vi "tvac_gui_chamber_workingcopy.vi"() -> ()   [LabVIEW 2017]
uses:
  Zones.ctl
  <vilib>/httpClient/ClientHandle.ctl
  msg7171_linux.llb/send single message.vi
  <vilib>/httpClient/POSTBuffer.vi
  <vilib>/Utility/file.llb/Read Delimited Spreadsheet (string).vi
  <vilib>/httpClient/LabVIEWHTTPClient.lvlib
panel:
  in  "tprofilesheet":string[][](array[string])
  in  "ThermalProfileCluster":T1
  out "body 2":string
  out "body":string
  in  "Custom Graph Selector":i32
  in  "exit":bool
  in  "AlarmColor":u32(colorbox)
  in  "Alarm String":string
  in  "Plot Color":u32(colorbox)=16860
  in  "Temperature":dbl format="%#_13g"
  in  "TC Label":string
  in  "Graph ON/OFF":u32(colorbox)=4250624
  in  "index (col)":i32
  in  "index (row)":i32
  out "working array":bool[](array[boolean])
  in  "Local Debug":bool
  in  "Tab Control":T2(tab)
  in  "Log/Linear Y-Axis":u16(ring) items=["Linear", "Log"]
  in  "Total Time":dbl
  in  "Set Time TC Graph":bool
  in  "Graphing Selection":u16(ring) items=["User Selection", "Graph All Thermocouples", "Clear Graph"]
  in  "Time Scale":u16(ring) items=["Minutes", "Hours", "Seconds"]
  out "Waveform Chart":waveform(dbl)[](graph)
  out "Thermocouples":T3(array[cluster])
  in  "Log/Linear Y-Axis 6":u16(ring) items=["Linear", "Log"]
  in  "Log/Linear Y-Axis 5":u16(ring) items=["Linear", "Log"]
  in  "Log/Linear Y-Axis 3":u16(ring) items=["Linear", "Log"]
  in  "Log/Linear Y-Axis 2":u16(ring) items=["Linear", "Log"]
  in  "Total Time 6":dbl
  in  "Set Time TC Graph 6":bool
  in  "Time Scale 6":u16(ring) items=["Minutes", "Hours", "Seconds"]
  in  "Total Time 5":dbl
  in  "Set Time TC Graph 5":bool
  in  "Time Scale 5":u16(ring) items=["Minutes", "Hours", "Seconds"]
  in  "Total Time 4":dbl
  in  "Set Time TC Graph 4":bool
  in  "Time Scale 4":u16(ring) items=["Minutes", "Hours", "Seconds"]
  in  "Total Time 3":dbl
  in  "Set Time TC Graph 3":bool
  in  "Time Scale 3":u16(ring) items=["Minutes", "Hours", "Seconds"]
  in  "Total Time 2":dbl
  in  "Set Time TC Graph 2":bool
  in  "Time Scale 2":u16(ring) items=["Minutes", "Hours", "Seconds"]
  in  "Log/Linear Y-Axis 1":u16(ring) items=["Linear", "Log"]
  in  "Total Time 1":dbl
  in  "Set Time TC Graph 1":bool
  in  "Time Scale 1":u16(ring) items=["Minutes", "Hours", "Seconds"]
  in  "Custom Chart 2 Selection":i32[](listbox)=[0]
  in  "Custom Chart 1 Selection":i32[](listbox)=[0]
  out "Custom Chart 1":waveform(dbl)[](graph)
  in  "Custom Chart 3 Selection":i32[](listbox)=[0]
  in  "Custom Chart 4 Selection":i32[](listbox)=[0]
  in  "Custom Chart 5 Selection":i32[](listbox)=[0]
  in  "Custom Chart 6 Selection":i32[](listbox)=[0]
  out "Custom Chart 2":waveform(dbl)[](graph)
  out "Custom Chart 3":waveform(dbl)[](graph)
  out "Custom Chart 4":waveform(dbl)[](graph)
  out "Custom Chart 5":waveform(dbl)[](graph)
  out "Custom Chart 6":waveform(dbl)[](graph)
  in  "Log/Linear Y-Axis 4":u16(ring) items=["Linear", "Log"]
  in  "Import Profile":bool
  out "Thermal Profile":dbl[](graph)
  out "Thermal Profile Event Status":string
  in  "CreateTProfile":T4(tab)
  in  "ZoneSetup":T5={"Number of Set points"=0.0, "Zone Selection"=[8], "Initiate Setup"=FALSE, "Thermal Profile Name"=""}
  in  "RampSoakTimes":cluster{"RampSoakTimes":dbl[][]}
  in  "Zone 1":T6={"Zone Thermocouples"=[0], "Temperature Calculation"=0, "Thermocouples Selected"="", "Temperature Goal"=[], "Max Allowable Temp"="", "Min Allowable Temp"=""} {"Temperature Calculation" items=["Average", "Minimum", "Maximum"]}
  in  "Zone 2":T6={"Zone Thermocouples"=[0], "Temperature Calculation"=0, "Thermocouples Selected"="", "Temperature Goal"=[], "Max Allowable Temp"="", "Min Allowable Temp"=""} {"Temperature Calculation" items=["Average", "Minimum", "Maximum"]}
  in  "Zone 3":T6={"Zone Thermocouples"=[0], "Temperature Calculation"=0, "Thermocouples Selected"="", "Temperature Goal"=[], "Max Allowable Temp"="", "Min Allowable Temp"=""} {"Temperature Calculation" items=["Average", "Minimum", "Maximum"]}
  in  "Zone 4":T6={"Zone Thermocouples"=[0], "Temperature Calculation"=0, "Thermocouples Selected"="", "Temperature Goal"=[], "Max Allowable Temp"="", "Min Allowable Temp"=""} {"Temperature Calculation" items=["Average", "Minimum", "Maximum"]}
  in  "Zone 5":T6={"Zone Thermocouples"=[0], "Temperature Calculation"=0, "Thermocouples Selected"="", "Temperature Goal"=[], "Max Allowable Temp"="", "Min Allowable Temp"=""} {"Temperature Calculation" items=["Average", "Minimum", "Maximum"]}
  in  "Zone 6":T6={"Zone Thermocouples"=[0], "Temperature Calculation"=0, "Thermocouples Selected"="", "Temperature Goal"=[], "Max Allowable Temp"="", "Min Allowable Temp"=""} {"Temperature Calculation" items=["Average", "Minimum", "Maximum"]}
  in  "Zone 7":T6={"Zone Thermocouples"=[0], "Temperature Calculation"=0, "Thermocouples Selected"="", "Temperature Goal"=[], "Max Allowable Temp"="", "Min Allowable Temp"=""} {"Temperature Calculation" items=["Average", "Minimum", "Maximum"]}
  in  "Zone 8":T6={"Zone Thermocouples"=[0], "Temperature Calculation"=0, "Thermocouples Selected"="", "Temperature Goal"=[], "Max Allowable Temp"="", "Min Allowable Temp"=""} {"Temperature Calculation" items=["Average", "Minimum", "Maximum"]}
  in  "Zone 9":T6={"Zone Thermocouples"=[0], "Temperature Calculation"=0, "Thermocouples Selected"="", "Temperature Goal"=[], "Max Allowable Temp"="", "Min Allowable Temp"=""} {"Temperature Calculation" items=["Average", "Minimum", "Maximum"]}
  in  "Save as CSV":bool
  in  "Load Into Database":bool
  in  "Compile Profile":bool
  in  "Run Profile":bool
  in  "Resume Profile":bool
  in  "Stop Profile":bool
  in  "Pause Profile":bool
  in  "Hold Profile":bool
  in  "Path":path
  in  "Tab Control 2":enum32{"Current", "History"}(tab)
  in  "Current Errors (click to clear)":i32(listbox)
  in  "Error History":i32(listbox)
  in  "TCs On":bool=TRUE
  in  "Pressure On":bool=TRUE
  in  "MCC On":bool=TRUE
  in  "ZoneTemps On":bool=TRUE
  in  "Compressor On":bool
  in  "Generate Error":bool
  out "errortrue":bool
  # "Set Pt #"
  # "Ramp Time (s)"
  # "Soak Time (s)"
  # "Set Pt #"
  # "Goal Temp (K)"
  # "Set Pt #"
  # "Goal Temp (K)"
  # "Set Pt #"
  # "Goal Temp (K)"
  # "Set Pt #"
  # "Goal Temp (K)"
  # "Set Pt #"
  # "Goal Temp (K)"
  # "Set Pt #"
  # "Goal Temp (K)"
  # "Set Pt #"
  # "Goal Temp (K)"
  # "Set Pt #"
  # "Goal Temp (K)"
  # "Set Pt #"
  # "Goal Temp (K)"
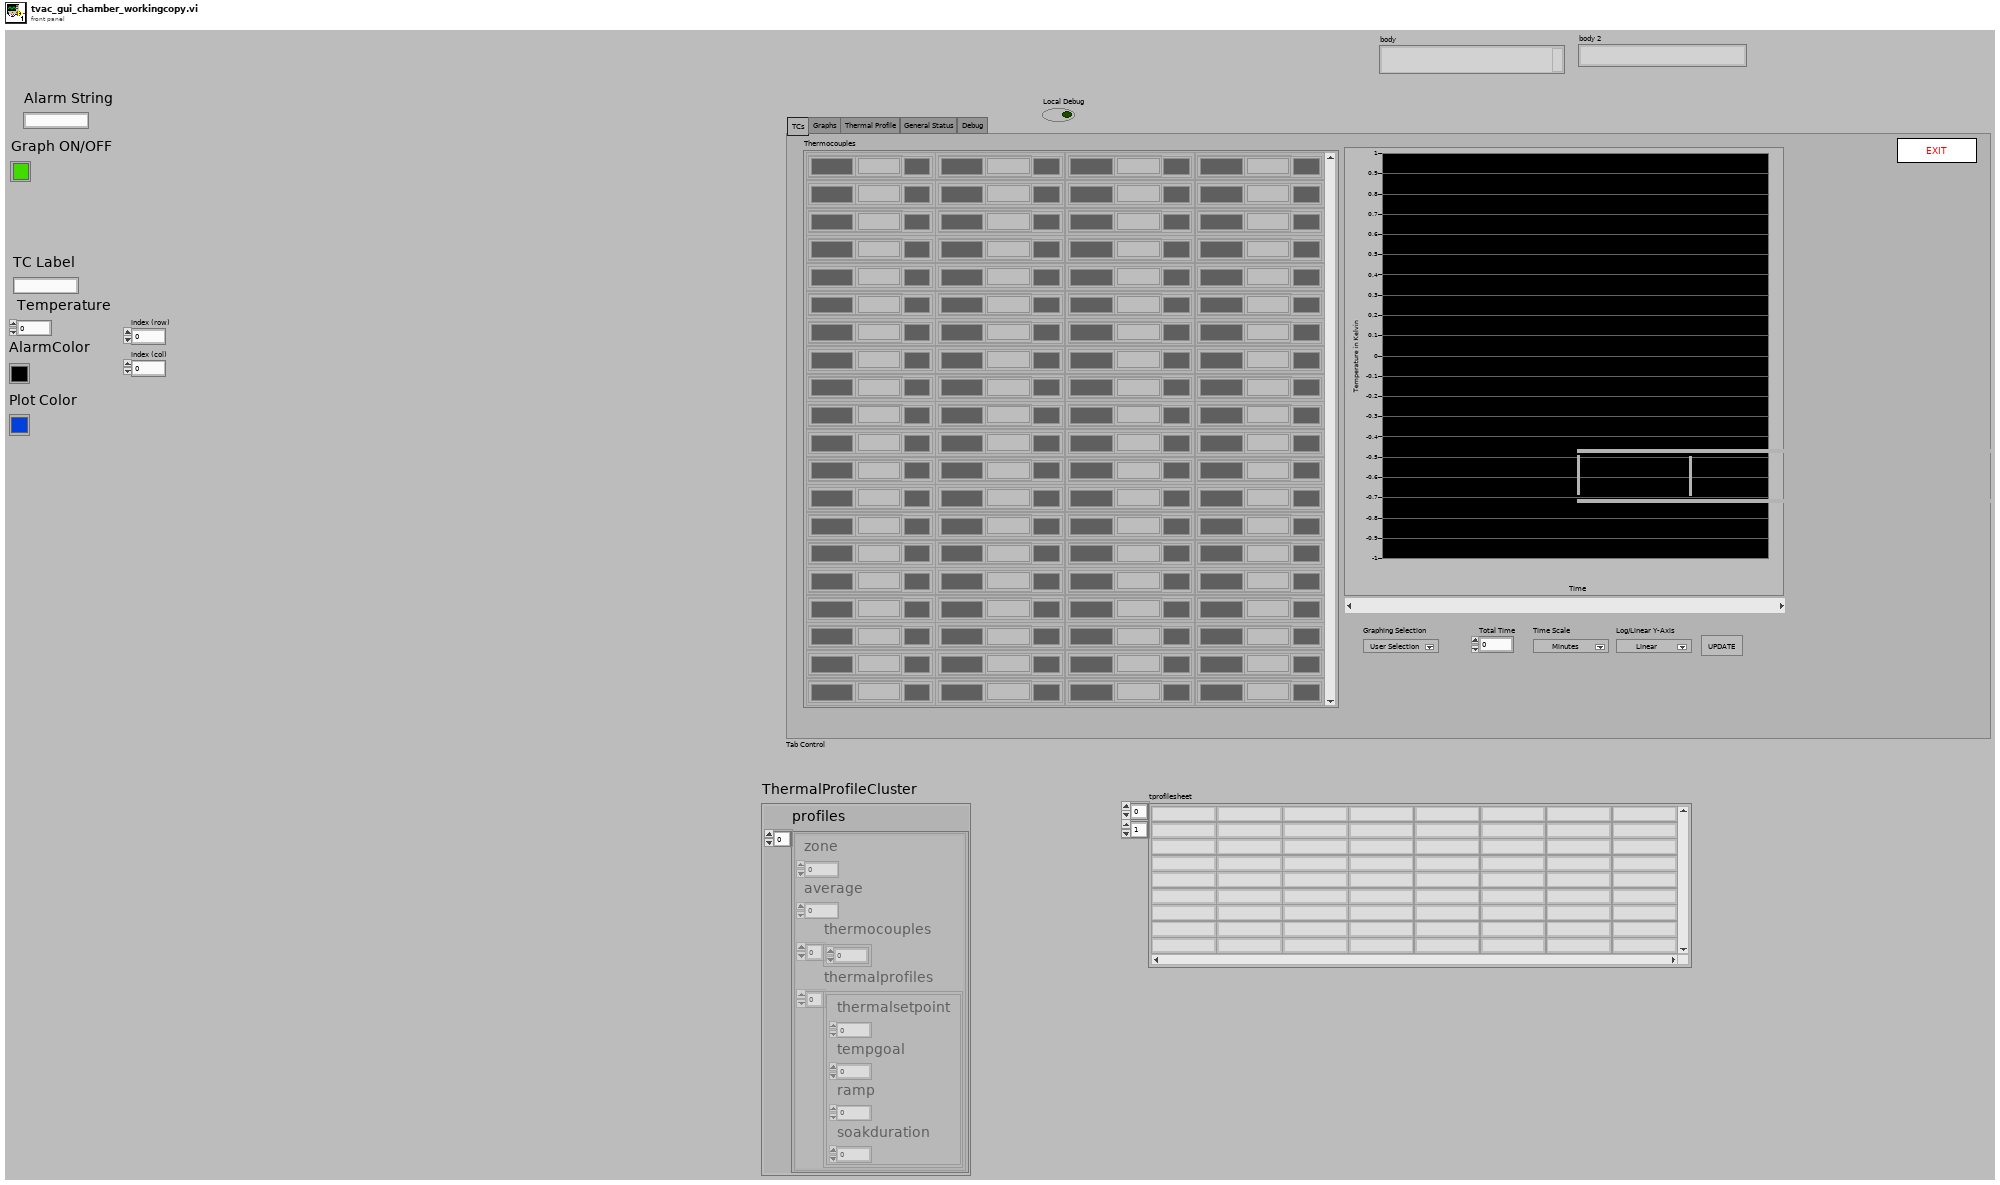
[diagram p1: front panel]
types:
  T1 = cluster{"profiles":cluster{"zone":i32, "average":i32, "thermocouples":i32[], "thermalprofiles":cluster{"thermalsetpoint":i32, "tempgoal":i32, "ramp":i32, "soakduration":i32}[]}[]}
  T2 = enum32{"TCs", "Graphs", "Thermal Profile", "General Status", "Debug"}
  T3 = cluster{"TC Label":string, "Alarm Status":string, "Alarm Color":u32, "Temperature":string, "PlotColor":u32, "Graph On/Off":u32}[][]
  T4 = enum32{"Setup", "Setup 2", "Zone 1", "Zone 2", "Zone 3", "Zone 4", "Zone 5", "Zone 6", "Zone 7", "Zone 8", "Zone 9", "Preview Profile"}
  T5 = cluster{"Number of Set points":dbl, "Zone Selection":i32[], "Initiate Setup":bool, "Thermal Profile Name":string}
  T6 = typedef "Zones.ctl" = cluster{"Zone Thermocouples":i32[], "Temperature Calculation":u16, "Thermocouples Selected":string, "Temperature Goal":dbl[][], "Max Allowable Temp":string, "Min Allowable Temp":string}
  T7 = cluster{"thermocouple":i32, "time":dbl, "temp":dbl, "working":bool, "alarm":i32}[]
  T8 = cluster{"Cp Stage 1 Temp":dbl[], "Cp Stage 2 Temp":dbl[]}
  T9 = typedef "LabVIEWHTTPClient.lvlib/ClientHandle.ctl" = refnum<k1>
  T10 = cluster{"ZoneSetup":cluster{"Number of Set points":dbl, "Zone Selection":i32[], "Initiate Setup":bool, "Thermal Profile Name":string}, "go":bool, "Http session":T9, "URL prefex":string, "index (row)":i32, "index (col)":i32, "Graph ON/OFF":u32, "TC Label":string, "Temperature":dbl, "AlarmColor":u32, "Plot Color":u32, "Alarm String":string, "Thermocouples":cluster{"TC Label":string, "Alarm Status":string, "Alarm Color":u32, "Temperature":string, "PlotColor":u32, "Graph On/Off":u32}[][], "working array":bool[], "i":i32, "NumberTCs":i32, "Waveform Chart":waveform(dbl)[], "Custom Chart 1":waveform(dbl)[], "Pressure":dbl[], "numSensors":i32, "Database":dbl[], "PumpTemps":cluster{"Cp Stage 1 Temp":dbl[], "Cp Stage 2 Temp":dbl[]}, "Zones":dbl[], "Time":i32, "TCs":cluster{"thermocouple":i32, "time":dbl, "temp":dbl, "working":bool, "alarm":i32}[], "ZoneTemps":cluster{"ZoneTemps":dbl[]}, "Compressor":cluster{"CompressorTemp":dbl}, "ErrorArray":string[][], "PrevErrorArray":string[][], "tprofilesheet":string[][], "Zone 1":T6, "ThermalProfileCluster":cluster{"profiles":cluster{"zone":i32, "average":i32, "thermocouples":i32[], "thermalprofiles":cluster{"thermalsetpoint":i32, "tempgoal":i32, "ramp":i32, "soakduration":i32}[]}[]}, "ZonesSelected":bool[], "Zone 2":T6, "Zone 3":T6, "Zone 4":T6, "Zone 5":T6, "Zone 6":T6, "Zone 7":T6, "Zone 8":T6, "Zone 9":T6}
  T11 = cluster{"TC Label":string, "Alarm Status":string, "Alarm Color":u32, "Temperature":string, "PlotColor":u32, "Graph On/Off":u32}
  T12 = enum32{"TCs", "Graphs", "Thermal Profile", "General Status"}
  T13 = cluster{"zone":i32, "average":i32, "thermocouples":i32[], "thermalprofiles":cluster{"thermalsetpoint":i32, "tempgoal":i32, "ramp":i32, "soakduration":i32}[]}
  T14 = cluster{"thermalsetpoint":i32, "tempgoal":i32, "ramp":i32, "soakduration":i32}
  T15 = cluster{"DutyCycle":i32, "Stage1Temp":i32, "CryoPumpReadyState":cluster{"MotorOn":bool, "Ready":bool}, "PurgeValveState":bool, "RegenError":string, "RegenStep":string, "RoughingValveState":bool, "RoughingInterlock":cluster{"RoughingPermission":bool, "RoughingNeeded":bool, "Cryopumprunning":bool}, "Stage2Temp":i32, "Status":cluster{"PumpOn":bool, "RoughOpen":bool, "PurgeOpen":bool, "ThermocoupleGaugeOn":bool, "PowerFailureOccurred":bool}, "TcPressure":i32}
  T16 = cluster{"time":string[], "event":string[], "Thermocouple":i32[], "details":string[], "actions":string[][]}
  T17 = cluster{"CryoPressure":dbl, "ChamberPressure":dbl, "RoughingPressure":dbl}
  T18 = cluster{"time":string, "TCs":cluster{"thermocouple":i32, "time":dbl, "temp":dbl, "working":bool, "alarm":i32}[]}
  T19 = typedef "LVPositionTypeDef.ctl" = cluster{"Left":i32, "Top":i32}
  T20 = typedef "LVPoint32TypeDef.ctl" = cluster{"Horizontal":i32, "Vertical":i32}
  T21 = typedef "LVRangeTypeDef.ctl" = cluster{"Minimum":dbl, "Maximum":dbl, "Increment":dbl, "Minor Increment":dbl, "Start":dbl}
  T22 = typedef "LVRowAndColumnTypeDef.ctl" = cluster{"Row":i32, "Column":i32}
  T23 = cluster{"zone":i32, "average":i32, "thermocouples":i32[], "thermalprofiles":cluster{"thermalsetpoint":i32, "tempgoal":i32, "ramp":i32, "soakduration":i32}[]}[]
  T24 = cluster{"thermalsetpoint":i32, "tempgoal":i32, "ramp":i32, "soakduration":i32}[]
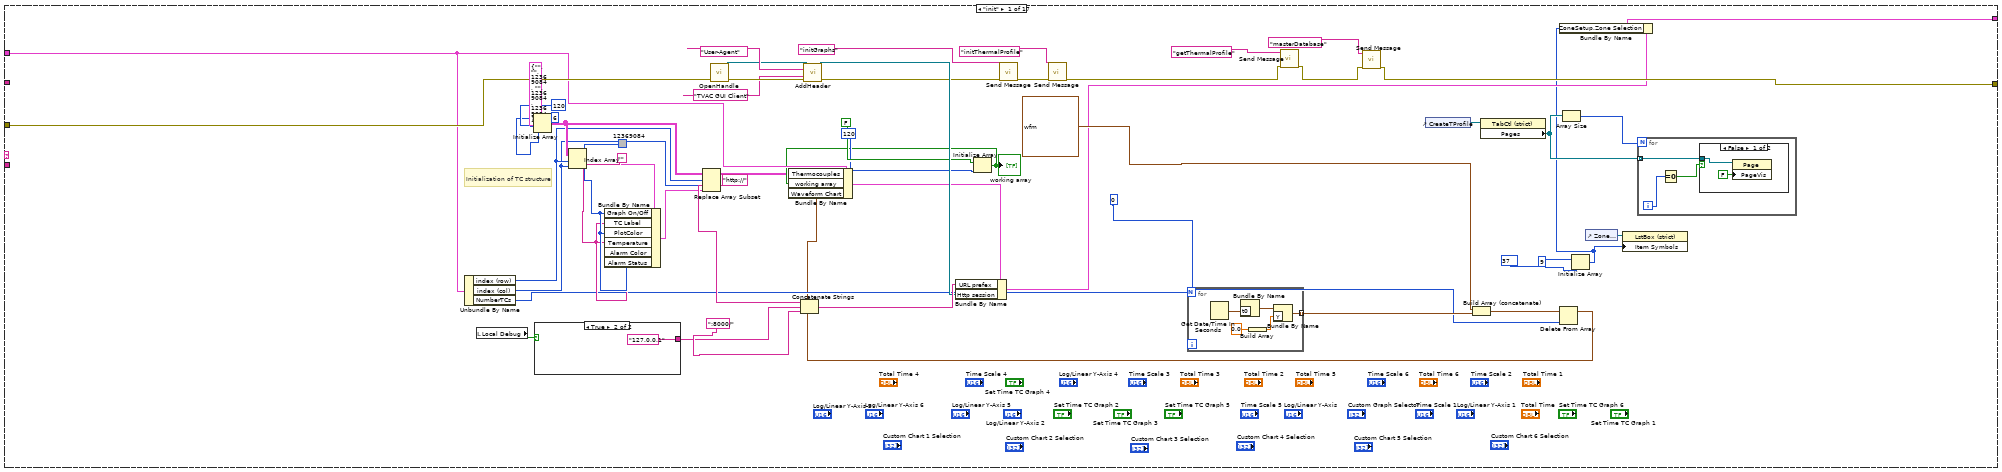
[diagram p2: hidden frame]
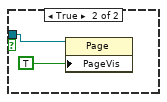
[diagram p3: hidden frame]
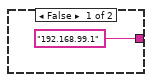
[diagram p4: hidden frame]
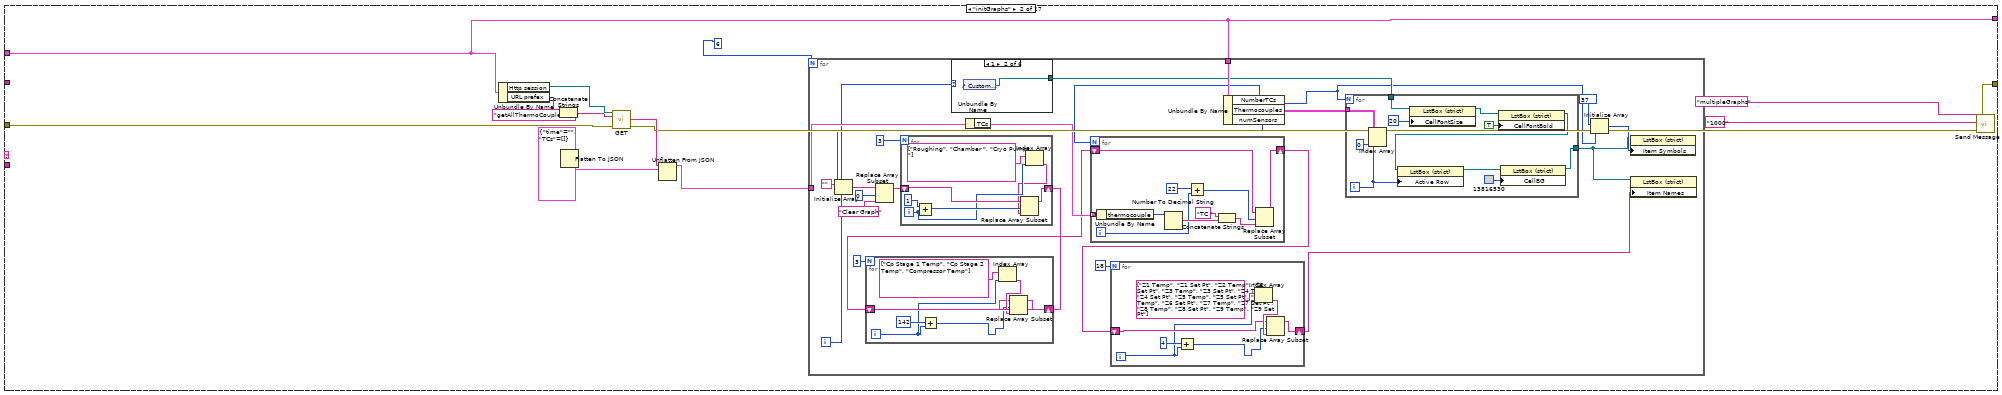
[diagram p5: hidden frame]
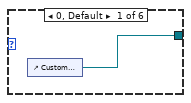
[diagram p6: hidden frame]
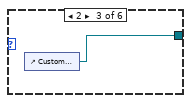
[diagram p7: hidden frame]
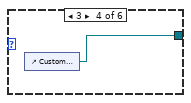
[diagram p8: hidden frame]
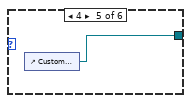
[diagram p9: hidden frame]
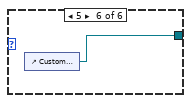
[diagram p10: hidden frame]
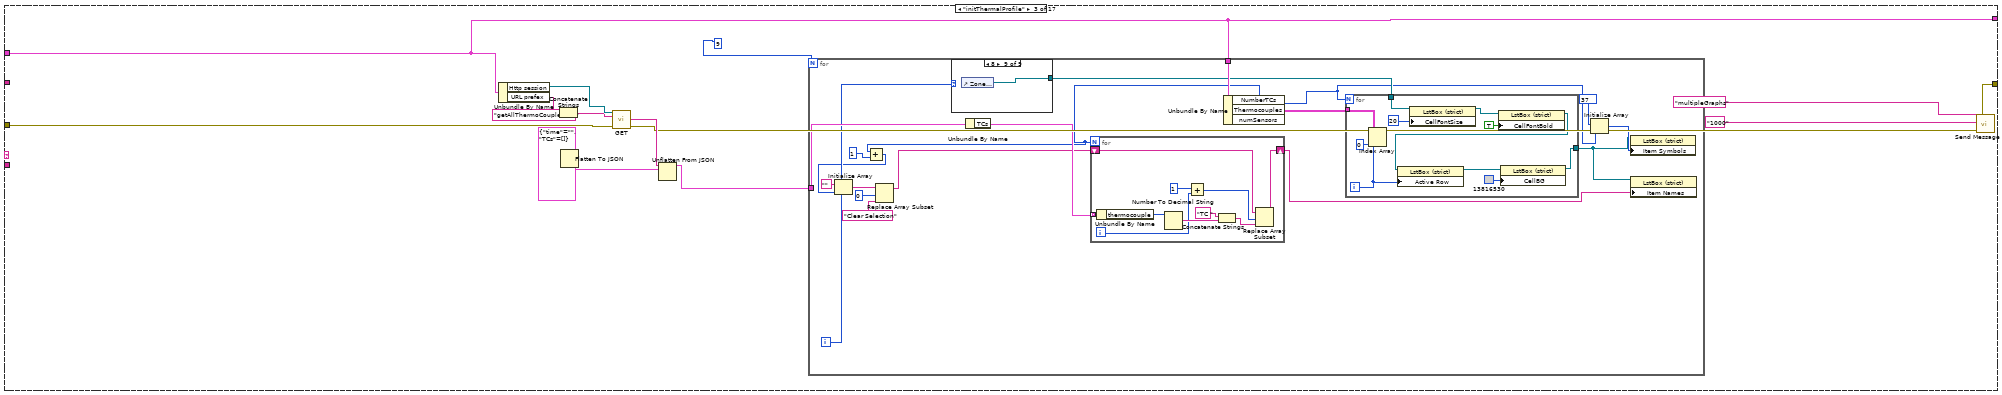
[diagram p11: hidden frame]
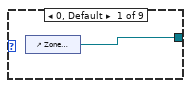
[diagram p12: hidden frame]
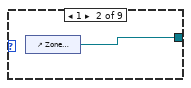
[diagram p13: hidden frame]
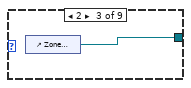
[diagram p14: hidden frame]
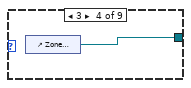
[diagram p15: hidden frame]
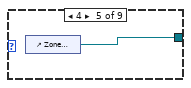
[diagram p16: hidden frame]
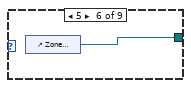
[diagram p17: hidden frame]
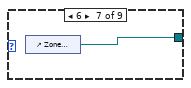
[diagram p18: hidden frame]
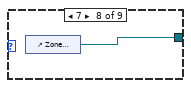
[diagram p19: hidden frame]
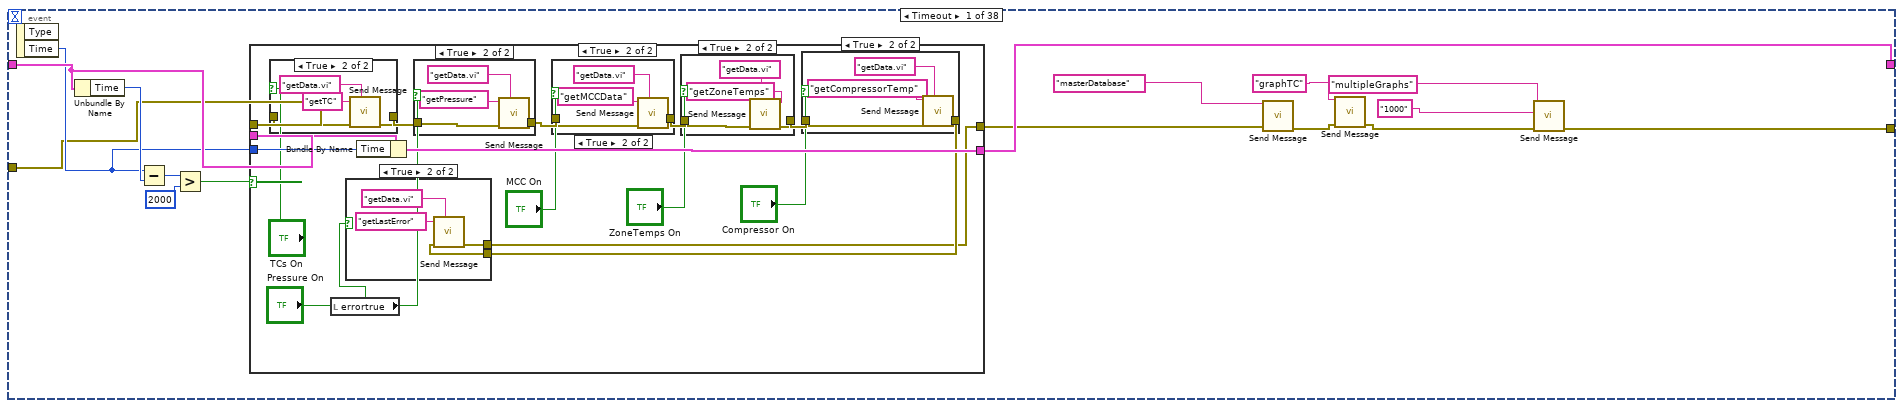
[diagram p20: hidden frame]
diagram:
  w9 = bool[] [FALSE, FALSE, FALSE, FALSE, FALSE, FALSE, FALSE, FALSE, FALSE]  # ZonesSelected
  w14 = string[][] []  # PrevErrorArray
  w15 = string[][] []  # ErrorArray
  w18 = cluster{"ZoneTemps":dbl[]} {"ZoneTemps"=[]}  # ZoneTemps
  w21 = dbl[] [24.54828257301887, 25.0, 20.035959453954195, 26.0, 28.926820041278148, 27.0, 21.321976066931608, 28.0, 29.197600688359813, 29.0, 29.117373424110085, 30.0, 21.092914485312942, 31.0, 27.791581465649088, 32.0, 24.70861457288988, 33.0]  # Zones
  w22 = T8 {"Cp Stage 1 Temp"=[0.0], "Cp Stage 2 Temp"=[0.0]}  # PumpTemps
  w23 = dbl[] [0.0, 1000.5841582194602, 1000.5841582194602, 1000.5841582194602, 0.6389895835935778, 0.7578061575842531, 1.153531014677555, 1.4572061556343079, 1.0192558642672256, 0.9245021790184325, 0.34311035179988925, 1.1970333160202968, 1.066989851322369, 0.5926593131154867, 0.7219240511326698, 1.0529790116491695, 1.4485694746891444, 0.9139060201605569, 0.7997359753068659, 0.6568795179977746, 0.8470104541419833, 1.0272585161866683, 0.6577301535824354, 0.645139941938139, 1.5235316442408067, 0.5128651184775285, 1.6421980587090137, 1.3961508335147417, 1.1242639015795428, 1.5954313466624428, 1.1919135255187876, 1.2615004458206727, 1.1320092264321664, 1.922759836270222, 1.1315561200367314, 1.4924621723754858, 0.6988771274186227, 1.069709701591943, 0.9920698240997152, 0.5395549253287656, 0.42891479657680576, 1.2794224940227927, 0.2687949632437338, 0.16127136772755854, 1.0174597006256374, 1.2079238230365172, 0.9745554383837218, 1.5348516925460962, 0.9488878852839246, 1.6634477658652282, 1.1924291951744272, 1.2231949298067308, 1.2223766746774598, 1.30664154589907, 1.2872878364107239, 0.5274250065177812, 0.7905999067114673, 1.2748974665085449, 1.216972941585413, 0.959115576325391, 0.5743502840762814, 0.8219540421676025, 0.613053899308251, 1.3785560870413707, 1.034117232127813, 1.1237698659753859, 1.4495548642149667, 0.6967905980938514, 0.6224497255665377, 1.6551326273040576, 1.2103048396824558, 0.6078721016951973, 1.3790669246280296, 0.5454332940871525, 1.5318777012492035, 1.2496539590411258, 0.9145395304446965, 1.3855381787793546, 1.0857600342029163, 1.3185833631438346, 0.9769688683142593, 1.026663691242448, 0.6744610422623843, 1.1965175398567691, 0.4847084945450119, 0.6435799980029115, 0.8079659363810663, 0.9130053929540112, 0.5271098423006861, 0.8088111736464799, 1.1455315536576556, 1.139809531926708, 1.5840192673434794, 1.0296748968089129, 1.7370669751200136, 1.3715484550405317, 0.3362063953932494, 1.0385868418202253, 1.4947740276021626, 1.0393600693910505, 0.8870410800672984, 1.2470388696569872, 0.9846724980375481, 0.9952471377109308, 1.0807485178906029, 1.1016630607035562, 1.3301039036808464, 0.8856852816151205, 0.4719509873120426, 0.5191430277856135, 0.12135113366044793, 0.4230478635224125, 1.1140562049976255, 1.5484968368781251, 1.1999891199114734, 1.8721302183420216, 1.071489235222563, 0.6260864330445979, 1.0305668002030492, 1.0223711899566386, 0.7842533472819472, 1.7301290335750898, 1.318694748426881, 0.6978662965493679]  # Database
  w25 = dbl[] [0.0, 0.0, 0.0]  # Pressure
  w45 = ""  # URL prefex
  w46 = T9 refnum  # Http session
  w47 = TRUE  # go
  n1 = call "Register Module.vi"() -> ("error out"=w43:errorcluster)  [unwired: 10 in, 1 out]
  n2 = call-poly "Send Message.vi"("error in (no error)"=w43, "event"="init") -> ("error out"=w42:errorcluster)  [unwired: 9 in]
  n3 = local read "Waveform Chart"() -> (w29:waveform(dbl)[])
  n4 = local read "Thermocouples"() -> (w27:T3)
  n5 = local read "Custom Chart 1"() -> (w26:waveform(dbl)[])
  n6 = Bundle("ZoneSetup"="ZoneSetup", "go"=w47, "Http session"=w46, "URL prefex"=w45, "index (row)"="index (row)", "index (col)"="index (col)", "Graph ON/OFF"="Graph ON/OFF", "TC Label"="TC Label", "Temperature"="Temperature", "AlarmColor"="AlarmColor", "Plot Color"="Plot Color", "Alarm String"="Alarm String", "Thermocouples"=w27, "working array"=bool[] [TRUE, TRUE, TRUE, TRUE, TRUE, TRUE, TRUE, TRUE, TRUE, TRUE, TRUE, TRUE, TRUE, TRUE, TRUE, TRUE, TRUE, TRUE, TRUE, TRUE, TRUE, TRUE, TRUE, TRUE, TRUE, TRUE, TRUE, TRUE, TRUE, TRUE, TRUE, TRUE, TRUE, TRUE, TRUE, TRUE, TRUE, TRUE, TRUE, TRUE, TRUE, TRUE, TRUE, TRUE, TRUE, TRUE, TRUE, TRUE, TRUE, TRUE, TRUE, TRUE, TRUE, TRUE, TRUE, TRUE, TRUE, TRUE, TRUE, TRUE, TRUE, TRUE, TRUE, TRUE, TRUE, TRUE, TRUE, TRUE, TRUE, TRUE, TRUE, TRUE, TRUE, TRUE, TRUE, TRUE, TRUE, TRUE, TRUE, TRUE, TRUE, TRUE, TRUE, TRUE, TRUE, TRUE, TRUE, TRUE, TRUE, TRUE, TRUE, TRUE, TRUE, TRUE, TRUE, TRUE, TRUE, TRUE, TRUE, TRUE, TRUE, TRUE, TRUE, TRUE, TRUE, TRUE, TRUE, TRUE, TRUE, TRUE, TRUE, TRUE, TRUE, TRUE, TRUE, TRUE, TRUE, TRUE, TRUE, TRUE], "i"=0, "NumberTCs"=120, "Waveform Chart"=w29, "Custom Chart 1"=w26, "Pressure"=w25, "numSensors"=145, "Database"=w23, "PumpTemps"=w22, "Zones"=w21, "Time"=0, "TCs"=T7 [], "ZoneTemps"=w18, "Compressor"=cluster{"CompressorTemp":dbl} {"CompressorTemp"=0.0}, "ErrorArray"=w15, "PrevErrorArray"=w14, "tprofilesheet"="tprofilesheet", "Zone 1"="Zone 1", "ThermalProfileCluster"="ThermalProfileCluster", "ZonesSelected"=w9, "Zone 2"="Zone 2", "Zone 3"="Zone 3", "Zone 4"="Zone 4", "Zone 5"="Zone 5", "Zone 6"="Zone 6", "Zone 7"="Zone 7", "Zone 8"="Zone 8", "Zone 9"="Zone 9") -> (w33:T10)  [unwired: 1 in]
  n7 = while {
    shift-left: w33 -> [w52]
    shift-right: [w49] -> _
    shift-right: [w50] -> w28
    shift-left: w42 -> [w57]
    stop <- w48 continue-if-true
    n8 = call "Get Message.vi"("error in (no error)"=w57) -> ("error out"=w55:errorcluster, "event buffer"=w56:string, "event"=w54:string, "source"=w53:string)  [unwired: 7 in]
    n9 = case shown="\"\", \"Idle\"" w54 {
      selector: w54 -> [_ _ _ _ _ _ _ _ _ _ _ _ _ _ _ _ w2622]
      tunnel: [w60 w129 w214 w282 w1761 w1860 w2299 w2381 w2394 w2403 w2437 w2439 w2451 w2464 w2484 w2620 w2624] -> w49
      tunnel: w52 -> [w83 w129 w214 w283 w1763 w1863 w2304 w2380 w2393 w2398 w2438 w2443 w2450 w2465 w2484 w2616 w2624]
      tunnel: w56 -> [_ _ _ _ _ _ _ w2378 w2383 w2414 w2429 w2442 w2448 _ w2485 _ _]
      tunnel: w55 -> [w104 w128 w213 w272 w1766 w1896 w2294 w2379 w2384 w2400 w2430 w2440 w2449 w2470 _ w2619 w2623]
      tunnel: [w68 w124 w209 w271 w1766 w1896 w2294 w2379 w2384 w2400 w2430 w2440 w2449 w2470 _ w2618 w2621] -> w51
      tunnel: w53 -> [_ _ _ _ _ _ _ _ _ _ _ _ _ _ _ _ _]
      frame "init" {
        w88 = ""
        w89 = u32 12369084 ("PlotColor")
        # "Initialization of TC structure"
        n10 = Unbundle By Name(w83) -> ("index (row)"=w91:i32, "index (col)"=w90:i32, "NumberTCs"=w80:i32)
        n11 = local read "Local Debug"() -> (w96:bool)
        n12 = Initialize Array(T11 {"TC Label"="", "Alarm Status"="", "Alarm Color"=12369084, "Temperature"="", "PlotColor"=12369084, "Graph On/Off"=12369084}, 120 ("dimension size"), 6 ("dimension size")) -> (w92:T3)
        n13 = case shown="True" w96 {
          tunnel: ["192.168.99.1" ("Address") "127.0.0.1" ("Address")] -> w97
          frame False {
          }
          frame True {
          }
        }
        n14 = Index Array(array=w92, index (row)=w91, index (col)=w90) -> (element=w87:T11)
        n15 = Bundle By Name(cluster=w87, "Graph On/Off"=w89, "TC Label"=w88, "PlotColor"=w89, "Temperature"=w88, "Alarm Color"=w89, "Alarm Status"=w88) -> (w86:T11)
        n16 = Replace Array Subset(array=w92, new element=w86, index (row)=w91, index (col)=w90) -> (w74:T3)
        n17 = call <vilib>:"OpenHandle.vi"("error in (no error)"=w104) -> ("client handle out"=w105:T9, "error out"=w108:errorcluster)  [unwired: 13 in]
        n18 = Concatenate Strings("http://" ("url"), w97, ":8000/" ("url")) -> (w101:string)
        n19 = call <vilib>:"AddHeader.vi"("client handle"=w105, "header"="User-Agent", "value"="TVAC GUI Client", "error in (no error)"=w108) -> ("client handle out"=w100:T9, "error out"=w99:errorcluster)  [unwired: 10 in]
        n20 = Initialize Array(FALSE ("Boolean"), 120 ("dimension size")) -> (w81:bool[])
        "working array" <- w81
        n21 = call-poly "Send Message.vi"("error in (no error)"=w99, "event"="initGraphs") -> ("error out"=w73:errorcluster)  [unwired: 9 in]
        n22 = call-poly "Send Message.vi"("error in (no error)"=w73, "event"="initThermalProfile") -> ("error out"=w71:errorcluster)  [unwired: 9 in]
        n23 = for {
          N: w80 -> [_]
          tunnel: [w116] -> w78 mode=indexing
          n24 = Get Date/Time In Seconds() -> (seconds since 1Jan1904=w120:timestamp)
          n25 = Bundle By Name("t0"=w120) -> (w117:waveform(dbl))  [unwired: 1 in]
          n26 = Build Array(0.0) -> (w119:dbl[])
          n27 = Bundle By Name(cluster=w117, "Y"=w119) -> (w116:waveform(dbl))
        }
        n28 = call-poly "Send Message.vi"("error in (no error)"=w71, "event"="getThermalProfile") -> ("error out"=w69:errorcluster)  [unwired: 9 in]
        n29 = call-poly "Send Message.vi"("error in (no error)"=w69, "event"="masterDatabase") -> ("error out"=w68:errorcluster)  [unwired: 9 in]
        n30 = control-ref of="CreateTProfile"() -> (w66:refnum<vi>)
        n31 = Build Array (concatenate)(waveform(dbl) {"t0"=timestamp(0 s since 1904-01-01), "dt"=1.0, "Y"=[0.0]} ("element"), w78) -> (w79:waveform(dbl)[])
        n32 = property on="Property Node" class="TabCtl (strict)"(reference=w66) -> ("Pages"=w64:refnum<vi>[])  [unwired: 1 in, 2 out]
        n33 = Delete From Array(array=w79, index=0) -> (array with subset deleted=w77:waveform(dbl)[])  [unwired: 1 in, 1 out]
        n34 = Bundle By Name(cluster=w83, "Thermocouples"=w74, "working array"=w81, "Waveform Chart"=w77) -> (w82:T10)
        n35 = Bundle By Name(cluster=w82, "URL prefex"=w101, "Http session"=w100) -> (w61:T10)
        n36 = Array Size(array=w64) -> (size(s)=w65:i32)
        n37 = Initialize Array(37, 9 ("dimension size")) -> (w58:i32[])
        n38 = Bundle By Name(cluster=w61, "ZoneSetup.Zone Selection"=w58) -> (w60:T10)
        n39 = control-ref of="Zone Selection"() -> (w59:refnum<vi>)
        n40 = property class="LstBox (strict)"(reference=w59, "Item Symbols"=w58) -> ()  [unwired: 1 in, 2 out]
        n41 = for {
          N: w65 -> [_]
          tunnel: w64 -> [w109] mode=indexing
          i -> [w111]
          n42 = Equal To 0?(x=w111) -> (x = 0?=w110:bool)
          n43 = case shown="False" w110 {
            tunnel: w109 -> [w112 w114]
            frame False {
              n44 = property on="Property Node" class="Page"(reference=w112, "PageVis"=FALSE ("Page Visible")) -> ()  [unwired: 1 in, 2 out]
            }
            frame True {
              n45 = property on="Property Node" class="Page"(reference=w114, "PageVis"=TRUE ("Page Selector Visible")) -> ()  [unwired: 1 in, 2 out]
            }
          }
        }
      }
      frame "initGraphs" {
        w130 = T18 {"time"="", "TCs"=[]} ("Cluster")
        n46 = Unbundle By Name(w129) -> ("Http session"=w136:T9, "URL prefex"=w134:string)
        n47 = Concatenate Strings(w134, "getAllThermoCoupleData" ("url")) -> (w135:string)
        n48 = Flatten To JSON(anything=w130) -> ()  [unwired: 2 in, 2 out]
        n49 = call <vilib>:"GET.vi"("client handle"=w136, "url"=w135, "error in (no error)"=w128) -> ("body"=w132:string, "error out"=w125:errorcluster)  [unwired: 9 in, 2 out]
        n50 = Unflatten From JSON(JSON string=w132, type and defaults=w130) -> (value=w131:T18)  [unwired: 5 in, 1 out]
        n51 = for {
          N: 6 ("Numeric") -> [_]
          tunnel: w131 -> [w158]
          tunnel: w129 -> [w157]
          i -> [w140]
          n52 = case shown="1" w140 {
            tunnel: [w160 w161 w162 w163 w164 w165] -> w141
            frame 0, Default {
              n53 = control-ref of="Custom Chart 1 Selection"() -> (w160:refnum<vi>)
            }
            frame 1 {
              n54 = control-ref of="Custom Chart 2 Selection"() -> (w161:refnum<vi>)
            }
            frame 2 {
              n55 = control-ref of="Custom Chart 3 Selection"() -> (w162:refnum<vi>)
            }
            frame 3 {
              n56 = control-ref of="Custom Chart 4 Selection"() -> (w163:refnum<vi>)
            }
            frame 4 {
              n57 = control-ref of="Custom Chart 5 Selection"() -> (w164:refnum<vi>)
            }
            frame 5 {
              n58 = control-ref of="Custom Chart 6 Selection"() -> (w165:refnum<vi>)
            }
          }
          n59 = Unbundle By Name(w158) -> ("TCs"=w154:T7)
          n60 = Unbundle By Name(w157) -> ("NumberTCs"=w152:i32, "Thermocouples"=w159:T3, "numSensors"=w138:i32)
          n61 = Initialize Array("", w138) -> (w150:string[])
          n62 = Replace Array Subset(array=w150, new element="Clear Graph" ("new element/subarray"), index=0) -> (w147:string[])
          n63 = for {
            N: 3 -> [_]
            shift-right: [w185] -> w145
            shift-left: w147 -> [w186]
            i -> [w181]
            n64 = Add(x=1 ("index"), y=w181) -> (x+y=w183:i32)
            n65 = Index Array(array=string[] ["Roughing", "Chamber ", "Cryo Pump "], index=w181) -> (element=w180:string)
            n66 = Replace Array Subset(array=w186, new element=w180, index=w183) -> (w185:string[])
          }
          n67 = for {
            N: 3 -> [_]
            shift-right: [w176] -> w144
            shift-left: w145 -> [w177]
            i -> [w173]
            n68 = Add(x=142 ("index"), y=w173) -> (x+y=w174:i32)
            n69 = Index Array(array=string[] ["Cp Stage 1 Temp", "Cp Stage 2 Temp", "Compressor Temp"], index=w173) -> (element=w178:string)
            n70 = Replace Array Subset(array=w177, new element=w178, index=w174) -> (w176:string[])
          }
          n71 = for {
            N: w152 -> [_]
            tunnel: w154 -> [w193] mode=indexing
            shift-right: [w187] -> w137
            shift-left: w144 -> [w189]
            i -> [w191]
            n72 = Unbundle By Name(w193) -> ("thermocouple"=w194:i32)
            n73 = Number To Decimal String(number=w194) -> (decimal integer string=w196:string)  [unwired: 1 in]
            n74 = Add(x=22 ("index"), y=w191) -> (x+y=w190:i32)
            n75 = Concatenate Strings("TC " ("string"), w196) -> (w188:string)
            n76 = Replace Array Subset(array=w189, new element=w188, index=w190) -> (w187:string[])
          }
          n77 = for {
            N: 18 -> [_]
            shift-right: [w166] -> w143
            shift-left: w137 -> [w168]
            i -> [w167]
            n78 = Add(x=4 ("index"), y=w167) -> (x+y=w169:i32)
            n79 = Index Array(array=string[] ["Z1 Temp", "Z1 Set Pt", "Z2 Temp", "Z2 Set Pt", "Z3 Temp", "Z3 Set Pt", "Z4 Temp", "Z4 Set Pt", "Z5 Temp", "Z5 Set Pt", "Z6 Temp", "Z6 Set Pt", "Z7 Temp", "Z7 Set Pt", "Z8 Temp", "Z8 Set Pt", "Z9 Temp", "Z9 Set Pt"], index=w167) -> (element=w171:string)
            n80 = Replace Array Subset(array=w168, new element=w171, index=w169) -> (w166:string[])
          }
          n81 = for {
            N: w138 -> [_]
            tunnel: w159 -> [w207]
            tunnel: w141 -> [w201]
            tunnel: [w197] -> w139
            i -> [w204]
            n82 = Index Array(array=w207, index (row)=w204, index (col)=0 ("disabled index (col)")) -> ()  [unwired: 1 out]
            n83 = property on="Property Node" class="LstBox (strict)"(reference=w201, "CellFontSize"=u32 20 ("Active Row:Cell Font:Size")) -> (reference out=w200:refnum<vi>)  [unwired: 1 in, 1 out]
            n84 = property on="Property Node" class="LstBox (strict)"(reference=w200, "CellFontBold"=TRUE ("Active Row:Cell Font:Bold")) -> (reference out=w199:refnum<vi>)  [unwired: 1 in, 1 out]
            n85 = property on="Property Node" class="LstBox (strict)"(reference=w199, "Active Row"=w204) -> (reference out=w198:refnum<vi>)  [unwired: 1 in, 1 out]
            n86 = property on="Property Node" class="LstBox (strict)"(reference=w198, "CellBG"=u32 13816530 ("Active Row:Cell Background Color")) -> (reference out=w197:refnum<vi>)  [unwired: 1 in, 1 out]
          }
          n87 = Initialize Array(37, w138) -> (w155:i32[])
          n88 = property on="Property Node" class="LstBox (strict)"(reference=w139, "Item Symbols"=w155) -> ()  [unwired: 1 in, 2 out]
          n89 = property on="Property Node" class="LstBox (strict)"(reference=w139, "Item Names"=w143) -> ()  [unwired: 1 in, 2 out]
        }
        n90 = call-poly "Send Message.vi"("error in (no error)"=w125, "event buffer"="1000", "event"="multipleGraphs") -> ("error out"=w124:errorcluster)  [unwired: 8 in]
      }
      frame "initThermalProfile" {
        w215 = T18 {"time"="", "TCs"=[]} ("Cluster")
        n91 = Unbundle By Name(w214) -> ("Http session"=w221:T9, "URL prefex"=w219:string)
        n92 = Concatenate Strings(w219, "getAllThermoCoupleData" ("url")) -> (w220:string)
        n93 = Flatten To JSON(anything=w215) -> ()  [unwired: 2 in, 2 out]
        n94 = call <vilib>:"GET.vi"("client handle"=w221, "url"=w220, "error in (no error)"=w213) -> ("body"=w217:string, "error out"=w210:errorcluster)  [unwired: 9 in, 2 out]
        n95 = Unflatten From JSON(JSON string=w217, type and defaults=w215) -> (value=w216:T18)  [unwired: 5 in, 1 out]
        n96 = for {
          N: 9 ("Numeric") -> [_]
          tunnel: w216 -> [w239]
          tunnel: w214 -> [w238]
          i -> [w229]
          n97 = case shown="8" w229 {
            tunnel: [w241 w242 w243 w244 w245 w246 w247 w248 w249] -> w230
            frame 0, Default {
              n98 = control-ref of="Zone Thermocouples"() -> (w241:refnum<vi>)
            }
            frame 1 {
              n99 = control-ref of="Zone Thermocouples"() -> (w242:refnum<vi>)
            }
            frame 2 {
              n100 = control-ref of="Zone Thermocouples"() -> (w243:refnum<vi>)
            }
            frame 3 {
              n101 = control-ref of="Zone Thermocouples"() -> (w244:refnum<vi>)
            }
            frame 4 {
              n102 = control-ref of="Zone Thermocouples"() -> (w245:refnum<vi>)
            }
            frame 5 {
              n103 = control-ref of="Zone Thermocouples"() -> (w246:refnum<vi>)
            }
            frame 6 {
              n104 = control-ref of="Zone Thermocouples"() -> (w247:refnum<vi>)
            }
            frame 7 {
              n105 = control-ref of="Zone Thermocouples"() -> (w248:refnum<vi>)
            }
            frame 8 {
              n106 = control-ref of="Zone Thermocouples"() -> (w249:refnum<vi>)
            }
          }
          n107 = Unbundle By Name(w239) -> ("TCs"=w235:T7)
          n108 = Unbundle By Name(w238) -> ("NumberTCs"=w224:i32, "Thermocouples"=w240:T3, "numSensors"=w227:i32)
          n109 = Add(x=w224, y=1 ("index")) -> (x+y=w222:i32)
          n110 = Initialize Array("", w222) -> (w233:string[])
          n111 = Replace Array Subset(array=w233, new element="Clear Selection" ("new element/subarray"), index=0) -> (w226:string[])
          n112 = for {
            N: w224 -> [_]
            tunnel: w235 -> [w256] mode=indexing
            shift-right: [w250] -> w225
            shift-left: w226 -> [w252]
            i -> [w254]
            n113 = Unbundle By Name(w256) -> ("thermocouple"=w257:i32)
            n114 = Number To Decimal String(number=w257) -> (decimal integer string=w259:string)  [unwired: 1 in]
            n115 = Add(x=1 ("index"), y=w254) -> (x+y=w253:i32)
            n116 = Concatenate Strings("TC " ("string"), w259) -> (w251:string)
            n117 = Replace Array Subset(array=w252, new element=w251, index=w253) -> (w250:string[])
          }
          n118 = for {
            N: w227 -> [_]
            tunnel: w240 -> [w270]
            tunnel: w230 -> [w264]
            tunnel: [w260] -> w228
            i -> [w267]
            n119 = Index Array(array=w270, index (row)=w267, index (col)=0 ("disabled index (col)")) -> ()  [unwired: 1 out]
            n120 = property on="Property Node" class="LstBox (strict)"(reference=w264, "CellFontSize"=u32 20 ("Active Row:Cell Font:Size")) -> (reference out=w263:refnum<vi>)  [unwired: 1 in, 1 out]
            n121 = property on="Property Node" class="LstBox (strict)"(reference=w263, "CellFontBold"=TRUE ("Active Row:Cell Font:Bold")) -> (reference out=w262:refnum<vi>)  [unwired: 1 in, 1 out]
            n122 = property on="Property Node" class="LstBox (strict)"(reference=w262, "Active Row"=w267) -> (reference out=w261:refnum<vi>)  [unwired: 1 in, 1 out]
            n123 = property on="Property Node" class="LstBox (strict)"(reference=w261, "CellBG"=u32 13816530 ("Active Row:Cell Background Color")) -> (reference out=w260:refnum<vi>)  [unwired: 1 in, 1 out]
          }
          n124 = Initialize Array(37, w227) -> (w236:i32[])
          n125 = property on="Property Node" class="LstBox (strict)"(reference=w228, "Item Symbols"=w236) -> ()  [unwired: 1 in, 2 out]
          n126 = property on="Property Node" class="LstBox (strict)"(reference=w228, "Item Names"=w225) -> ()  [unwired: 1 in, 2 out]
        }
        n127 = call-poly "Send Message.vi"("error in (no error)"=w210, "event buffer"="1000", "event"="multipleGraphs") -> ("error out"=w209:errorcluster)  [unwired: 8 in]
      }
      frame "", "Idle" {
        n128 = control-ref of="Thermocouples"() -> (w281:refnum<vi>)
        n129 = property on="Property Node" class="Arr (strict)"(reference=w281) -> ("Position"=w280:T19)  [unwired: 1 in, 2 out]
        n130 = Unbundle By Name(w280) -> ("Left"=w279:i32, "Top"=w277:i32)
        n131 = Add(x=4, y=w279) -> (x+y=w275:i32)
        n132 = Add(x=w277, y=23 ("x")) -> (x+y=w274:i32)
        n133 = event shown="[26] \"Import Profile\": Value Change" {
          selector: _ -> [_ _ _ _ _ _ _ _ _ _ _ _ _ _ _ _ _ _ _ _ _ _ _ _ _ _ _ _ _ _ _ _ _ _ _ _ _ _]
          dyn-events: _ -> [_ _ _ _ _ _ _ _ _ _ _ _ _ _ _ _ _ _ _ _ _ _ _ _ _ _ _ _ _ _ _ _ _ _ _ _ _ _]
          timeout: 200 ("milliseconds to wait") -> [_ _ _ _ _ _ _ _ _ _ _ _ _ _ _ _ _ _ _ _ _ _ _ _ _ _ _ _ _ _ _ _ _ _ _ _ _ _]
          tunnel: [w299 w354 w363 w372 w381 w390 w399 w402 w418 w511 w575 w636 w697 w758 w819 w880 w941 w1010 w1011 w1017 w1023 w1029 w1039 w1046 w1069 w1096 w1180 w1264 w1270 w1324 w1378 w1432 w1486 w1540 w1594 w1648 w1702 w1752] -> w271
          tunnel: [w292 w356 w365 w374 w383 w392 w401 w407 w419 w505 w576 w637 w698 w759 w820 w881 w942 w1009 w1016 w1022 w1028 w1034 w1038 w1042 w1064 w1099 w1175 w1260 w1269 w1323 w1377 w1431 w1485 w1539 w1593 w1647 w1701 w1755] -> w282
          tunnel: w283 -> [w293 w356 w365 w374 w383 w392 w401 w407 w420 w507 w576 w637 w698 w759 w820 w881 w942 w1009 w1016 w1022 w1028 w1034 w1038 w1043 w1065 w1099 w1176 w1261 w1269 w1323 w1377 w1431 w1485 w1539 w1593 w1647 w1701 w1755]
          tunnel: w275 -> [_ _ _ _ _ _ _ _ w417 _ _ _ _ _ _ _ _ _ _ _ _ _ _ _ _ _ _ _ _ _ _ _ _ _ _ _ _ _]
          tunnel: w274 -> [_ _ _ _ _ _ _ _ w414 _ _ _ _ _ _ _ _ _ _ _ _ _ _ _ _ _ _ _ _ _ _ _ _ _ _ _ _ _]
          tunnel: w272 -> [w288 w355 w364 w373 w382 w391 w400 w403 w418 w511 w575 w636 w697 w758 w819 w880 w941 w1010 w1012 w1018 w1024 w1030 w1039 w1046 w1069 w1096 w1181 w1265 w1270 w1324 w1378 w1432 w1486 w1540 w1594 w1648 w1702 w1754]
          event Timeout {
            n134 = event-data() -> ("Time"=w291:u32)  [unwired: 1 in, 1 out]
            n135 = Unbundle By Name(w293) -> ("Time"=w296:i32)
            n136 = Subtract(x=w291, y=w296) -> (x-y=w295:u32)
            n137 = Greater?(x=w295, y=u32 2000 ("millisecond multiple")) -> (0:w284:bool)
            n138 = case shown="True" w284 {
              tunnel: w293 -> [w301 w317]
              tunnel: [w301 w316] -> w292
              tunnel: w291 -> [_ w315]
              tunnel: [w300 w308] -> w290
              tunnel: w288 -> [w300 w314]
              frame False {
              }
              frame True {
                n139 = case shown="True" "TCs On" {
                  tunnel: w314 -> [w318 w322]
                  tunnel: [w318 w320] -> w313
                  frame False {
                  }
                  frame True {
                    n140 = call-poly "Send Message.vi"("Destination Module"="getData.vi", "error in (no error)"=w322, "event"="getTC") -> ("error out"=w320:errorcluster)  [unwired: 8 in]
                  }
                }
                n141 = local read "errortrue"() -> (w307:bool)
                n142 = Bundle By Name(cluster=w317, "Time"=w315) -> (w316:T10)
                n143 = case shown="True" "Pressure On" {
                  tunnel: w313 -> [w338 w341]
                  tunnel: [w338 w339] -> w312
                  frame False {
                  }
                  frame True {
                    n144 = call-poly "Send Message.vi"("Destination Module"="getData.vi", "error in (no error)"=w341, "event"="getPressure") -> ("error out"=w339:errorcluster)  [unwired: 8 in]
                  }
                }
                n145 = case shown="True" "MCC On" {
                  tunnel: w312 -> [w333 w335]
                  tunnel: [w333 w334] -> w311
                  frame False {
                  }
                  frame True {
                    n146 = call-poly "Send Message.vi"("Destination Module"="getData.vi", "error in (no error)"=w335, "event"="getMCCData") -> ("error out"=w334:errorcluster)  [unwired: 8 in]
                  }
                }
                n147 = case shown="True" "ZoneTemps On" {
                  tunnel: w311 -> [w328 w332]
                  tunnel: [w328 w329] -> w310
                  frame False {
                  }
                  frame True {
                    n148 = call-poly "Send Message.vi"("Destination Module"="getData.vi", "error in (no error)"=w332, "event"="getZoneTemps") -> ("error out"=w329:errorcluster)  [unwired: 8 in]
                  }
                }
                n149 = case shown="True" "Compressor On" {
                  tunnel: w310 -> [w323 w325]
                  tunnel: [w323 w324] -> w309
                  frame False {
                  }
                  frame True {
                    n150 = call-poly "Send Message.vi"("Destination Module"="getData.vi", "error in (no error)"=w325, "event"="getCompressorTemp") -> ("error out"=w324:errorcluster)  [unwired: 8 in]
                  }
                }
                n151 = case shown="True" w307 {
                  tunnel: w309 -> [w343 w345]
                  tunnel: [w343 w344] -> w308
                  frame False {
                  }
                  frame True {
                    n152 = call-poly "Send Message.vi"("Destination Module"="getData.vi", "error in (no error)"=w345, "event"="getLastError") -> ("error out"=w344:errorcluster)  [unwired: 8 in]
                  }
                }
              }
            }
            n153 = call-poly "Send Message.vi"("error in (no error)"=w290, "event"="masterDatabase") -> ("error out"=w287:errorcluster)  [unwired: 9 in]
            n154 = call-poly "Send Message.vi"("error in (no error)"=w287, "event"="graphTC") -> ("error out"=w286:errorcluster)  [unwired: 9 in]
            n155 = call-poly "Send Message.vi"("error in (no error)"=w286, "event buffer"="1000", "event"="multipleGraphs") -> ("error out"=w299:errorcluster)  [unwired: 8 in]
          }
          event "Custom Chart 1 Selection": Mouse Down {
            n156 = event-data() -> ("CtlRef"=w350:refnum<vi>, "Coords"=w349:T20)  [unwired: 1 in, 6 out]
            n157 = invoke on="Invoke Node" class="LstBox (strict)" method="Point To Row"(reference=w350, "Point"=w349) -> ("Row"=w348:i32)  [unwired: 5 in, 6 out]
            n158 = local write "Custom Graph Selector"(0) -> ()
            n159 = Number To Decimal String(number=w348) -> (decimal integer string=w352:string)  [unwired: 1 in]
            n160 = call-poly "Send Message.vi"("error in (no error)"=w355, "event buffer"=w352, "event"="multipleGraphs") -> ("error out"=w354:errorcluster)  [unwired: 8 in]
          }
          event "Custom Chart 2 Selection": Mouse Down {
            n161 = event-data() -> ("CtlRef"=w359:refnum<vi>, "Coords"=w358:T20)  [unwired: 1 in, 6 out]
            n162 = invoke on="Invoke Node" class="LstBox (strict)" method="Point To Row"(reference=w359, "Point"=w358) -> ("Row"=w357:i32)  [unwired: 5 in, 6 out]
            n163 = local write "Custom Graph Selector"(1) -> ()
            n164 = Number To Decimal String(number=w357) -> (decimal integer string=w361:string)  [unwired: 1 in]
            n165 = call-poly "Send Message.vi"("error in (no error)"=w364, "event buffer"=w361, "event"="multipleGraphs") -> ("error out"=w363:errorcluster)  [unwired: 8 in]
          }
          event "Custom Chart 3 Selection": Mouse Down {
            n166 = event-data() -> ("CtlRef"=w368:refnum<vi>, "Coords"=w367:T20)  [unwired: 1 in, 6 out]
            n167 = invoke on="Invoke Node" class="LstBox (strict)" method="Point To Row"(reference=w368, "Point"=w367) -> ("Row"=w366:i32)  [unwired: 5 in, 6 out]
            n168 = local write "Custom Graph Selector"(2) -> ()
            n169 = Number To Decimal String(number=w366) -> (decimal integer string=w370:string)  [unwired: 1 in]
            n170 = call-poly "Send Message.vi"("error in (no error)"=w373, "event buffer"=w370, "event"="multipleGraphs") -> ("error out"=w372:errorcluster)  [unwired: 8 in]
          }
          event "Custom Chart 4 Selection": Mouse Down {
            n171 = event-data() -> ("CtlRef"=w377:refnum<vi>, "Coords"=w376:T20)  [unwired: 1 in, 6 out]
            n172 = invoke on="Invoke Node" class="LstBox (strict)" method="Point To Row"(reference=w377, "Point"=w376) -> ("Row"=w375:i32)  [unwired: 5 in, 6 out]
            n173 = local write "Custom Graph Selector"(3) -> ()
            n174 = Number To Decimal String(number=w375) -> (decimal integer string=w379:string)  [unwired: 1 in]
            n175 = call-poly "Send Message.vi"("error in (no error)"=w382, "event buffer"=w379, "event"="multipleGraphs") -> ("error out"=w381:errorcluster)  [unwired: 8 in]
          }
          event "Custom Chart 5 Selection": Mouse Down {
            n176 = event-data() -> ("CtlRef"=w386:refnum<vi>, "Coords"=w385:T20)  [unwired: 1 in, 6 out]
            n177 = invoke on="Invoke Node" class="LstBox (strict)" method="Point To Row"(reference=w386, "Point"=w385) -> ("Row"=w384:i32)  [unwired: 5 in, 6 out]
            n178 = local write "Custom Graph Selector"(4) -> ()
            n179 = Number To Decimal String(number=w384) -> (decimal integer string=w388:string)  [unwired: 1 in]
            n180 = call-poly "Send Message.vi"("error in (no error)"=w391, "event buffer"=w388, "event"="multipleGraphs") -> ("error out"=w390:errorcluster)  [unwired: 8 in]
          }
          event "Custom Chart 6 Selection": Mouse Down {
            n181 = event-data() -> ("CtlRef"=w395:refnum<vi>, "Coords"=w394:T20)  [unwired: 1 in, 6 out]
            n182 = invoke on="Invoke Node" class="LstBox (strict)" method="Point To Row"(reference=w395, "Point"=w394) -> ("Row"=w393:i32)  [unwired: 5 in, 6 out]
            n183 = local write "Custom Graph Selector"(5) -> ()
            n184 = Number To Decimal String(number=w393) -> (decimal integer string=w397:string)  [unwired: 1 in]
            n185 = call-poly "Send Message.vi"("error in (no error)"=w400, "event buffer"=w397, "event"="multipleGraphs") -> ("error out"=w399:errorcluster)  [unwired: 8 in]
          }
          event "Tab Control": Value Change {
            n186 = event-data() -> ("NewVal"=w406:T2)  [unwired: 1 in, 5 out]
            n187 = Equal?(x=w406, y=enum16{"Graphs"}."Graphs") -> (x = y?=w404:bool)
            n188 = case shown="True" w404 {
              tunnel: w403 -> [w408 w410]
              tunnel: [w408 w409] -> w402
              frame False {
              }
              frame True {
                n189 = call-poly "Send Message.vi"("error in (no error)"=w410, "event"="getGraphs") -> ("error out"=w409:errorcluster)  [unwired: 9 in]
              }
            }
          }
          event "Thermocouples": Mouse Down {
            n190 = event-data() -> ("CtlRef"=w422:refnum<vi>, "Coords"=w427:T20)  [unwired: 1 in, 3 out]
            n191 = Unbundle By Name(w427) -> ("Horizontal"=w425:i32, "Vertical"=w424:i32)
            n192 = Add(x=783 ("y"), y=w417) -> (x+y=w412:i32)
            n193 = Less?(x=w425, y=w412) -> (x < y?=w426:bool)
            n194 = Add(x=w414, y=854) -> (x+y=w413:i32)
            n195 = Less?(x=w424, y=w413) -> (x < y?=w423:bool)
            n196 = And(x=w426, y=w423) -> (x .and. y?=w421:bool)
            n197 = case shown="True" w421 {
              tunnel: w422 -> [_ w469]
              tunnel: w420 -> [_ w441]
              tunnel: w420 -> [w428 w439]
              tunnel: [w428 w431] -> w419
              tunnel: w417 -> [_ w430]
              tunnel: w414 -> [_ w429]
              frame False {
              }
              frame True {
                w463 = u16 0 items=["User Selection", "Graph All Thermocouples", "Clear Graph"] ("Graphing Selection")
                n198 = property class="Arr (strict)"(reference=w469) -> ("Array Element.Position"=w461:T19)  [unwired: 1 in, 2 out]
                n199 = local write "Graphing Selection"(w463) -> ()
                n200 = Unbundle By Name(w461) -> ("Left"=w459:i32, "Top"=w462:i32)
                n201 = property on="Thermocouples" class="Arr (strict)"() -> ("Index Values"=w453:u32[])  [unwired: 2 in, 2 out]
                n202 = Subtract(x=w430, y=w459) -> (x-y=w458:i32)
                n203 = Subtract(x=w429, y=w462) -> (x-y=w450:i32)
                n204 = Absolute Value(x=w450) -> (abs(x)=w460:i32)
                n205 = Index Array(array=w453, index=0) -> (element=w449:u32)
                n206 = To Byte Integer(number=w449) -> (8bit integer=w448:i8)
                n207 = Absolute Value(x=w458) -> (abs(x)=w457:i32)
                n208 = local read "Thermocouples"() -> (w432:T3)
                n209 = Quotient & Remainder(x=w460, y=42) -> (floor(x/y)=w447:i32)  [unwired: 1 out]
                n210 = Add(x=w448, y=w447) -> (x+y=w434:i32)
                n211 = Quotient & Remainder(x=w457, y=197 ("Numeric 2")) -> (floor(x/y)=w433:i32)  [unwired: 1 out]
                n212 = Index Array(array=w432, index (row)=w434, index (col)=w433) -> (element=w435:T11)
                n213 = Multiply(x=4, y=w434) -> (x*y=w454:i32)
                n214 = Unbundle By Name(w441) -> ("working array"=w440:bool[])  [unwired: 1 out]
                n215 = Unbundle By Name(w435) -> ("Alarm Color"=w467:u32, "Graph On/Off"=w466:u32, "TC Label"=w465:string, "PlotColor"=w446:u32, "Alarm Status"=w464:string, "Temperature"=w437:string)
                n216 = Add(x=w454, y=w433) -> (x+y=w443:i32)
                n217 = control-ref of="Waveform Chart"() -> (w468:refnum<vi>)
                n218 = Index Array(array=w440, index=w443) -> (element=w442:bool)
                n219 = Decimal String To Number(string=w437) -> ()  [unwired: 2 in, 2 out]
                n220 = Equal?(x=w466, y=u32 12369084) -> (x = y?=w444:bool)
                n221 = case shown="True" w442 {
                  selector: w442 -> [_ w475]
                  tunnel: w468 -> [_ w481]
                  tunnel: w467 -> [_ w480]
                  tunnel: w465 -> [_ w479]
                  tunnel: w464 -> [_ w478]
                  tunnel: w443 -> [_ w471]
                  tunnel: w446 -> [_ w477]
                  tunnel: w444 -> [_ w476]
                  tunnel: w437 -> [_ w474]
                  tunnel: [w470 w473] -> w436
                  tunnel: w435 -> [w470 w472]
                  frame False {
                  }
                  frame True {
                    n222 = case shown="True" w476 {
                      tunnel: w481 -> [w491 w502]
                      tunnel: w480 -> [w485 w497]
                      tunnel: w479 -> [w486 w496]
                      tunnel: w478 -> [w487 w498]
                      tunnel: w477 -> [_ w500]
                      tunnel: w475 -> [_ _]
                      tunnel: w474 -> [w488 w499]
                      tunnel: [w483 w495] -> w473
                      tunnel: w472 -> [w484 w494]
                      tunnel: w471 -> [w482 w493]
                      frame False {
                        w489 = u32 12369084
                        n223 = property on="Property Node" class="WFChart (strict)"(reference=w491, "Active Plot"=w482) -> (reference out=w492:refnum<vi>)  [unwired: 1 in, 1 out]
                        n224 = Bundle By Name(cluster=w484, "Graph On/Off"=w489, "TC Label"=w486, "PlotColor"=w489, "Temperature"=w488, "Alarm Color"=w485, "Alarm Status"=w487) -> (w483:T11)
                        n225 = property class="WFChart (strict)"(reference=w492, "Plot.Visible?"=FALSE ("Plot.Visible")) -> ()  [unwired: 1 in, 2 out]
                      }
                      frame True {
                        n226 = property class="WFChart (strict)"(reference=w502, "Active Plot"=w493) -> (reference out=w503:refnum<vi>)  [unwired: 1 in, 1 out]
                        n227 = Bundle By Name(cluster=w494, "Graph On/Off"=u32 6618880, "TC Label"=w496, "PlotColor"=w500, "Temperature"=w499, "Alarm Color"=w497, "Alarm Status"=w498) -> (w495:T11)
                        n228 = property class="WFChart (strict)"(reference=w503, "Plot.Visible?"=TRUE ("Plot.Visible")) -> ()  [unwired: 1 in, 2 out]
                      }
                    }
                  }
                }
                n229 = Replace Array Subset(array=w432, new element=w436, index (row)=w434, index (col)=w433) -> (w438:T3)
                n230 = Bundle By Name(cluster=w439, "Thermocouples"=w438) -> (w431:T10)
              }
            }
          }
          event "Graphing Selection": Value Change {
            n231 = event-data() -> ("NewVal"=w512:u16)  [unwired: 1 in, 5 out]
            n232 = Unbundle By Name(w507) -> ("Thermocouples"=w506:T3, "working array"=w509:bool[])
            n233 = control-ref of="Waveform Chart"() -> (w513:refnum<vi>)
            n234 = case shown="1" w512 {
              tunnel: w506 -> [w514 w519 w550]
              tunnel: w513 -> [_ w518 w549]
              tunnel: 120 ("disabled index (col)") -> [_ w517 w548]
              tunnel: w507 -> [_ _ _]
              tunnel: w509 -> [_ w516 _]
              tunnel: [w514 w515 w547] -> w508
              frame 0, Default {
              }
              frame 1 {
                n235 = for {
                  N: w517 -> [_]
                  tunnel: w518 -> [w525]
                  shift-right: [w520] -> w515
                  shift-left: w519 -> [w524]
                  tunnel: w516 -> [w521]
                  i -> [w523]
                  n236 = Index Array(array=w521, index=w523) -> (element=w522:bool)
                  n237 = case shown="True" w522 {
                    tunnel: w525 -> [_ w546]
                    tunnel: w524 -> [w526 w527]
                    tunnel: [w526 w528] -> w520
                    tunnel: w523 -> [_ w545]
                    frame False {
                    }
                    frame True {
                      n238 = Quotient & Remainder(x=w545, y=4) -> (x-y*floor(x/y)=w531:i32, floor(x/y)=w530:i32)
                      n239 = Multiply(x=4, y=w530) -> (x*y=w541:i32)
                      n240 = Add(x=w541, y=w531) -> (x+y=w540:i32)
                      n241 = property class="WFChart (strict)"(reference=w546, "Active Plot"=w540) -> (reference out=w543:refnum<vi>)  [unwired: 1 in, 1 out]
                      n242 = Index Array(array=w527, index (row)=w530, index (col)=w531) -> (element=w529:T11)
                      n243 = Unbundle By Name(w529) -> ("TC Label"=w532:string, "Alarm Status"=w538:string, "Temperature"=w537:string, "PlotColor"=w534:u32, "Alarm Color"=w533:u32)
                      n244 = property class="WFChart (strict)"(reference=w543, "Plot.Visible?"=TRUE ("Plot.Visible")) -> ()  [unwired: 1 in, 2 out]
                      n245 = Bundle By Name(cluster=w529, "TC Label"=w532, "Alarm Status"=w538, "Alarm Color"=w533, "Temperature"=w537, "PlotColor"=w534, "Graph On/Off"=u32 6618880) -> (w536:T11)
                      n246 = Replace Array Subset(array=w527, new element=w536, index (row)=w530, index (col)=w531) -> (w528:T3)
                    }
                  }
                }
              }
              frame 2 {
                n247 = for {
                  N: w548 -> [_]
                  tunnel: w549 -> [w568]
                  shift-right: [w551] -> w547
                  shift-left: w550 -> [w555]
                  i -> [w569]
                  w561 = u32 12369084
                  n248 = local read "working array"() -> (w570:bool[])
                  n249 = Quotient & Remainder(x=w569, y=4 ("Numeric")) -> (x-y*floor(x/y)=w553:i32, floor(x/y)=w552:i32)
                  n250 = Index Array(array=w555, index (row)=w552, index (col)=w553) -> (element=w560:T11)
                  n251 = Multiply(x=4, y=w552) -> (x*y=w564:i32)
                  n252 = Add(x=w564, y=w553) -> (x+y=w563:i32)
                  n253 = Index Array(array=w570, index=w569) -> ()  [unwired: 1 out]
                  n254 = property class="WFChart (strict)"(reference=w568, "Active Plot"=w563) -> (reference out=w566:refnum<vi>)  [unwired: 1 in, 1 out]
                  n255 = Unbundle By Name(w560) -> ("TC Label"=w559:string, "Alarm Status"=w558:string, "Temperature"=w557:string, "PlotColor"=w556:u32)
                  n256 = property class="WFChart (strict)"(reference=w566, "Plot.Visible?"=FALSE ("Plot.Visible")) -> ()  [unwired: 1 in, 2 out]
                  n257 = Bundle By Name(cluster=w560, "TC Label"=w559, "Alarm Status"=w558, "Alarm Color"=w561, "Temperature"=w557, "PlotColor"=w556, "Graph On/Off"=w561) -> (w554:T11)
                  n258 = Replace Array Subset(array=w555, new element=w554, index (row)=w552, index (col)=w553) -> (w551:T3)
                }
              }
            }
            n259 = Bundle By Name(cluster=w507, "Thermocouples"=w508) -> (w505:T10)
          }
          event "Set Time TC Graph": Mouse Down {
            n260 = event-data() -> ()  [unwired: 1 in, 8 out]
            n261 = local read "Log/Linear Y-Axis"() -> (w572:u16)
            n262 = control-ref of="Waveform Chart"() -> (w571:refnum<vi>)
            n263 = property on="Property Node" class="WFChart (strict)"(reference=w571, "YScale.Mapping Mode"=w572) -> ()  [unwired: 1 in, 2 out]
            n264 = local read "Total Time"() -> (w573:dbl)
            n265 = local read "Time Scale"() -> (w574:u16)
            n266 = case shown="2" w574 {
              tunnel: w571 -> [w579 w598 w617]
              tunnel: w573 -> [w577 w596 w615]
              frame 0, Default {
                n267 = Not Equal To 0?(x=w577) -> (x != 0?=w578:bool)
                n268 = case shown="True" w578 {
                  tunnel: w579 -> [w581 w593]
                  tunnel: w577 -> [_ w587]
                  frame False {
                    n269 = property on="Property Node" class="WFChart (strict)"(reference=w581) -> (reference out=w580:refnum<vi>, "XScale.Range"=w586:T21)  [unwired: 1 in, 1 out]
                    n270 = Bundle By Name(cluster=w586, "Minimum"=0.0, "Maximum"=3600.0, "Increment"=60.0) -> (w585:T21)
                    n271 = property on="Property Node" class="WFChart (strict)"(reference=w580, "XScale.Range"=w585) -> ()  [unwired: 1 in, 2 out]
                  }
                  frame True {
                    n272 = property on="Property Node" class="WFChart (strict)"(reference=w593) -> (reference out=w590:refnum<vi>, "XScale.Range"=w595:T21)  [unwired: 1 in, 1 out]
                    n273 = Multiply(x=w587, y=60.0) -> (x*y=w589:dbl)
                    n274 = Bundle By Name(cluster=w595, "Minimum"=0.0, "Maximum"=w589, "Increment"=1.0) -> (w594:T21)
                    n275 = property on="Property Node" class="WFChart (strict)"(reference=w590, "XScale.Range"=w594) -> ()  [unwired: 1 in, 2 out]
                  }
                }
              }
              frame 1 {
                n276 = Not Equal To 0?(x=w596) -> (x != 0?=w597:bool)
                n277 = case shown="True" w597 {
                  tunnel: w598 -> [w600 w610]
                  tunnel: w596 -> [_ w607]
                  frame False {
                    n278 = property on="Property Node" class="WFChart (strict)"(reference=w600) -> (reference out=w599:refnum<vi>, "XScale.Range"=w605:T21)  [unwired: 1 in, 1 out]
                    n279 = Bundle By Name(cluster=w605, "Minimum"=0.0, "Maximum"=43200.0, "Increment"=3600.0) -> (w601:T21)
                    n280 = property on="Property Node" class="WFChart (strict)"(reference=w599, "XScale.Range"=w601) -> ()  [unwired: 1 in, 2 out]
                  }
                  frame True {
                    n281 = Multiply(x=w607, y=3600.0) -> (x*y=w606:dbl)
                    n282 = property on="Property Node" class="WFChart (strict)"(reference=w610) -> (reference out=w609:refnum<vi>, "XScale.Range"=w614:T21)  [unwired: 1 in, 1 out]
                    n283 = Bundle By Name(cluster=w614, "Minimum"=0.0, "Maximum"=w606, "Increment"=3600.0) -> (w611:T21)
                    n284 = property on="Property Node" class="WFChart (strict)"(reference=w609, "XScale.Range"=w611) -> ()  [unwired: 1 in, 2 out]
                  }
                }
              }
              frame 2 {
                n285 = Not Equal To 0?(x=w615) -> (x != 0?=w616:bool)
                n286 = case shown="True" w616 {
                  tunnel: w617 -> [w619 w627]
                  tunnel: w615 -> [_ w625]
                  frame False {
                    n287 = property on="Property Node" class="WFChart (strict)"(reference=w619) -> (reference out=w618:refnum<vi>, "XScale.Range"=w624:T21)  [unwired: 1 in, 1 out]
                    n288 = Bundle By Name(cluster=w624, "Minimum"=0.0, "Maximum"=60.0, "Increment"=1.0) -> (w620:T21)
                    n289 = property on="Property Node" class="WFChart (strict)"(reference=w618, "XScale.Range"=w620) -> ()  [unwired: 1 in, 2 out]
                  }
                  frame True {
                    n290 = property on="Property Node" class="WFChart (strict)"(reference=w627) -> (reference out=w626:refnum<vi>, "XScale.Range"=w631:T21)  [unwired: 1 in, 1 out]
                    n291 = Bundle By Name(cluster=w631, "Minimum"=0.0, "Maximum"=w625, "Increment"=1.0) -> (w628:T21)
                    n292 = property on="Property Node" class="WFChart (strict)"(reference=w626, "XScale.Range"=w628) -> ()  [unwired: 1 in, 2 out]
                  }
                }
              }
            }
          }
          event "Set Time TC Graph 1": Mouse Down {
            n293 = event-data() -> ()  [unwired: 1 in, 8 out]
            n294 = local read "Log/Linear Y-Axis 1"() -> (w633:u16)
            n295 = control-ref of="Custom Chart 1"() -> (w632:refnum<vi>)
            n296 = property on="Property Node" class="WFChart (strict)"(reference=w632, "YScale.Mapping Mode"=w633) -> ()  [unwired: 1 in, 2 out]
            n297 = local read "Total Time 1"() -> (w634:dbl)
            n298 = local read "Time Scale 1"() -> (w635:u16)
            n299 = case shown="2" w635 {
              tunnel: w632 -> [w640 w659 w678]
              tunnel: w634 -> [w638 w657 w676]
              frame 0, Default {
                n300 = Not Equal To 0?(x=w638) -> (x != 0?=w639:bool)
                n301 = case shown="True" w639 {
                  tunnel: w640 -> [w642 w654]
                  tunnel: w638 -> [_ w648]
                  frame False {
                    n302 = property on="Property Node" class="WFChart (strict)"(reference=w642) -> (reference out=w641:refnum<vi>, "XScale.Range"=w647:T21)  [unwired: 1 in, 1 out]
                    n303 = Bundle By Name(cluster=w647, "Minimum"=0.0, "Maximum"=3600.0, "Increment"=60.0) -> (w646:T21)
                    n304 = property on="Property Node" class="WFChart (strict)"(reference=w641, "XScale.Range"=w646) -> ()  [unwired: 1 in, 2 out]
                  }
                  frame True {
                    n305 = property on="Property Node" class="WFChart (strict)"(reference=w654) -> (reference out=w651:refnum<vi>, "XScale.Range"=w656:T21)  [unwired: 1 in, 1 out]
                    n306 = Multiply(x=w648, y=60.0) -> (x*y=w650:dbl)
                    n307 = Bundle By Name(cluster=w656, "Minimum"=0.0, "Maximum"=w650, "Increment"=1.0) -> (w655:T21)
                    n308 = property on="Property Node" class="WFChart (strict)"(reference=w651, "XScale.Range"=w655) -> ()  [unwired: 1 in, 2 out]
                  }
                }
              }
              frame 1 {
                n309 = Not Equal To 0?(x=w657) -> (x != 0?=w658:bool)
                n310 = case shown="True" w658 {
                  tunnel: w659 -> [w661 w671]
                  tunnel: w657 -> [_ w668]
                  frame False {
                    n311 = property on="Property Node" class="WFChart (strict)"(reference=w661) -> (reference out=w660:refnum<vi>, "XScale.Range"=w666:T21)  [unwired: 1 in, 1 out]
                    n312 = Bundle By Name(cluster=w666, "Minimum"=0.0, "Maximum"=43200.0, "Increment"=3600.0) -> (w662:T21)
                    n313 = property on="Property Node" class="WFChart (strict)"(reference=w660, "XScale.Range"=w662) -> ()  [unwired: 1 in, 2 out]
                  }
                  frame True {
                    n314 = Multiply(x=w668, y=3600.0) -> (x*y=w667:dbl)
                    n315 = property on="Property Node" class="WFChart (strict)"(reference=w671) -> (reference out=w670:refnum<vi>, "XScale.Range"=w675:T21)  [unwired: 1 in, 1 out]
                    n316 = Bundle By Name(cluster=w675, "Minimum"=0.0, "Maximum"=w667, "Increment"=3600.0) -> (w672:T21)
                    n317 = property on="Property Node" class="WFChart (strict)"(reference=w670, "XScale.Range"=w672) -> ()  [unwired: 1 in, 2 out]
                  }
                }
              }
              frame 2 {
                n318 = Not Equal To 0?(x=w676) -> (x != 0?=w677:bool)
                n319 = case shown="True" w677 {
                  tunnel: w678 -> [w680 w688]
                  tunnel: w676 -> [_ w686]
                  frame False {
                    n320 = property on="Property Node" class="WFChart (strict)"(reference=w680) -> (reference out=w679:refnum<vi>, "XScale.Range"=w685:T21)  [unwired: 1 in, 1 out]
                    n321 = Bundle By Name(cluster=w685, "Minimum"=0.0, "Maximum"=60.0, "Increment"=1.0) -> (w681:T21)
                    n322 = property on="Property Node" class="WFChart (strict)"(reference=w679, "XScale.Range"=w681) -> ()  [unwired: 1 in, 2 out]
                  }
                  frame True {
                    n323 = property on="Property Node" class="WFChart (strict)"(reference=w688) -> (reference out=w687:refnum<vi>, "XScale.Range"=w692:T21)  [unwired: 1 in, 1 out]
                    n324 = Bundle By Name(cluster=w692, "Minimum"=0.0, "Maximum"=w686, "Increment"=1.0) -> (w689:T21)
                    n325 = property on="Property Node" class="WFChart (strict)"(reference=w687, "XScale.Range"=w689) -> ()  [unwired: 1 in, 2 out]
                  }
                }
              }
            }
          }
          event "Set Time TC Graph 2": Mouse Down {
            n326 = event-data() -> ()  [unwired: 1 in, 8 out]
            n327 = local read "Log/Linear Y-Axis 2"() -> (w694:u16)
            n328 = control-ref of="Custom Chart 2"() -> (w693:refnum<vi>)
            n329 = property on="Property Node" class="WFChart (strict)"(reference=w693, "YScale.Mapping Mode"=w694) -> ()  [unwired: 1 in, 2 out]
            n330 = local read "Total Time 2"() -> (w695:dbl)
            n331 = local read "Time Scale 2"() -> (w696:u16)
            n332 = case shown="2" w696 {
              tunnel: w693 -> [w701 w720 w739]
              tunnel: w695 -> [w699 w718 w737]
              frame 0, Default {
                n333 = Not Equal To 0?(x=w699) -> (x != 0?=w700:bool)
                n334 = case shown="True" w700 {
                  tunnel: w701 -> [w703 w715]
                  tunnel: w699 -> [_ w709]
                  frame False {
                    n335 = property on="Property Node" class="WFChart (strict)"(reference=w703) -> (reference out=w702:refnum<vi>, "XScale.Range"=w708:T21)  [unwired: 1 in, 1 out]
                    n336 = Bundle By Name(cluster=w708, "Minimum"=0.0, "Maximum"=3600.0, "Increment"=60.0) -> (w707:T21)
                    n337 = property on="Property Node" class="WFChart (strict)"(reference=w702, "XScale.Range"=w707) -> ()  [unwired: 1 in, 2 out]
                  }
                  frame True {
                    n338 = property on="Property Node" class="WFChart (strict)"(reference=w715) -> (reference out=w712:refnum<vi>, "XScale.Range"=w717:T21)  [unwired: 1 in, 1 out]
                    n339 = Multiply(x=w709, y=60.0) -> (x*y=w711:dbl)
                    n340 = Bundle By Name(cluster=w717, "Minimum"=0.0, "Maximum"=w711, "Increment"=1.0) -> (w716:T21)
                    n341 = property on="Property Node" class="WFChart (strict)"(reference=w712, "XScale.Range"=w716) -> ()  [unwired: 1 in, 2 out]
                  }
                }
              }
              frame 1 {
                n342 = Not Equal To 0?(x=w718) -> (x != 0?=w719:bool)
                n343 = case shown="True" w719 {
                  tunnel: w720 -> [w722 w732]
                  tunnel: w718 -> [_ w729]
                  frame False {
                    n344 = property on="Property Node" class="WFChart (strict)"(reference=w722) -> (reference out=w721:refnum<vi>, "XScale.Range"=w727:T21)  [unwired: 1 in, 1 out]
                    n345 = Bundle By Name(cluster=w727, "Minimum"=0.0, "Maximum"=43200.0, "Increment"=3600.0) -> (w723:T21)
                    n346 = property on="Property Node" class="WFChart (strict)"(reference=w721, "XScale.Range"=w723) -> ()  [unwired: 1 in, 2 out]
                  }
                  frame True {
                    n347 = Multiply(x=w729, y=3600.0) -> (x*y=w728:dbl)
                    n348 = property on="Property Node" class="WFChart (strict)"(reference=w732) -> (reference out=w731:refnum<vi>, "XScale.Range"=w736:T21)  [unwired: 1 in, 1 out]
                    n349 = Bundle By Name(cluster=w736, "Minimum"=0.0, "Maximum"=w728, "Increment"=3600.0) -> (w733:T21)
                    n350 = property on="Property Node" class="WFChart (strict)"(reference=w731, "XScale.Range"=w733) -> ()  [unwired: 1 in, 2 out]
                  }
                }
              }
              frame 2 {
                n351 = Not Equal To 0?(x=w737) -> (x != 0?=w738:bool)
                n352 = case shown="True" w738 {
                  tunnel: w739 -> [w741 w749]
                  tunnel: w737 -> [_ w747]
                  frame False {
                    n353 = property on="Property Node" class="WFChart (strict)"(reference=w741) -> (reference out=w740:refnum<vi>, "XScale.Range"=w746:T21)  [unwired: 1 in, 1 out]
                    n354 = Bundle By Name(cluster=w746, "Minimum"=0.0, "Maximum"=60.0, "Increment"=1.0) -> (w742:T21)
                    n355 = property on="Property Node" class="WFChart (strict)"(reference=w740, "XScale.Range"=w742) -> ()  [unwired: 1 in, 2 out]
                  }
                  frame True {
                    n356 = property on="Property Node" class="WFChart (strict)"(reference=w749) -> (reference out=w748:refnum<vi>, "XScale.Range"=w753:T21)  [unwired: 1 in, 1 out]
                    n357 = Bundle By Name(cluster=w753, "Minimum"=0.0, "Maximum"=w747, "Increment"=1.0) -> (w750:T21)
                    n358 = property on="Property Node" class="WFChart (strict)"(reference=w748, "XScale.Range"=w750) -> ()  [unwired: 1 in, 2 out]
                  }
                }
              }
            }
          }
          event "Set Time TC Graph 3": Mouse Down {
            n359 = event-data() -> ()  [unwired: 1 in, 8 out]
            n360 = local read "Log/Linear Y-Axis 3"() -> (w755:u16)
            n361 = control-ref of="Custom Chart 3"() -> (w754:refnum<vi>)
            n362 = property on="Property Node" class="WFChart (strict)"(reference=w754, "YScale.Mapping Mode"=w755) -> ()  [unwired: 1 in, 2 out]
            n363 = local read "Total Time 3"() -> (w756:dbl)
            n364 = local read "Time Scale 3"() -> (w757:u16)
            n365 = case shown="2" w757 {
              tunnel: w754 -> [w762 w781 w800]
              tunnel: w756 -> [w760 w779 w798]
              frame 0, Default {
                n366 = Not Equal To 0?(x=w760) -> (x != 0?=w761:bool)
                n367 = case shown="True" w761 {
                  tunnel: w762 -> [w764 w776]
                  tunnel: w760 -> [_ w770]
                  frame False {
                    n368 = property on="Property Node" class="WFChart (strict)"(reference=w764) -> (reference out=w763:refnum<vi>, "XScale.Range"=w769:T21)  [unwired: 1 in, 1 out]
                    n369 = Bundle By Name(cluster=w769, "Minimum"=0.0, "Maximum"=3600.0, "Increment"=60.0) -> (w768:T21)
                    n370 = property on="Property Node" class="WFChart (strict)"(reference=w763, "XScale.Range"=w768) -> ()  [unwired: 1 in, 2 out]
                  }
                  frame True {
                    n371 = property on="Property Node" class="WFChart (strict)"(reference=w776) -> (reference out=w773:refnum<vi>, "XScale.Range"=w778:T21)  [unwired: 1 in, 1 out]
                    n372 = Multiply(x=w770, y=60.0) -> (x*y=w772:dbl)
                    n373 = Bundle By Name(cluster=w778, "Minimum"=0.0, "Maximum"=w772, "Increment"=1.0) -> (w777:T21)
                    n374 = property on="Property Node" class="WFChart (strict)"(reference=w773, "XScale.Range"=w777) -> ()  [unwired: 1 in, 2 out]
                  }
                }
              }
              frame 1 {
                n375 = Not Equal To 0?(x=w779) -> (x != 0?=w780:bool)
                n376 = case shown="True" w780 {
                  tunnel: w781 -> [w783 w793]
                  tunnel: w779 -> [_ w790]
                  frame False {
                    n377 = property on="Property Node" class="WFChart (strict)"(reference=w783) -> (reference out=w782:refnum<vi>, "XScale.Range"=w788:T21)  [unwired: 1 in, 1 out]
                    n378 = Bundle By Name(cluster=w788, "Minimum"=0.0, "Maximum"=43200.0, "Increment"=3600.0) -> (w784:T21)
                    n379 = property on="Property Node" class="WFChart (strict)"(reference=w782, "XScale.Range"=w784) -> ()  [unwired: 1 in, 2 out]
                  }
                  frame True {
                    n380 = Multiply(x=w790, y=3600.0) -> (x*y=w789:dbl)
                    n381 = property on="Property Node" class="WFChart (strict)"(reference=w793) -> (reference out=w792:refnum<vi>, "XScale.Range"=w797:T21)  [unwired: 1 in, 1 out]
                    n382 = Bundle By Name(cluster=w797, "Minimum"=0.0, "Maximum"=w789, "Increment"=3600.0) -> (w794:T21)
                    n383 = property on="Property Node" class="WFChart (strict)"(reference=w792, "XScale.Range"=w794) -> ()  [unwired: 1 in, 2 out]
                  }
                }
              }
              frame 2 {
                n384 = Not Equal To 0?(x=w798) -> (x != 0?=w799:bool)
                n385 = case shown="True" w799 {
                  tunnel: w800 -> [w802 w810]
                  tunnel: w798 -> [_ w808]
                  frame False {
                    n386 = property on="Property Node" class="WFChart (strict)"(reference=w802) -> (reference out=w801:refnum<vi>, "XScale.Range"=w807:T21)  [unwired: 1 in, 1 out]
                    n387 = Bundle By Name(cluster=w807, "Minimum"=0.0, "Maximum"=60.0, "Increment"=1.0) -> (w803:T21)
                    n388 = property on="Property Node" class="WFChart (strict)"(reference=w801, "XScale.Range"=w803) -> ()  [unwired: 1 in, 2 out]
                  }
                  frame True {
                    n389 = property on="Property Node" class="WFChart (strict)"(reference=w810) -> (reference out=w809:refnum<vi>, "XScale.Range"=w814:T21)  [unwired: 1 in, 1 out]
                    n390 = Bundle By Name(cluster=w814, "Minimum"=0.0, "Maximum"=w808, "Increment"=1.0) -> (w811:T21)
                    n391 = property on="Property Node" class="WFChart (strict)"(reference=w809, "XScale.Range"=w811) -> ()  [unwired: 1 in, 2 out]
                  }
                }
              }
            }
          }
          event "Set Time TC Graph 4": Mouse Down {
            n392 = event-data() -> ()  [unwired: 1 in, 8 out]
            n393 = local read "Log/Linear Y-Axis 4"() -> (w816:u16)
            n394 = control-ref of="Custom Chart 4"() -> (w815:refnum<vi>)
            n395 = property on="Property Node" class="WFChart (strict)"(reference=w815, "YScale.Mapping Mode"=w816) -> ()  [unwired: 1 in, 2 out]
            n396 = local read "Total Time 4"() -> (w817:dbl)
            n397 = local read "Time Scale 4"() -> (w818:u16)
            n398 = case shown="2" w818 {
              tunnel: w815 -> [w823 w842 w861]
              tunnel: w817 -> [w821 w840 w859]
              frame 0, Default {
                n399 = Not Equal To 0?(x=w821) -> (x != 0?=w822:bool)
                n400 = case shown="True" w822 {
                  tunnel: w823 -> [w825 w837]
                  tunnel: w821 -> [_ w831]
                  frame False {
                    n401 = property on="Property Node" class="WFChart (strict)"(reference=w825) -> (reference out=w824:refnum<vi>, "XScale.Range"=w830:T21)  [unwired: 1 in, 1 out]
                    n402 = Bundle By Name(cluster=w830, "Minimum"=0.0, "Maximum"=3600.0, "Increment"=60.0) -> (w829:T21)
                    n403 = property on="Property Node" class="WFChart (strict)"(reference=w824, "XScale.Range"=w829) -> ()  [unwired: 1 in, 2 out]
                  }
                  frame True {
                    n404 = property on="Property Node" class="WFChart (strict)"(reference=w837) -> (reference out=w834:refnum<vi>, "XScale.Range"=w839:T21)  [unwired: 1 in, 1 out]
                    n405 = Multiply(x=w831, y=60.0) -> (x*y=w833:dbl)
                    n406 = Bundle By Name(cluster=w839, "Minimum"=0.0, "Maximum"=w833, "Increment"=1.0) -> (w838:T21)
                    n407 = property on="Property Node" class="WFChart (strict)"(reference=w834, "XScale.Range"=w838) -> ()  [unwired: 1 in, 2 out]
                  }
                }
              }
              frame 1 {
                n408 = Not Equal To 0?(x=w840) -> (x != 0?=w841:bool)
                n409 = case shown="True" w841 {
                  tunnel: w842 -> [w844 w854]
                  tunnel: w840 -> [_ w851]
                  frame False {
                    n410 = property on="Property Node" class="WFChart (strict)"(reference=w844) -> (reference out=w843:refnum<vi>, "XScale.Range"=w849:T21)  [unwired: 1 in, 1 out]
                    n411 = Bundle By Name(cluster=w849, "Minimum"=0.0, "Maximum"=43200.0, "Increment"=3600.0) -> (w845:T21)
                    n412 = property on="Property Node" class="WFChart (strict)"(reference=w843, "XScale.Range"=w845) -> ()  [unwired: 1 in, 2 out]
                  }
                  frame True {
                    n413 = Multiply(x=w851, y=3600.0) -> (x*y=w850:dbl)
                    n414 = property on="Property Node" class="WFChart (strict)"(reference=w854) -> (reference out=w853:refnum<vi>, "XScale.Range"=w858:T21)  [unwired: 1 in, 1 out]
                    n415 = Bundle By Name(cluster=w858, "Minimum"=0.0, "Maximum"=w850, "Increment"=3600.0) -> (w855:T21)
                    n416 = property on="Property Node" class="WFChart (strict)"(reference=w853, "XScale.Range"=w855) -> ()  [unwired: 1 in, 2 out]
                  }
                }
              }
              frame 2 {
                n417 = Not Equal To 0?(x=w859) -> (x != 0?=w860:bool)
                n418 = case shown="True" w860 {
                  tunnel: w861 -> [w863 w871]
                  tunnel: w859 -> [_ w869]
                  frame False {
                    n419 = property on="Property Node" class="WFChart (strict)"(reference=w863) -> (reference out=w862:refnum<vi>, "XScale.Range"=w868:T21)  [unwired: 1 in, 1 out]
                    n420 = Bundle By Name(cluster=w868, "Minimum"=0.0, "Maximum"=60.0, "Increment"=1.0) -> (w864:T21)
                    n421 = property on="Property Node" class="WFChart (strict)"(reference=w862, "XScale.Range"=w864) -> ()  [unwired: 1 in, 2 out]
                  }
                  frame True {
                    n422 = property on="Property Node" class="WFChart (strict)"(reference=w871) -> (reference out=w870:refnum<vi>, "XScale.Range"=w875:T21)  [unwired: 1 in, 1 out]
                    n423 = Bundle By Name(cluster=w875, "Minimum"=0.0, "Maximum"=w869, "Increment"=1.0) -> (w872:T21)
                    n424 = property on="Property Node" class="WFChart (strict)"(reference=w870, "XScale.Range"=w872) -> ()  [unwired: 1 in, 2 out]
                  }
                }
              }
            }
          }
          event "Set Time TC Graph 5": Mouse Down {
            n425 = event-data() -> ()  [unwired: 1 in, 8 out]
            n426 = local read "Log/Linear Y-Axis 5"() -> (w877:u16)
            n427 = control-ref of="Custom Chart 5"() -> (w876:refnum<vi>)
            n428 = property on="Property Node" class="WFChart (strict)"(reference=w876, "YScale.Mapping Mode"=w877) -> ()  [unwired: 1 in, 2 out]
            n429 = local read "Total Time 5"() -> (w878:dbl)
            n430 = local read "Time Scale 5"() -> (w879:u16)
            n431 = case shown="2" w879 {
              tunnel: w876 -> [w884 w903 w922]
              tunnel: w878 -> [w882 w901 w920]
              frame 0, Default {
                n432 = Not Equal To 0?(x=w882) -> (x != 0?=w883:bool)
                n433 = case shown="True" w883 {
                  tunnel: w884 -> [w886 w898]
                  tunnel: w882 -> [_ w892]
                  frame False {
                    n434 = property on="Property Node" class="WFChart (strict)"(reference=w886) -> (reference out=w885:refnum<vi>, "XScale.Range"=w891:T21)  [unwired: 1 in, 1 out]
                    n435 = Bundle By Name(cluster=w891, "Minimum"=0.0, "Maximum"=3600.0, "Increment"=60.0) -> (w890:T21)
                    n436 = property on="Property Node" class="WFChart (strict)"(reference=w885, "XScale.Range"=w890) -> ()  [unwired: 1 in, 2 out]
                  }
                  frame True {
                    n437 = property on="Property Node" class="WFChart (strict)"(reference=w898) -> (reference out=w895:refnum<vi>, "XScale.Range"=w900:T21)  [unwired: 1 in, 1 out]
                    n438 = Multiply(x=w892, y=60.0) -> (x*y=w894:dbl)
                    n439 = Bundle By Name(cluster=w900, "Minimum"=0.0, "Maximum"=w894, "Increment"=1.0) -> (w899:T21)
                    n440 = property on="Property Node" class="WFChart (strict)"(reference=w895, "XScale.Range"=w899) -> ()  [unwired: 1 in, 2 out]
                  }
                }
              }
              frame 1 {
                n441 = Not Equal To 0?(x=w901) -> (x != 0?=w902:bool)
                n442 = case shown="True" w902 {
                  tunnel: w903 -> [w905 w915]
                  tunnel: w901 -> [_ w912]
                  frame False {
                    n443 = property on="Property Node" class="WFChart (strict)"(reference=w905) -> (reference out=w904:refnum<vi>, "XScale.Range"=w910:T21)  [unwired: 1 in, 1 out]
                    n444 = Bundle By Name(cluster=w910, "Minimum"=0.0, "Maximum"=43200.0, "Increment"=3600.0) -> (w906:T21)
                    n445 = property on="Property Node" class="WFChart (strict)"(reference=w904, "XScale.Range"=w906) -> ()  [unwired: 1 in, 2 out]
                  }
                  frame True {
                    n446 = Multiply(x=w912, y=3600.0) -> (x*y=w911:dbl)
                    n447 = property on="Property Node" class="WFChart (strict)"(reference=w915) -> (reference out=w914:refnum<vi>, "XScale.Range"=w919:T21)  [unwired: 1 in, 1 out]
                    n448 = Bundle By Name(cluster=w919, "Minimum"=0.0, "Maximum"=w911, "Increment"=3600.0) -> (w916:T21)
                    n449 = property on="Property Node" class="WFChart (strict)"(reference=w914, "XScale.Range"=w916) -> ()  [unwired: 1 in, 2 out]
                  }
                }
              }
              frame 2 {
                n450 = Not Equal To 0?(x=w920) -> (x != 0?=w921:bool)
                n451 = case shown="True" w921 {
                  tunnel: w922 -> [w924 w932]
                  tunnel: w920 -> [_ w930]
                  frame False {
                    n452 = property on="Property Node" class="WFChart (strict)"(reference=w924) -> (reference out=w923:refnum<vi>, "XScale.Range"=w929:T21)  [unwired: 1 in, 1 out]
                    n453 = Bundle By Name(cluster=w929, "Minimum"=0.0, "Maximum"=60.0, "Increment"=1.0) -> (w925:T21)
                    n454 = property on="Property Node" class="WFChart (strict)"(reference=w923, "XScale.Range"=w925) -> ()  [unwired: 1 in, 2 out]
                  }
                  frame True {
                    n455 = property on="Property Node" class="WFChart (strict)"(reference=w932) -> (reference out=w931:refnum<vi>, "XScale.Range"=w936:T21)  [unwired: 1 in, 1 out]
                    n456 = Bundle By Name(cluster=w936, "Minimum"=0.0, "Maximum"=w930, "Increment"=1.0) -> (w933:T21)
                    n457 = property on="Property Node" class="WFChart (strict)"(reference=w931, "XScale.Range"=w933) -> ()  [unwired: 1 in, 2 out]
                  }
                }
              }
            }
          }
          event "Set Time TC Graph 6": Mouse Down {
            n458 = event-data() -> ()  [unwired: 1 in, 8 out]
            n459 = local read "Log/Linear Y-Axis 6"() -> (w938:u16)
            n460 = control-ref of="Custom Chart 6"() -> (w937:refnum<vi>)
            n461 = property on="Property Node" class="WFChart (strict)"(reference=w937, "YScale.Mapping Mode"=w938) -> ()  [unwired: 1 in, 2 out]
            n462 = local read "Total Time 6"() -> (w939:dbl)
            n463 = local read "Time Scale 6"() -> (w940:u16)
            n464 = case shown="2" w940 {
              tunnel: w937 -> [w945 w964 w983]
              tunnel: w939 -> [w943 w962 w981]
              frame 0, Default {
                n465 = Not Equal To 0?(x=w943) -> (x != 0?=w944:bool)
                n466 = case shown="True" w944 {
                  tunnel: w945 -> [w947 w959]
                  tunnel: w943 -> [_ w953]
                  frame False {
                    n467 = property on="Property Node" class="WFChart (strict)"(reference=w947) -> (reference out=w946:refnum<vi>, "XScale.Range"=w952:T21)  [unwired: 1 in, 1 out]
                    n468 = Bundle By Name(cluster=w952, "Minimum"=0.0, "Maximum"=3600.0, "Increment"=60.0) -> (w951:T21)
                    n469 = property on="Property Node" class="WFChart (strict)"(reference=w946, "XScale.Range"=w951) -> ()  [unwired: 1 in, 2 out]
                  }
                  frame True {
                    n470 = property on="Property Node" class="WFChart (strict)"(reference=w959) -> (reference out=w956:refnum<vi>, "XScale.Range"=w961:T21)  [unwired: 1 in, 1 out]
                    n471 = Multiply(x=w953, y=60.0) -> (x*y=w955:dbl)
                    n472 = Bundle By Name(cluster=w961, "Minimum"=0.0, "Maximum"=w955, "Increment"=1.0) -> (w960:T21)
                    n473 = property on="Property Node" class="WFChart (strict)"(reference=w956, "XScale.Range"=w960) -> ()  [unwired: 1 in, 2 out]
                  }
                }
              }
              frame 1 {
                n474 = Not Equal To 0?(x=w962) -> (x != 0?=w963:bool)
                n475 = case shown="True" w963 {
                  tunnel: w964 -> [w966 w976]
                  tunnel: w962 -> [_ w973]
                  frame False {
                    n476 = property on="Property Node" class="WFChart (strict)"(reference=w966) -> (reference out=w965:refnum<vi>, "XScale.Range"=w971:T21)  [unwired: 1 in, 1 out]
                    n477 = Bundle By Name(cluster=w971, "Minimum"=0.0, "Maximum"=43200.0, "Increment"=3600.0) -> (w967:T21)
                    n478 = property on="Property Node" class="WFChart (strict)"(reference=w965, "XScale.Range"=w967) -> ()  [unwired: 1 in, 2 out]
                  }
                  frame True {
                    n479 = Multiply(x=w973, y=3600.0) -> (x*y=w972:dbl)
                    n480 = property on="Property Node" class="WFChart (strict)"(reference=w976) -> (reference out=w975:refnum<vi>, "XScale.Range"=w980:T21)  [unwired: 1 in, 1 out]
                    n481 = Bundle By Name(cluster=w980, "Minimum"=0.0, "Maximum"=w972, "Increment"=3600.0) -> (w977:T21)
                    n482 = property on="Property Node" class="WFChart (strict)"(reference=w975, "XScale.Range"=w977) -> ()  [unwired: 1 in, 2 out]
                  }
                }
              }
              frame 2 {
                n483 = Not Equal To 0?(x=w981) -> (x != 0?=w982:bool)
                n484 = case shown="True" w982 {
                  tunnel: w983 -> [w985 w993]
                  tunnel: w981 -> [_ w991]
                  frame False {
                    n485 = property on="Property Node" class="WFChart (strict)"(reference=w985) -> (reference out=w984:refnum<vi>, "XScale.Range"=w990:T21)  [unwired: 1 in, 1 out]
                    n486 = Bundle By Name(cluster=w990, "Minimum"=0.0, "Maximum"=60.0, "Increment"=1.0) -> (w986:T21)
                    n487 = property on="Property Node" class="WFChart (strict)"(reference=w984, "XScale.Range"=w986) -> ()  [unwired: 1 in, 2 out]
                  }
                  frame True {
                    n488 = property on="Property Node" class="WFChart (strict)"(reference=w993) -> (reference out=w992:refnum<vi>, "XScale.Range"=w997:T21)  [unwired: 1 in, 1 out]
                    n489 = Bundle By Name(cluster=w997, "Minimum"=0.0, "Maximum"=w991, "Increment"=1.0) -> (w994:T21)
                    n490 = property on="Property Node" class="WFChart (strict)"(reference=w992, "XScale.Range"=w994) -> ()  [unwired: 1 in, 2 out]
                  }
                }
              }
            }
          }
          event "Run Profile": Mouse Down {
            n491 = event-data() -> ()  [unwired: 1 in, 1 out]
            n492 = Unbundle By Name(w1009) -> ("Http session"=w1008:T9, "URL prefex"=w1000:string)
            n493 = Flatten To JSON(anything=cluster{"profile_name":string} {"profile_name"="testSoak"}) -> (JSON string=w1004:string)  [unwired: 2 in, 1 out]
            n494 = Concatenate Strings(w1000, "loadProfile" ("url")) -> (w1006:string)
            n495 = call-poly <vilib>:"POST.vi"("client handle"=w1008, "url"=w1006, "buffer"=w1004) -> ("client handle out"=w1002:T9, "body"=→"body":string)  [unwired: 9 in, 2 out]
            n496 = Concatenate Strings(w1000, "runProfile" ("url")) -> (w999:string)
            n497 = call <vilib>:"GET.vi"("client handle"=w1002, "url"=w999) -> ("body"=→"body 2":string)  [unwired: 10 in, 3 out]
          }
          event "Hold Profile": Mouse Down {
            n498 = event-data() -> ()  [unwired: 1 in, 1 out]
            n499 = Unbundle By Name(w1016) -> ("URL prefex"=w1014:string)  [unwired: 1 out]
            n500 = Concatenate Strings(w1014, "hold" ("url")) -> (w1013:string)
            n501 = call <vilib>:"GET.vi"("url"=w1013, "error in (no error)"=w1012) -> ("error out"=w1011:errorcluster)  [unwired: 10 in, 3 out]
          }
          event "Pause Profile": Mouse Down {
            n502 = event-data() -> ()  [unwired: 1 in, 1 out]
            n503 = Unbundle By Name(w1022) -> ("URL prefex"=w1020:string)  [unwired: 1 out]
            n504 = Concatenate Strings(w1020, "pause" ("url")) -> (w1019:string)
            n505 = call <vilib>:"GET.vi"("url"=w1019, "error in (no error)"=w1018) -> ("error out"=w1017:errorcluster)  [unwired: 10 in, 3 out]
          }
          event "Resume Profile": Mouse Down {
            n506 = event-data() -> ()  [unwired: 1 in, 1 out]
            n507 = Unbundle By Name(w1028) -> ("URL prefex"=w1026:string)  [unwired: 1 out]
            n508 = Concatenate Strings(w1026, "resume" ("url")) -> (w1025:string)
            n509 = call <vilib>:"GET.vi"("url"=w1025, "error in (no error)"=w1024) -> ("error out"=w1023:errorcluster)  [unwired: 10 in, 3 out]
          }
          event "Stop Profile": Mouse Down {
            n510 = event-data() -> ()  [unwired: 1 in, 1 out]
            n511 = Unbundle By Name(w1034) -> ("URL prefex"=w1032:string)  [unwired: 1 out]
            n512 = Concatenate Strings(w1032, "hardStop" ("url")) -> (w1031:string)
            n513 = call <vilib>:"GET.vi"("url"=w1031, "error in (no error)"=w1030) -> ("error out"=w1029:errorcluster)  [unwired: 10 in, 3 out]
          }
          event "Generate Error": Mouse Down {
            n514 = event-data() -> ()  [unwired: 1 in, 1 out]
            n515 = One Button Dialog(message="There has been an error", button name ("OK")="Proceed to Error Log") -> (true=w1035:bool)
            "errortrue" <- w1035
            n516 = case shown="True" w1035 {
              frame False {
              }
              frame True {
                n517 = local write "Tab Control"(T12."General Status" ("Tab Control")) -> ()
              }
            }
          }
          event "Current Errors (click to clear)": Mouse Down {
            n518 = event-data() -> ("CtlRef"=w1048:refnum<vi>, "Coords"=w1047:T20)  [unwired: 1 in]
            n519 = invoke on="Invoke Node" class="MCListbox (strict)" method="Point To Row Column"(reference=w1048, "Point"=w1047) -> (reference out=w1044:refnum<vi>, "InBounds"=w1041:bool, "CellPosition"=w1045:T22)  [unwired: 5 in, 4 out]
            n520 = case shown="True" w1041 {
              tunnel: w1045 -> [_ w1061]
              tunnel: w1044 -> [_ w1060]
              tunnel: w1043 -> [w1049 w1057]
              tunnel: [w1049 w1056] -> w1042
              frame False {
              }
              frame True {
                n521 = Unbundle By Name(w1061) -> ("Row"=w1058:i32)
                n522 = property on="Property Node" class="MCListbox (strict)"(reference=w1060, "ActiveCell"=w1061) -> (reference out=w1053:refnum<vi>)  [unwired: 1 in, 1 out]
                n523 = Unbundle By Name(w1057) -> ("ErrorArray"=w1059:string[][], "PrevErrorArray"=w1055:string[][])
                n524 = control-ref of="Error History"() -> (w1051:refnum<vi>)
                n525 = Delete From Array(array=w1059, index (row)=w1058) -> (deleted portion=w1054:string[], array with subset deleted=w1052:string[][])  [unwired: 2 in]
                n526 = Build Array (concatenate)(w1054, w1055) -> (w1050:string[][])
                n527 = property on="Property Node" class="MCListbox (strict)"(reference=w1053, "ItemNames"=w1052) -> ()  [unwired: 1 in, 2 out]
                n528 = property on="Property Node" class="MCListbox (strict)"(reference=w1051, "ItemNames"=w1050) -> ()  [unwired: 1 in, 2 out]
                n529 = Bundle By Name(cluster=w1057, "ErrorArray"=w1052, "PrevErrorArray"=w1050) -> (w1056:T10)
              }
            }
          }
          event "ZoneSetup.Zone Selection": Mouse Down {
            n530 = event-data() -> ("CtlRef"=w1068:refnum<vi>, "Coords"=w1074:T20)  [unwired: 1 in]
            n531 = Unbundle By Name(w1065) -> ("ZonesSelected"=w1066:bool[])
            n532 = invoke on="Invoke Node" class="LstBox (strict)" method="Point To Row"(reference=w1068, "Point"=w1074) -> ("Row"=w1067:i32)  [unwired: 5 in, 6 out]
            n533 = property on="Property Node" class="LstBox (strict)"(reference=w1068) -> ("Item Symbols"=w1070:i32[])  [unwired: 1 in, 2 out]
            n534 = Index Array(array=w1070, index=w1067) -> (element=w1072:i32)
            n535 = Equal?(x=w1072, y=37) -> (x = y?=w1073:bool)
            n536 = case shown="True" w1073 {
              tunnel: w1070 -> [w1080 w1088]
              tunnel: w1067 -> [w1076 w1085]
              tunnel: [w1079 w1086] -> w1062
              tunnel: w1066 -> [w1078 w1083]
              tunnel: [w1075 w1082] -> w1063
              frame False {
                n537 = Replace Array Subset(array=w1078, new element=FALSE ("Boolean"), index=w1076) -> (w1075:bool[])
                n538 = Replace Array Subset(array=w1080, new element=37, index=w1076) -> (w1079:i32[])
              }
              frame True {
                n539 = Replace Array Subset(array=w1083, new element=TRUE ("Boolean"), index=w1085) -> (w1082:bool[])
                n540 = Replace Array Subset(array=w1088, new element=38, index=w1085) -> (w1086:i32[])
              }
            }
            n541 = Bundle By Name(cluster=w1065, "ZonesSelected"=w1063, "ZoneSetup.Zone Selection"=w1062) -> (w1064:T10)
            n542 = property on="Property Node" class="LstBox (strict)"(reference=w1068, "Item Symbols"=w1062) -> ()  [unwired: 1 in, 2 out]
          }
          event "ZoneSetup.Initiate Setup": Value Change {
            w1092 = TRUE ("Page Visible")
            n543 = event-data() -> ("CtlRef"=w1091:refnum<vi>, "OldVal"=w1090:bool)  [unwired: 1 in, 4 out]
            n544 = control-ref of="CreateTProfile"() -> (w1105:refnum<vi>)
            n545 = property class="Bool (strict)"(reference=w1091, "Value"=w1090) -> ()  [unwired: 1 in, 2 out]
            n546 = control-ref of="Zone Selection"() -> (w1104:refnum<vi>)
            n547 = property on="Property Node" class="TabCtl (strict)"(reference=w1105) -> ("Pages"=w1095:refnum<vi>[])  [unwired: 1 in, 2 out]
            n548 = property on="Property Node" class="LstBox (strict)"(reference=w1104) -> ("Item Symbols"=w1103:i32[])  [unwired: 1 in, 2 out]
            n549 = for {
              N: 13 -> [_]
              tunnel: w1103 -> [w1159]
              tunnel: w1095 -> [w1160] mode=indexing
              i -> [w1154]
              n550 = Greater?(x=w1154, y=1) -> (0:w1156:bool)
              n551 = Less?(x=w1154, y=11 ("x")) -> (x < y?=w1157:bool)
              n552 = And(x=w1157, y=w1156) -> (x .and. y?=w1155:bool)
              n553 = case shown="True" w1155 {
                tunnel: w1160 -> [_ w1168]
                tunnel: w1159 -> [_ w1165]
                tunnel: w1154 -> [_ w1164]
                frame False {
                }
                frame True {
                  n554 = Subtract(x=w1164, y=2) -> (x-y=w1162:i32)
                  n555 = Index Array(array=w1165, index=w1162) -> (element=w1161:i32)
                  n556 = Equal?(x=38, y=w1161) -> (x = y?=w1166:bool)
                  n557 = case shown="True" w1166 {
                    tunnel: w1168 -> [w1169 w1171]
                    frame False {
                      n558 = property class="Page"(reference=w1169, "Page Visible"=FALSE) -> ()  [unwired: 1 in, 2 out]
                    }
                    frame True {
                      n559 = property class="Page"(reference=w1171, "Page Visible"=TRUE) -> ()  [unwired: 1 in, 2 out]
                    }
                  }
                }
              }
            }
            n560 = Index Array(array=w1095, index #1=11 ("index"), index #2=1 ("index")) -> (element #1=w1100:refnum<vi>, element #2=w1093:refnum<vi>)
            n561 = property on="Number of Set points" class="DigNum (strict)"() -> ("NumText.Text"=w1097:string)  [unwired: 2 in, 2 out]
            n562 = property class="Page"(reference=w1100, "Page Visible"=w1092) -> ()  [unwired: 1 in, 2 out]
            n563 = property class="Page"(reference=w1093, "Page Visible"=w1092) -> ()  [unwired: 1 in, 2 out]
            n564 = Decimal String To Number(string=w1097) -> (number=w1089:i32)  [unwired: 2 in, 1 out]
            n565 = for {
              N: 9 -> [_]
              tunnel: w1089 -> [w1112]
              i -> [w1110]
              n566 = Initialize Array(0, w1112, 2 ("dimension size")) -> (w1111:i32[][])
              n567 = Initialize Array(0, w1112, 3 ("dimension size")) -> (w1117:i32[][])
              n568 = for {
                N: w1112 -> [_]
                shift-right: [w1151] -> w1108
                shift-left: w1117 -> [w1152]
                shift-right: [w1142] -> w1107
                shift-left: w1111 -> [w1143]
                i -> [w1140]
                w1144 = 0 ("disabled index (col)")
                w1146 = 0 ("disabled index (col)")
                n569 = Increment(x=w1140) -> (x+1=w1145:i32)
                n570 = Increment(x=w1140) -> (x+1=w1147:i32)
                n571 = Replace Array Subset(array=i32[][] [[0, 0]], new element=w1145, index (row)=w1144, index (col)=w1144) -> (w1138:i32[][])
                n572 = Replace Array Subset(array=i32[][] [[0, 0, 0]], new element=w1147, index (row)=w1146, index (col)=w1146) -> (w1150:i32[][])
                n573 = Index Array(array=w1138, index (row)=w1144) -> (element=w1141:i32[])  [unwired: 1 in]
                n574 = Index Array(array=w1150, index (row)=w1146) -> (element=w1149:i32[])  [unwired: 1 in]
                n575 = Replace Array Subset(array=w1143, new element=w1141, index (row)=w1140) -> (w1142:i32[][])  [unwired: 1 in]
                n576 = Replace Array Subset(array=w1152, new element=w1149, index (row)=w1140) -> (w1151:i32[][])  [unwired: 1 in]
              }
              n577 = To Double Precision Float(number=w1107) -> (double precision float=w1106:dbl[][])
              n578 = To Double Precision Float(number=w1108) -> (double precision float=w1109:dbl[][])
              n579 = case shown="0, Default" w1110 {
                tunnel: w1109 -> [w1119 _ _ _ _ _ _ _ _]
                tunnel: w1106 -> [w1118 w1122 w1124 w1126 w1128 w1130 w1132 w1134 w1136]
                frame 0, Default {
                  n580 = control-ref of="Temperature Goal"() -> (w1121:refnum<vi>)
                  n581 = control-ref of="RampSoakTimes"() -> (w1120:refnum<vi>)
                  n582 = property class="Arr (strict)"(reference=w1121, "Value"=w1118) -> ()  [unwired: 1 in, 2 out]
                  n583 = property class="Arr (strict)"(reference=w1120, "Value"=w1119) -> ()  [unwired: 1 in, 2 out]
                }
                frame 1 {
                  n584 = control-ref of="Temperature Goal"() -> (w1123:refnum<vi>)
                  n585 = property class="Arr (strict)"(reference=w1123, "Value"=w1122) -> ()  [unwired: 1 in, 2 out]
                }
                frame 2 {
                  n586 = control-ref of="Temperature Goal"() -> (w1125:refnum<vi>)
                  n587 = property class="Arr (strict)"(reference=w1125, "Value"=w1124) -> ()  [unwired: 1 in, 2 out]
                }
                frame 3 {
                  n588 = control-ref of="Temperature Goal"() -> (w1127:refnum<vi>)
                  n589 = property class="Arr (strict)"(reference=w1127, "Value"=w1126) -> ()  [unwired: 1 in, 2 out]
                }
                frame 4 {
                  n590 = control-ref of="Temperature Goal"() -> (w1129:refnum<vi>)
                  n591 = property class="Arr (strict)"(reference=w1129, "Value"=w1128) -> ()  [unwired: 1 in, 2 out]
                }
                frame 5 {
                  n592 = control-ref of="Temperature Goal"() -> (w1131:refnum<vi>)
                  n593 = property class="Arr (strict)"(reference=w1131, "Value"=w1130) -> ()  [unwired: 1 in, 2 out]
                }
                frame 6 {
                  n594 = control-ref of="Temperature Goal"() -> (w1133:refnum<vi>)
                  n595 = property class="Arr (strict)"(reference=w1133, "Value"=w1132) -> ()  [unwired: 1 in, 2 out]
                }
                frame 7 {
                  n596 = control-ref of="Temperature Goal"() -> (w1135:refnum<vi>)
                  n597 = property class="Arr (strict)"(reference=w1135, "Value"=w1134) -> ()  [unwired: 1 in, 2 out]
                }
                frame 8 {
                  n598 = control-ref of="Temperature Goal"() -> (w1137:refnum<vi>)
                  n599 = property class="Arr (strict)"(reference=w1137, "Value"=w1136) -> ()  [unwired: 1 in, 2 out]
                }
              }
            }
          }
          event "Import Profile": Value Change {
            w1191 = TRUE ("Page Visible")
            n600 = event-data() -> ("CtlRef"=w1177:refnum<vi>, "OldVal"=w1178:bool)  [unwired: 1 in, 4 out]
            n601 = local read "Path"() -> (w1183:path)
            n602 = control-ref of="CreateTProfile"() -> (w1201:refnum<vi>)
            n603 = control-ref of="Zone Selection"() -> (w1200:refnum<vi>)
            n604 = property on="Property Node" class="TabCtl (strict)"(reference=w1201) -> ("Pages"=w1194:refnum<vi>[])  [unwired: 1 in, 2 out]
            n605 = property class="Bool (strict)"(reference=w1177, "Value"=w1178) -> ()  [unwired: 1 in, 2 out]
            n606 = property on="Property Node" class="LstBox (strict)"(reference=w1200) -> ("Item Symbols"=w1199:i32[])  [unwired: 1 in, 2 out]
            n607 = call-poly <vilib>:"Read Delimited Spreadsheet.vi"("file path (dialog if empty)"=w1183, "delimiter (\\t)"="," ("delimiter (\\t)")) -> ("all rows"=w1184:string[][])  [unwired: 8 in, 5 out]
            n608 = Array Size(array=w1184) -> (size(s)=w1189:i32[])
            n609 = Index Array(array=w1189, index=0) -> (element=w1187:i32)
            n610 = Subtract(x=w1187, y=7) -> (x-y=w1185:i32)
            n611 = To Double Precision Float(number=w1185) -> (double precision float=w1182:dbl)
            n612 = Unbundle By Name(w1176) -> ("ZonesSelected"=w1173:bool[])
            n613 = for {
              N: 13 -> [_]
              tunnel: w1199 -> [w1236]
              tunnel: w1194 -> [w1237] mode=indexing
              shift-right: [w1229] -> w1174
              shift-left: w1173 -> [w1228]
              i -> [w1231]
              n614 = Greater?(x=w1231, y=1) -> (0:w1233:bool)
              n615 = Less?(x=w1231, y=11 ("x")) -> (x < y?=w1234:bool)
              n616 = And(x=w1234, y=w1233) -> (x .and. y?=w1232:bool)
              n617 = case shown="True" w1232 {
                tunnel: w1237 -> [_ w1248]
                tunnel: w1236 -> [_ w1245]
                tunnel: w1231 -> [_ w1244]
                tunnel: w1228 -> [w1238 w1241]
                tunnel: [w1238 w1239] -> w1229
                frame False {
                }
                frame True {
                  n618 = Subtract(x=w1244, y=2) -> (x-y=w1240:i32)
                  n619 = Index Array(array=w1245, index=w1240) -> (element=w1242:i32)
                  n620 = Equal?(x=38, y=w1242) -> (x = y?=w1246:bool)
                  n621 = case shown="False" w1246 {
                    tunnel: w1248 -> [w1253 w1258]
                    tunnel: w1241 -> [w1252 w1257]
                    tunnel: w1240 -> [w1250 w1256]
                    tunnel: [w1251 w1254] -> w1239
                    frame False {
                      w1249 = FALSE ("Page Visible")
                      n622 = property class="Page"(reference=w1253, "Page Visible"=w1249) -> ()  [unwired: 1 in, 2 out]
                      n623 = Replace Array Subset(array=w1252, new element=w1249, index=w1250) -> (w1251:bool[])
                    }
                    frame True {
                      w1255 = TRUE ("Page Visible")
                      n624 = property class="Page"(reference=w1258, "Page Visible"=w1255) -> ()  [unwired: 1 in, 2 out]
                      n625 = Replace Array Subset(array=w1257, new element=w1255, index=w1256) -> (w1254:bool[])
                    }
                  }
                }
              }
            }
            n626 = Bundle By Name(cluster=w1176, "ZonesSelected"=w1174) -> (w1175:T10)
            n627 = Index Array(array=w1194, index #1=11 ("index"), index #2=1 ("index")) -> (element #1=w1196:refnum<vi>, element #2=w1192:refnum<vi>)
            n628 = property class="Page"(reference=w1196, "Page Visible"=w1191) -> ()  [unwired: 1 in, 2 out]
            n629 = property class="Page"(reference=w1192, "Page Visible"=w1191) -> ()  [unwired: 1 in, 2 out]
            n630 = for {
              N: 9 -> [_]
              tunnel: w1182 -> [w1207]
              n631 = Initialize Array(0, w1207, 2 ("dimension size")) -> (w1206:i32[][])
              n632 = Initialize Array(0, w1207, 3 ("dimension size")) -> (w1212:i32[][])
              n633 = for {
                N: w1207 -> [_]
                shift-right: [w1226] -> w1203
                shift-left: w1212 -> [w1227]
                shift-right: [w1217] -> w1205
                shift-left: w1206 -> [w1218]
                i -> [w1215]
                w1219 = 0 ("disabled index (col)")
                w1221 = 0 ("disabled index (col)")
                n634 = Increment(x=w1215) -> (x+1=w1220:i32)
                n635 = Increment(x=w1215) -> (x+1=w1222:i32)
                n636 = Replace Array Subset(array=i32[][] [[0]], new element=w1220, index (row)=w1219, index (col)=w1219) -> (w1213:i32[][])
                n637 = Replace Array Subset(array=i32[][] [[0, 0, 0]], new element=w1222, index (row)=w1221, index (col)=w1221) -> (w1225:i32[][])
                n638 = Index Array(array=w1213, index (row)=w1219) -> (element=w1216:i32[])  [unwired: 1 in]
                n639 = Index Array(array=w1225, index (row)=w1221) -> (element=w1224:i32[])  [unwired: 1 in]
                n640 = Replace Array Subset(array=w1218, new element=w1216, index (row)=w1215) -> (w1217:i32[][])  [unwired: 1 in]
                n641 = Replace Array Subset(array=w1227, new element=w1224, index (row)=w1215) -> (w1226:i32[][])  [unwired: 1 in]
              }
              n642 = Number To Decimal String(number=w1205) -> ()  [unwired: 1 in, 1 out]
              n643 = To Double Precision Float(number=w1203) -> (double precision float=w1202:dbl[][])
              n644 = control-ref of="RampSoakTimes"() -> (w1204:refnum<vi>)
              n645 = property class="Arr (strict)"(reference=w1204, "Value"=w1202) -> ()  [unwired: 1 in, 2 out]
            }
            n646 = call-poly "Send Message.vi"("error in (no error)"=w1181, "event"="importProfile") -> ("error out"=w1180:errorcluster)  [unwired: 9 in]
          }
          event "Compile Profile": Mouse Down {
            n647 = event-data() -> ()  [unwired: 1 in, 1 out]
            n648 = control-ref of="Number of Set points"() -> (w1262:refnum<vi>)
            n649 = property class="DigNum (strict)"(reference=w1262) -> ("Value"=w1259:dbl)  [unwired: 1 in, 2 out]
            n650 = Bundle By Name(cluster=w1261, "ZoneSetup.Number of Set points"=w1259) -> (w1260:T10)
            n651 = call-poly "Send Message.vi"("error in (no error)"=w1265, "event"="compileProfile") -> ("error out"=w1264:errorcluster)  [unwired: 9 in]
          }
          event Mouse Down {
            n652 = event-data() -> ("CtlRef"=w1266:refnum<vi>, "Coords"=w1272:T20)  [unwired: 1 in, 6 out]
            n653 = invoke on="Invoke Node" class="LstBox (strict)" method="Point To Row"(reference=w1266, "Point"=w1272) -> ("InBounds"=w1267:bool, "Row"=w1268:i32)  [unwired: 5 in, 5 out]
            n654 = property on="Property Node" class="LstBox (strict)"(reference=w1266) -> ("Item Symbols"=w1271:i32[])  [unwired: 1 in, 2 out]
            n655 = case shown="True" w1267 {
              tunnel: w1266 -> [_ w1274]
              tunnel: w1271 -> [_ w1282]
              tunnel: w1268 -> [_ w1281]
              frame False {
              }
              frame True {
                n656 = Index Array(array=w1282, index=w1281) -> (element=w1284:i32)
                n657 = control-ref of="Thermocouples Selected"() -> (w1273:refnum<vi>)
                n658 = Equal?(x=w1284, y=37) -> (x = y?=w1279:bool)
                n659 = case shown="True" w1279 {
                  tunnel: w1282 -> [w1297 w1311]
                  tunnel: w1281 -> [w1294 w1307]
                  tunnel: [w1296 w1309] -> w1276
                  tunnel: w1273 -> [w1295 w1308]
                  frame False {
                    n660 = Not Equal To 0?(x=w1294) -> (x != 0?=w1293:bool)
                    n661 = case shown="True" w1293 {
                      tunnel: w1294 -> [_ w1305]
                      tunnel: w1295 -> [_ w1304]
                      frame False {
                      }
                      frame True {
                        n662 = property class="Str"(reference=w1304) -> (reference out=w1303:refnum<vi>, "Text.Text"=w1300:string)  [unwired: 1 in, 1 out]
                        n663 = Number To Decimal String(number=w1305) -> (decimal integer string=w1302:string)  [unwired: 1 in]
                        n664 = call <vilib>:"Space Constant.vi"() -> ("String"=w1301:string)
                        n665 = Search and Replace String(input string=w1300, search string=w1302, replace string=w1301) -> (result string=w1299:string)  [unwired: 5 in, 3 out]
                        n666 = property class="Str"(reference=w1303, "Text.Text"=w1299) -> ()  [unwired: 1 in, 2 out]
                      }
                    }
                    n667 = Replace Array Subset(array=w1297, new element=37, index=w1294) -> (w1296:i32[])
                  }
                  frame True {
                    n668 = Not Equal To 0?(x=w1307) -> (x != 0?=w1306:bool)
                    n669 = case shown="False" w1306 {
                      tunnel: w1308 -> [w1312 w1319]
                      tunnel: w1307 -> [_ w1318]
                      frame False {
                        n670 = property class="Str"(reference=w1312, "Text.Text"="") -> ()  [unwired: 1 in, 2 out]
                      }
                      frame True {
                        n671 = property class="Str"(reference=w1319) -> ("Text.Text"=w1317:string)  [unwired: 1 in, 2 out]
                        n672 = Number To Decimal String(number=w1318) -> (decimal integer string=w1314:string)  [unwired: 1 in]
                        n673 = call <vilib>:"Space Constant.vi"() -> ("String"=w1315:string)
                        n674 = Concatenate Strings(w1317, w1315, w1314) -> (w1316:string)
                        n675 = property class="Str"(reference=w1319, "Text.Text"=w1316) -> ()  [unwired: 1 in, 2 out]
                      }
                    }
                    n676 = Replace Array Subset(array=w1311, new element=38, index=w1307) -> (w1309:i32[])
                  }
                }
                n677 = Equal To 0?(x=w1281) -> (x = 0?=w1280:bool)
                n678 = Array Size(array=w1276) -> (size(s)=w1275:i32)
                n679 = And(x=w1279, y=w1280) -> (x .and. y?=w1278:bool)
                n680 = case shown="True" w1278 {
                  tunnel: w1276 -> [w1285 w1288]
                  tunnel: [w1285 w1287] -> w1277
                  tunnel: w1275 -> [_ w1286]
                  frame False {
                  }
                  frame True {
                    n681 = for {
                      N: w1286 -> [_]
                      shift-right: [w1289] -> w1287
                      shift-left: w1288 -> [w1292]
                      i -> [w1291]
                      n682 = Replace Array Subset(array=w1292, new element=37, index=w1291) -> (w1289:i32[])
                    }
                  }
                }
                n683 = property on="Property Node" class="LstBox (strict)"(reference=w1274, "Item Symbols"=w1277) -> ()  [unwired: 1 in, 2 out]
              }
            }
          }
          event Mouse Down {
            n684 = event-data() -> ("CtlRef"=w1320:refnum<vi>, "Coords"=w1326:T20)  [unwired: 1 in, 6 out]
            n685 = invoke on="Invoke Node" class="LstBox (strict)" method="Point To Row"(reference=w1320, "Point"=w1326) -> ("InBounds"=w1321:bool, "Row"=w1322:i32)  [unwired: 5 in, 5 out]
            n686 = property on="Property Node" class="LstBox (strict)"(reference=w1320) -> ("Item Symbols"=w1325:i32[])  [unwired: 1 in, 2 out]
            n687 = case shown="True" w1321 {
              tunnel: w1320 -> [_ w1328]
              tunnel: w1325 -> [_ w1336]
              tunnel: w1322 -> [_ w1335]
              frame False {
              }
              frame True {
                n688 = Index Array(array=w1336, index=w1335) -> (element=w1338:i32)
                n689 = control-ref of="Thermocouples Selected"() -> (w1327:refnum<vi>)
                n690 = Equal?(x=w1338, y=37) -> (x = y?=w1333:bool)
                n691 = case shown="True" w1333 {
                  tunnel: w1336 -> [w1351 w1365]
                  tunnel: w1335 -> [w1348 w1361]
                  tunnel: [w1350 w1363] -> w1330
                  tunnel: w1327 -> [w1349 w1362]
                  frame False {
                    n692 = Not Equal To 0?(x=w1348) -> (x != 0?=w1347:bool)
                    n693 = case shown="True" w1347 {
                      tunnel: w1348 -> [_ w1359]
                      tunnel: w1349 -> [_ w1358]
                      frame False {
                      }
                      frame True {
                        n694 = property class="Str"(reference=w1358) -> (reference out=w1357:refnum<vi>, "Text.Text"=w1354:string)  [unwired: 1 in, 1 out]
                        n695 = Number To Decimal String(number=w1359) -> (decimal integer string=w1356:string)  [unwired: 1 in]
                        n696 = call <vilib>:"Space Constant.vi"() -> ("String"=w1355:string)
                        n697 = Search and Replace String(input string=w1354, search string=w1356, replace string=w1355) -> (result string=w1353:string)  [unwired: 5 in, 3 out]
                        n698 = property class="Str"(reference=w1357, "Text.Text"=w1353) -> ()  [unwired: 1 in, 2 out]
                      }
                    }
                    n699 = Replace Array Subset(array=w1351, new element=37, index=w1348) -> (w1350:i32[])
                  }
                  frame True {
                    n700 = Not Equal To 0?(x=w1361) -> (x != 0?=w1360:bool)
                    n701 = case shown="True" w1360 {
                      tunnel: w1362 -> [w1366 w1373]
                      tunnel: w1361 -> [_ w1372]
                      frame False {
                        n702 = property class="Str"(reference=w1366, "Text.Text"="") -> ()  [unwired: 1 in, 2 out]
                      }
                      frame True {
                        n703 = property class="Str"(reference=w1373) -> ("Text.Text"=w1371:string)  [unwired: 1 in, 2 out]
                        n704 = Number To Decimal String(number=w1372) -> (decimal integer string=w1368:string)  [unwired: 1 in]
                        n705 = call <vilib>:"Space Constant.vi"() -> ("String"=w1369:string)
                        n706 = Concatenate Strings(w1371, w1369, w1368) -> (w1370:string)
                        n707 = property class="Str"(reference=w1373, "Text.Text"=w1370) -> ()  [unwired: 1 in, 2 out]
                      }
                    }
                    n708 = Replace Array Subset(array=w1365, new element=38, index=w1361) -> (w1363:i32[])
                  }
                }
                n709 = Equal To 0?(x=w1335) -> (x = 0?=w1334:bool)
                n710 = Array Size(array=w1330) -> (size(s)=w1329:i32)
                n711 = And(x=w1333, y=w1334) -> (x .and. y?=w1332:bool)
                n712 = case shown="True" w1332 {
                  tunnel: w1330 -> [w1339 w1342]
                  tunnel: [w1339 w1341] -> w1331
                  tunnel: w1329 -> [_ w1340]
                  frame False {
                  }
                  frame True {
                    n713 = for {
                      N: w1340 -> [_]
                      shift-right: [w1343] -> w1341
                      shift-left: w1342 -> [w1346]
                      i -> [w1345]
                      n714 = Replace Array Subset(array=w1346, new element=37, index=w1345) -> (w1343:i32[])
                    }
                  }
                }
                n715 = property on="Property Node" class="LstBox (strict)"(reference=w1328, "Item Symbols"=w1331) -> ()  [unwired: 1 in, 2 out]
              }
            }
          }
          event Mouse Down {
            n716 = event-data() -> ("CtlRef"=w1374:refnum<vi>, "Coords"=w1380:T20)  [unwired: 1 in, 6 out]
            n717 = invoke on="Invoke Node" class="LstBox (strict)" method="Point To Row"(reference=w1374, "Point"=w1380) -> ("InBounds"=w1375:bool, "Row"=w1376:i32)  [unwired: 5 in, 5 out]
            n718 = property on="Property Node" class="LstBox (strict)"(reference=w1374) -> ("Item Symbols"=w1379:i32[])  [unwired: 1 in, 2 out]
            n719 = case shown="True" w1375 {
              tunnel: w1374 -> [_ w1382]
              tunnel: w1379 -> [_ w1390]
              tunnel: w1376 -> [_ w1389]
              frame False {
              }
              frame True {
                n720 = Index Array(array=w1390, index=w1389) -> (element=w1392:i32)
                n721 = control-ref of="Thermocouples Selected"() -> (w1381:refnum<vi>)
                n722 = Equal?(x=w1392, y=37) -> (x = y?=w1387:bool)
                n723 = case shown="True" w1387 {
                  tunnel: w1390 -> [w1405 w1419]
                  tunnel: w1389 -> [w1402 w1415]
                  tunnel: [w1404 w1417] -> w1384
                  tunnel: w1381 -> [w1403 w1416]
                  frame False {
                    n724 = Not Equal To 0?(x=w1402) -> (x != 0?=w1401:bool)
                    n725 = case shown="True" w1401 {
                      tunnel: w1402 -> [_ w1413]
                      tunnel: w1403 -> [_ w1412]
                      frame False {
                      }
                      frame True {
                        n726 = property class="Str"(reference=w1412) -> (reference out=w1411:refnum<vi>, "Text.Text"=w1408:string)  [unwired: 1 in, 1 out]
                        n727 = Number To Decimal String(number=w1413) -> (decimal integer string=w1410:string)  [unwired: 1 in]
                        n728 = call <vilib>:"Space Constant.vi"() -> ("String"=w1409:string)
                        n729 = Search and Replace String(input string=w1408, search string=w1410, replace string=w1409) -> (result string=w1407:string)  [unwired: 5 in, 3 out]
                        n730 = property class="Str"(reference=w1411, "Text.Text"=w1407) -> ()  [unwired: 1 in, 2 out]
                      }
                    }
                    n731 = Replace Array Subset(array=w1405, new element=37, index=w1402) -> (w1404:i32[])
                  }
                  frame True {
                    n732 = Not Equal To 0?(x=w1415) -> (x != 0?=w1414:bool)
                    n733 = case shown="True" w1414 {
                      tunnel: w1416 -> [w1420 w1427]
                      tunnel: w1415 -> [_ w1426]
                      frame False {
                        n734 = property class="Str"(reference=w1420, "Text.Text"="") -> ()  [unwired: 1 in, 2 out]
                      }
                      frame True {
                        n735 = property class="Str"(reference=w1427) -> ("Text.Text"=w1425:string)  [unwired: 1 in, 2 out]
                        n736 = Number To Decimal String(number=w1426) -> (decimal integer string=w1422:string)  [unwired: 1 in]
                        n737 = call <vilib>:"Space Constant.vi"() -> ("String"=w1423:string)
                        n738 = Concatenate Strings(w1425, w1423, w1422) -> (w1424:string)
                        n739 = property class="Str"(reference=w1427, "Text.Text"=w1424) -> ()  [unwired: 1 in, 2 out]
                      }
                    }
                    n740 = Replace Array Subset(array=w1419, new element=38, index=w1415) -> (w1417:i32[])
                  }
                }
                n741 = Equal To 0?(x=w1389) -> (x = 0?=w1388:bool)
                n742 = Array Size(array=w1384) -> (size(s)=w1383:i32)
                n743 = And(x=w1387, y=w1388) -> (x .and. y?=w1386:bool)
                n744 = case shown="True" w1386 {
                  tunnel: w1384 -> [w1393 w1396]
                  tunnel: [w1393 w1395] -> w1385
                  tunnel: w1383 -> [_ w1394]
                  frame False {
                  }
                  frame True {
                    n745 = for {
                      N: w1394 -> [_]
                      shift-right: [w1397] -> w1395
                      shift-left: w1396 -> [w1400]
                      i -> [w1399]
                      n746 = Replace Array Subset(array=w1400, new element=37, index=w1399) -> (w1397:i32[])
                    }
                  }
                }
                n747 = property on="Property Node" class="LstBox (strict)"(reference=w1382, "Item Symbols"=w1385) -> ()  [unwired: 1 in, 2 out]
              }
            }
          }
          event Mouse Down {
            n748 = event-data() -> ("CtlRef"=w1428:refnum<vi>, "Coords"=w1434:T20)  [unwired: 1 in, 6 out]
            n749 = invoke on="Invoke Node" class="LstBox (strict)" method="Point To Row"(reference=w1428, "Point"=w1434) -> ("InBounds"=w1429:bool, "Row"=w1430:i32)  [unwired: 5 in, 5 out]
            n750 = property on="Property Node" class="LstBox (strict)"(reference=w1428) -> ("Item Symbols"=w1433:i32[])  [unwired: 1 in, 2 out]
            n751 = case shown="True" w1429 {
              tunnel: w1428 -> [_ w1436]
              tunnel: w1433 -> [_ w1444]
              tunnel: w1430 -> [_ w1443]
              frame False {
              }
              frame True {
                n752 = Index Array(array=w1444, index=w1443) -> (element=w1446:i32)
                n753 = control-ref of="Thermocouples Selected"() -> (w1435:refnum<vi>)
                n754 = Equal?(x=w1446, y=37) -> (x = y?=w1441:bool)
                n755 = case shown="True" w1441 {
                  tunnel: w1444 -> [w1459 w1473]
                  tunnel: w1443 -> [w1456 w1469]
                  tunnel: [w1458 w1471] -> w1438
                  tunnel: w1435 -> [w1457 w1470]
                  frame False {
                    n756 = Not Equal To 0?(x=w1456) -> (x != 0?=w1455:bool)
                    n757 = case shown="True" w1455 {
                      tunnel: w1456 -> [_ w1467]
                      tunnel: w1457 -> [_ w1466]
                      frame False {
                      }
                      frame True {
                        n758 = property class="Str"(reference=w1466) -> (reference out=w1465:refnum<vi>, "Text.Text"=w1462:string)  [unwired: 1 in, 1 out]
                        n759 = Number To Decimal String(number=w1467) -> (decimal integer string=w1464:string)  [unwired: 1 in]
                        n760 = call <vilib>:"Space Constant.vi"() -> ("String"=w1463:string)
                        n761 = Search and Replace String(input string=w1462, search string=w1464, replace string=w1463) -> (result string=w1461:string)  [unwired: 5 in, 3 out]
                        n762 = property class="Str"(reference=w1465, "Text.Text"=w1461) -> ()  [unwired: 1 in, 2 out]
                      }
                    }
                    n763 = Replace Array Subset(array=w1459, new element=37, index=w1456) -> (w1458:i32[])
                  }
                  frame True {
                    n764 = Not Equal To 0?(x=w1469) -> (x != 0?=w1468:bool)
                    n765 = case shown="True" w1468 {
                      tunnel: w1470 -> [w1474 w1481]
                      tunnel: w1469 -> [_ w1480]
                      frame False {
                        n766 = property class="Str"(reference=w1474, "Text.Text"="") -> ()  [unwired: 1 in, 2 out]
                      }
                      frame True {
                        n767 = property class="Str"(reference=w1481) -> ("Text.Text"=w1479:string)  [unwired: 1 in, 2 out]
                        n768 = Number To Decimal String(number=w1480) -> (decimal integer string=w1476:string)  [unwired: 1 in]
                        n769 = call <vilib>:"Space Constant.vi"() -> ("String"=w1477:string)
                        n770 = Concatenate Strings(w1479, w1477, w1476) -> (w1478:string)
                        n771 = property class="Str"(reference=w1481, "Text.Text"=w1478) -> ()  [unwired: 1 in, 2 out]
                      }
                    }
                    n772 = Replace Array Subset(array=w1473, new element=38, index=w1469) -> (w1471:i32[])
                  }
                }
                n773 = Equal To 0?(x=w1443) -> (x = 0?=w1442:bool)
                n774 = Array Size(array=w1438) -> (size(s)=w1437:i32)
                n775 = And(x=w1441, y=w1442) -> (x .and. y?=w1440:bool)
                n776 = case shown="True" w1440 {
                  tunnel: w1438 -> [w1447 w1450]
                  tunnel: [w1447 w1449] -> w1439
                  tunnel: w1437 -> [_ w1448]
                  frame False {
                  }
                  frame True {
                    n777 = for {
                      N: w1448 -> [_]
                      shift-right: [w1451] -> w1449
                      shift-left: w1450 -> [w1454]
                      i -> [w1453]
                      n778 = Replace Array Subset(array=w1454, new element=37, index=w1453) -> (w1451:i32[])
                    }
                  }
                }
                n779 = property on="Property Node" class="LstBox (strict)"(reference=w1436, "Item Symbols"=w1439) -> ()  [unwired: 1 in, 2 out]
              }
            }
          }
          event Mouse Down {
            n780 = event-data() -> ("CtlRef"=w1482:refnum<vi>, "Coords"=w1488:T20)  [unwired: 1 in, 6 out]
            n781 = invoke on="Invoke Node" class="LstBox (strict)" method="Point To Row"(reference=w1482, "Point"=w1488) -> ("InBounds"=w1483:bool, "Row"=w1484:i32)  [unwired: 5 in, 5 out]
            n782 = property on="Property Node" class="LstBox (strict)"(reference=w1482) -> ("Item Symbols"=w1487:i32[])  [unwired: 1 in, 2 out]
            n783 = case shown="True" w1483 {
              tunnel: w1482 -> [_ w1490]
              tunnel: w1487 -> [_ w1498]
              tunnel: w1484 -> [_ w1497]
              frame False {
              }
              frame True {
                n784 = Index Array(array=w1498, index=w1497) -> (element=w1500:i32)
                n785 = control-ref of="Thermocouples Selected"() -> (w1489:refnum<vi>)
                n786 = Equal?(x=w1500, y=37) -> (x = y?=w1495:bool)
                n787 = case shown="True" w1495 {
                  tunnel: w1498 -> [w1513 w1527]
                  tunnel: w1497 -> [w1510 w1523]
                  tunnel: [w1512 w1525] -> w1492
                  tunnel: w1489 -> [w1511 w1524]
                  frame False {
                    n788 = Not Equal To 0?(x=w1510) -> (x != 0?=w1509:bool)
                    n789 = case shown="True" w1509 {
                      tunnel: w1510 -> [_ w1521]
                      tunnel: w1511 -> [_ w1520]
                      frame False {
                      }
                      frame True {
                        n790 = property class="Str"(reference=w1520) -> (reference out=w1519:refnum<vi>, "Text.Text"=w1516:string)  [unwired: 1 in, 1 out]
                        n791 = Number To Decimal String(number=w1521) -> (decimal integer string=w1518:string)  [unwired: 1 in]
                        n792 = call <vilib>:"Space Constant.vi"() -> ("String"=w1517:string)
                        n793 = Search and Replace String(input string=w1516, search string=w1518, replace string=w1517) -> (result string=w1515:string)  [unwired: 5 in, 3 out]
                        n794 = property class="Str"(reference=w1519, "Text.Text"=w1515) -> ()  [unwired: 1 in, 2 out]
                      }
                    }
                    n795 = Replace Array Subset(array=w1513, new element=37, index=w1510) -> (w1512:i32[])
                  }
                  frame True {
                    n796 = Not Equal To 0?(x=w1523) -> (x != 0?=w1522:bool)
                    n797 = case shown="True" w1522 {
                      tunnel: w1524 -> [w1528 w1535]
                      tunnel: w1523 -> [_ w1534]
                      frame False {
                        n798 = property class="Str"(reference=w1528, "Text.Text"="") -> ()  [unwired: 1 in, 2 out]
                      }
                      frame True {
                        n799 = property class="Str"(reference=w1535) -> ("Text.Text"=w1533:string)  [unwired: 1 in, 2 out]
                        n800 = Number To Decimal String(number=w1534) -> (decimal integer string=w1530:string)  [unwired: 1 in]
                        n801 = call <vilib>:"Space Constant.vi"() -> ("String"=w1531:string)
                        n802 = Concatenate Strings(w1533, w1531, w1530) -> (w1532:string)
                        n803 = property class="Str"(reference=w1535, "Text.Text"=w1532) -> ()  [unwired: 1 in, 2 out]
                      }
                    }
                    n804 = Replace Array Subset(array=w1527, new element=38, index=w1523) -> (w1525:i32[])
                  }
                }
                n805 = Equal To 0?(x=w1497) -> (x = 0?=w1496:bool)
                n806 = Array Size(array=w1492) -> (size(s)=w1491:i32)
                n807 = And(x=w1495, y=w1496) -> (x .and. y?=w1494:bool)
                n808 = case shown="True" w1494 {
                  tunnel: w1492 -> [w1501 w1504]
                  tunnel: [w1501 w1503] -> w1493
                  tunnel: w1491 -> [_ w1502]
                  frame False {
                  }
                  frame True {
                    n809 = for {
                      N: w1502 -> [_]
                      shift-right: [w1505] -> w1503
                      shift-left: w1504 -> [w1508]
                      i -> [w1507]
                      n810 = Replace Array Subset(array=w1508, new element=37, index=w1507) -> (w1505:i32[])
                    }
                  }
                }
                n811 = property on="Property Node" class="LstBox (strict)"(reference=w1490, "Item Symbols"=w1493) -> ()  [unwired: 1 in, 2 out]
              }
            }
          }
          event Mouse Down {
            n812 = event-data() -> ("CtlRef"=w1536:refnum<vi>, "Coords"=w1542:T20)  [unwired: 1 in, 6 out]
            n813 = invoke on="Invoke Node" class="LstBox (strict)" method="Point To Row"(reference=w1536, "Point"=w1542) -> ("InBounds"=w1537:bool, "Row"=w1538:i32)  [unwired: 5 in, 5 out]
            n814 = property on="Property Node" class="LstBox (strict)"(reference=w1536) -> ("Item Symbols"=w1541:i32[])  [unwired: 1 in, 2 out]
            n815 = case shown="True" w1537 {
              tunnel: w1536 -> [_ w1544]
              tunnel: w1541 -> [_ w1552]
              tunnel: w1538 -> [_ w1551]
              frame False {
              }
              frame True {
                n816 = Index Array(array=w1552, index=w1551) -> (element=w1554:i32)
                n817 = control-ref of="Thermocouples Selected"() -> (w1543:refnum<vi>)
                n818 = Equal?(x=w1554, y=37) -> (x = y?=w1549:bool)
                n819 = case shown="True" w1549 {
                  tunnel: w1552 -> [w1567 w1581]
                  tunnel: w1551 -> [w1564 w1577]
                  tunnel: [w1566 w1579] -> w1546
                  tunnel: w1543 -> [w1565 w1578]
                  frame False {
                    n820 = Not Equal To 0?(x=w1564) -> (x != 0?=w1563:bool)
                    n821 = case shown="True" w1563 {
                      tunnel: w1564 -> [_ w1575]
                      tunnel: w1565 -> [_ w1574]
                      frame False {
                      }
                      frame True {
                        n822 = property class="Str"(reference=w1574) -> (reference out=w1573:refnum<vi>, "Text.Text"=w1570:string)  [unwired: 1 in, 1 out]
                        n823 = Number To Decimal String(number=w1575) -> (decimal integer string=w1572:string)  [unwired: 1 in]
                        n824 = call <vilib>:"Space Constant.vi"() -> ("String"=w1571:string)
                        n825 = Search and Replace String(input string=w1570, search string=w1572, replace string=w1571) -> (result string=w1569:string)  [unwired: 5 in, 3 out]
                        n826 = property class="Str"(reference=w1573, "Text.Text"=w1569) -> ()  [unwired: 1 in, 2 out]
                      }
                    }
                    n827 = Replace Array Subset(array=w1567, new element=37, index=w1564) -> (w1566:i32[])
                  }
                  frame True {
                    n828 = Not Equal To 0?(x=w1577) -> (x != 0?=w1576:bool)
                    n829 = case shown="True" w1576 {
                      tunnel: w1578 -> [w1582 w1589]
                      tunnel: w1577 -> [_ w1588]
                      frame False {
                        n830 = property class="Str"(reference=w1582, "Text.Text"="") -> ()  [unwired: 1 in, 2 out]
                      }
                      frame True {
                        n831 = property class="Str"(reference=w1589) -> ("Text.Text"=w1587:string)  [unwired: 1 in, 2 out]
                        n832 = Number To Decimal String(number=w1588) -> (decimal integer string=w1584:string)  [unwired: 1 in]
                        n833 = call <vilib>:"Space Constant.vi"() -> ("String"=w1585:string)
                        n834 = Concatenate Strings(w1587, w1585, w1584) -> (w1586:string)
                        n835 = property class="Str"(reference=w1589, "Text.Text"=w1586) -> ()  [unwired: 1 in, 2 out]
                      }
                    }
                    n836 = Replace Array Subset(array=w1581, new element=38, index=w1577) -> (w1579:i32[])
                  }
                }
                n837 = Equal To 0?(x=w1551) -> (x = 0?=w1550:bool)
                n838 = Array Size(array=w1546) -> (size(s)=w1545:i32)
                n839 = And(x=w1549, y=w1550) -> (x .and. y?=w1548:bool)
                n840 = case shown="True" w1548 {
                  tunnel: w1546 -> [w1555 w1558]
                  tunnel: [w1555 w1557] -> w1547
                  tunnel: w1545 -> [_ w1556]
                  frame False {
                  }
                  frame True {
                    n841 = for {
                      N: w1556 -> [_]
                      shift-right: [w1559] -> w1557
                      shift-left: w1558 -> [w1562]
                      i -> [w1561]
                      n842 = Replace Array Subset(array=w1562, new element=37, index=w1561) -> (w1559:i32[])
                    }
                  }
                }
                n843 = property on="Property Node" class="LstBox (strict)"(reference=w1544, "Item Symbols"=w1547) -> ()  [unwired: 1 in, 2 out]
              }
            }
          }
          event Mouse Down {
            n844 = event-data() -> ("CtlRef"=w1590:refnum<vi>, "Coords"=w1596:T20)  [unwired: 1 in, 6 out]
            n845 = invoke on="Invoke Node" class="LstBox (strict)" method="Point To Row"(reference=w1590, "Point"=w1596) -> ("InBounds"=w1591:bool, "Row"=w1592:i32)  [unwired: 5 in, 5 out]
            n846 = property on="Property Node" class="LstBox (strict)"(reference=w1590) -> ("Item Symbols"=w1595:i32[])  [unwired: 1 in, 2 out]
            n847 = case shown="True" w1591 {
              tunnel: w1590 -> [_ w1598]
              tunnel: w1595 -> [_ w1606]
              tunnel: w1592 -> [_ w1605]
              frame False {
              }
              frame True {
                n848 = Index Array(array=w1606, index=w1605) -> (element=w1608:i32)
                n849 = control-ref of="Thermocouples Selected"() -> (w1597:refnum<vi>)
                n850 = Equal?(x=w1608, y=37) -> (x = y?=w1603:bool)
                n851 = case shown="True" w1603 {
                  tunnel: w1606 -> [w1621 w1635]
                  tunnel: w1605 -> [w1618 w1631]
                  tunnel: [w1620 w1633] -> w1600
                  tunnel: w1597 -> [w1619 w1632]
                  frame False {
                    n852 = Not Equal To 0?(x=w1618) -> (x != 0?=w1617:bool)
                    n853 = case shown="True" w1617 {
                      tunnel: w1618 -> [_ w1629]
                      tunnel: w1619 -> [_ w1628]
                      frame False {
                      }
                      frame True {
                        n854 = property class="Str"(reference=w1628) -> (reference out=w1627:refnum<vi>, "Text.Text"=w1624:string)  [unwired: 1 in, 1 out]
                        n855 = Number To Decimal String(number=w1629) -> (decimal integer string=w1626:string)  [unwired: 1 in]
                        n856 = call <vilib>:"Space Constant.vi"() -> ("String"=w1625:string)
                        n857 = Search and Replace String(input string=w1624, search string=w1626, replace string=w1625) -> (result string=w1623:string)  [unwired: 5 in, 3 out]
                        n858 = property class="Str"(reference=w1627, "Text.Text"=w1623) -> ()  [unwired: 1 in, 2 out]
                      }
                    }
                    n859 = Replace Array Subset(array=w1621, new element=37, index=w1618) -> (w1620:i32[])
                  }
                  frame True {
                    n860 = Not Equal To 0?(x=w1631) -> (x != 0?=w1630:bool)
                    n861 = case shown="True" w1630 {
                      tunnel: w1632 -> [w1636 w1643]
                      tunnel: w1631 -> [_ w1642]
                      frame False {
                        n862 = property class="Str"(reference=w1636, "Text.Text"="") -> ()  [unwired: 1 in, 2 out]
                      }
                      frame True {
                        n863 = property class="Str"(reference=w1643) -> ("Text.Text"=w1641:string)  [unwired: 1 in, 2 out]
                        n864 = Number To Decimal String(number=w1642) -> (decimal integer string=w1638:string)  [unwired: 1 in]
                        n865 = call <vilib>:"Space Constant.vi"() -> ("String"=w1639:string)
                        n866 = Concatenate Strings(w1641, w1639, w1638) -> (w1640:string)
                        n867 = property class="Str"(reference=w1643, "Text.Text"=w1640) -> ()  [unwired: 1 in, 2 out]
                      }
                    }
                    n868 = Replace Array Subset(array=w1635, new element=38, index=w1631) -> (w1633:i32[])
                  }
                }
                n869 = Equal To 0?(x=w1605) -> (x = 0?=w1604:bool)
                n870 = Array Size(array=w1600) -> (size(s)=w1599:i32)
                n871 = And(x=w1603, y=w1604) -> (x .and. y?=w1602:bool)
                n872 = case shown="True" w1602 {
                  tunnel: w1600 -> [w1609 w1612]
                  tunnel: [w1609 w1611] -> w1601
                  tunnel: w1599 -> [_ w1610]
                  frame False {
                  }
                  frame True {
                    n873 = for {
                      N: w1610 -> [_]
                      shift-right: [w1613] -> w1611
                      shift-left: w1612 -> [w1616]
                      i -> [w1615]
                      n874 = Replace Array Subset(array=w1616, new element=37, index=w1615) -> (w1613:i32[])
                    }
                  }
                }
                n875 = property on="Property Node" class="LstBox (strict)"(reference=w1598, "Item Symbols"=w1601) -> ()  [unwired: 1 in, 2 out]
              }
            }
          }
          event Mouse Down {
            n876 = event-data() -> ("CtlRef"=w1644:refnum<vi>, "Coords"=w1650:T20)  [unwired: 1 in, 6 out]
            n877 = invoke on="Invoke Node" class="LstBox (strict)" method="Point To Row"(reference=w1644, "Point"=w1650) -> ("InBounds"=w1645:bool, "Row"=w1646:i32)  [unwired: 5 in, 5 out]
            n878 = property on="Property Node" class="LstBox (strict)"(reference=w1644) -> ("Item Symbols"=w1649:i32[])  [unwired: 1 in, 2 out]
            n879 = case shown="True" w1645 {
              tunnel: w1644 -> [_ w1652]
              tunnel: w1649 -> [_ w1660]
              tunnel: w1646 -> [_ w1659]
              frame False {
              }
              frame True {
                n880 = Index Array(array=w1660, index=w1659) -> (element=w1662:i32)
                n881 = control-ref of="Thermocouples Selected"() -> (w1651:refnum<vi>)
                n882 = Equal?(x=w1662, y=37) -> (x = y?=w1657:bool)
                n883 = case shown="True" w1657 {
                  tunnel: w1660 -> [w1675 w1689]
                  tunnel: w1659 -> [w1672 w1685]
                  tunnel: [w1674 w1687] -> w1654
                  tunnel: w1651 -> [w1673 w1686]
                  frame False {
                    n884 = Not Equal To 0?(x=w1672) -> (x != 0?=w1671:bool)
                    n885 = case shown="True" w1671 {
                      tunnel: w1672 -> [_ w1683]
                      tunnel: w1673 -> [_ w1682]
                      frame False {
                      }
                      frame True {
                        n886 = property class="Str"(reference=w1682) -> (reference out=w1681:refnum<vi>, "Text.Text"=w1678:string)  [unwired: 1 in, 1 out]
                        n887 = Number To Decimal String(number=w1683) -> (decimal integer string=w1680:string)  [unwired: 1 in]
                        n888 = call <vilib>:"Space Constant.vi"() -> ("String"=w1679:string)
                        n889 = Search and Replace String(input string=w1678, search string=w1680, replace string=w1679) -> (result string=w1677:string)  [unwired: 5 in, 3 out]
                        n890 = property class="Str"(reference=w1681, "Text.Text"=w1677) -> ()  [unwired: 1 in, 2 out]
                      }
                    }
                    n891 = Replace Array Subset(array=w1675, new element=37, index=w1672) -> (w1674:i32[])
                  }
                  frame True {
                    n892 = Not Equal To 0?(x=w1685) -> (x != 0?=w1684:bool)
                    n893 = case shown="True" w1684 {
                      tunnel: w1686 -> [w1690 w1697]
                      tunnel: w1685 -> [_ w1696]
                      frame False {
                        n894 = property class="Str"(reference=w1690, "Text.Text"="") -> ()  [unwired: 1 in, 2 out]
                      }
                      frame True {
                        n895 = property class="Str"(reference=w1697) -> ("Text.Text"=w1695:string)  [unwired: 1 in, 2 out]
                        n896 = Number To Decimal String(number=w1696) -> (decimal integer string=w1692:string)  [unwired: 1 in]
                        n897 = call <vilib>:"Space Constant.vi"() -> ("String"=w1693:string)
                        n898 = Concatenate Strings(w1695, w1693, w1692) -> (w1694:string)
                        n899 = property class="Str"(reference=w1697, "Text.Text"=w1694) -> ()  [unwired: 1 in, 2 out]
                      }
                    }
                    n900 = Replace Array Subset(array=w1689, new element=38, index=w1685) -> (w1687:i32[])
                  }
                }
                n901 = Equal To 0?(x=w1659) -> (x = 0?=w1658:bool)
                n902 = Array Size(array=w1654) -> (size(s)=w1653:i32)
                n903 = And(x=w1657, y=w1658) -> (x .and. y?=w1656:bool)
                n904 = case shown="True" w1656 {
                  tunnel: w1654 -> [w1663 w1666]
                  tunnel: [w1663 w1665] -> w1655
                  tunnel: w1653 -> [_ w1664]
                  frame False {
                  }
                  frame True {
                    n905 = for {
                      N: w1664 -> [_]
                      shift-right: [w1667] -> w1665
                      shift-left: w1666 -> [w1670]
                      i -> [w1669]
                      n906 = Replace Array Subset(array=w1670, new element=37, index=w1669) -> (w1667:i32[])
                    }
                  }
                }
                n907 = property on="Property Node" class="LstBox (strict)"(reference=w1652, "Item Symbols"=w1655) -> ()  [unwired: 1 in, 2 out]
              }
            }
          }
          event Mouse Down {
            n908 = event-data() -> ("CtlRef"=w1698:refnum<vi>, "Coords"=w1704:T20)  [unwired: 1 in, 6 out]
            n909 = invoke on="Invoke Node" class="LstBox (strict)" method="Point To Row"(reference=w1698, "Point"=w1704) -> ("InBounds"=w1699:bool, "Row"=w1700:i32)  [unwired: 5 in, 5 out]
            n910 = property on="Property Node" class="LstBox (strict)"(reference=w1698) -> ("Item Symbols"=w1703:i32[])  [unwired: 1 in, 2 out]
            n911 = case shown="True" w1699 {
              tunnel: w1698 -> [_ w1706]
              tunnel: w1703 -> [_ w1714]
              tunnel: w1700 -> [_ w1713]
              frame False {
              }
              frame True {
                n912 = Index Array(array=w1714, index=w1713) -> (element=w1716:i32)
                n913 = control-ref of="Thermocouples Selected"() -> (w1705:refnum<vi>)
                n914 = Equal?(x=w1716, y=37) -> (x = y?=w1711:bool)
                n915 = case shown="True" w1711 {
                  tunnel: w1714 -> [w1729 w1743]
                  tunnel: w1713 -> [w1726 w1739]
                  tunnel: [w1728 w1741] -> w1708
                  tunnel: w1705 -> [w1727 w1740]
                  frame False {
                    n916 = Not Equal To 0?(x=w1726) -> (x != 0?=w1725:bool)
                    n917 = case shown="True" w1725 {
                      tunnel: w1726 -> [_ w1737]
                      tunnel: w1727 -> [_ w1736]
                      frame False {
                      }
                      frame True {
                        n918 = property class="Str"(reference=w1736) -> (reference out=w1735:refnum<vi>, "Text.Text"=w1732:string)  [unwired: 1 in, 1 out]
                        n919 = Number To Decimal String(number=w1737) -> (decimal integer string=w1734:string)  [unwired: 1 in]
                        n920 = call <vilib>:"Space Constant.vi"() -> ("String"=w1733:string)
                        n921 = Search and Replace String(input string=w1732, search string=w1734, replace string=w1733) -> (result string=w1731:string)  [unwired: 5 in, 3 out]
                        n922 = property class="Str"(reference=w1735, "Text.Text"=w1731) -> ()  [unwired: 1 in, 2 out]
                      }
                    }
                    n923 = Replace Array Subset(array=w1729, new element=37, index=w1726) -> (w1728:i32[])
                  }
                  frame True {
                    n924 = Not Equal To 0?(x=w1739) -> (x != 0?=w1738:bool)
                    n925 = case shown="True" w1738 {
                      tunnel: w1740 -> [w1744 w1751]
                      tunnel: w1739 -> [_ w1750]
                      frame False {
                        n926 = property class="Str"(reference=w1744, "Text.Text"="") -> ()  [unwired: 1 in, 2 out]
                      }
                      frame True {
                        n927 = property class="Str"(reference=w1751) -> ("Text.Text"=w1749:string)  [unwired: 1 in, 2 out]
                        n928 = Number To Decimal String(number=w1750) -> (decimal integer string=w1746:string)  [unwired: 1 in]
                        n929 = call <vilib>:"Space Constant.vi"() -> ("String"=w1747:string)
                        n930 = Concatenate Strings(w1749, w1747, w1746) -> (w1748:string)
                        n931 = property class="Str"(reference=w1751, "Text.Text"=w1748) -> ()  [unwired: 1 in, 2 out]
                      }
                    }
                    n932 = Replace Array Subset(array=w1743, new element=38, index=w1739) -> (w1741:i32[])
                  }
                }
                n933 = Equal To 0?(x=w1713) -> (x = 0?=w1712:bool)
                n934 = Array Size(array=w1708) -> (size(s)=w1707:i32)
                n935 = And(x=w1711, y=w1712) -> (x .and. y?=w1710:bool)
                n936 = case shown="True" w1710 {
                  tunnel: w1708 -> [w1717 w1720]
                  tunnel: [w1717 w1719] -> w1709
                  tunnel: w1707 -> [_ w1718]
                  frame False {
                  }
                  frame True {
                    n937 = for {
                      N: w1718 -> [_]
                      shift-right: [w1721] -> w1719
                      shift-left: w1720 -> [w1724]
                      i -> [w1723]
                      n938 = Replace Array Subset(array=w1724, new element=37, index=w1723) -> (w1721:i32[])
                    }
                  }
                }
                n939 = property on="Property Node" class="LstBox (strict)"(reference=w1706, "Item Symbols"=w1709) -> ()  [unwired: 1 in, 2 out]
              }
            }
          }
          event "exit": Value Change {
            n940 = event-data() -> ()  [unwired: 1 in, 1 out]
            n941 = call "Broadcast Message.vi"("error in (no error)"=w1754, "event"="exit") -> ("error out"=w1752:errorcluster)  [unwired: 9 in]
          }
        }
      }
      frame "compileProfile" {
        n942 = control-ref of="Max Allowable Temp"() -> ()  [unwired: 1 out]
        n943 = Unbundle By Name(w1763) -> ("ZonesSelected"=w1764:bool[], "ZoneSetup.Number of Set points"=w1759:dbl)
        n944 = Initialize Array(T13 {"zone"=0, "average"=0, "thermocouples"=[0], "thermalprofiles"=[{"thermalsetpoint"=0, "tempgoal"=0, "ramp"=0, "soakduration"=0}]} ("ThermalProfileCluster.profiles"), 9 ("dimension size")) -> (w1758:T23)
        n945 = for {
          N: 9 -> [_]
          tunnel: w1763 -> [w1777]
          tunnel: w1764 -> [w1776] mode=indexing
          shift-right: [w1774] -> w1762
          shift-left: w1763 -> [w1775]
          tunnel: w1759 -> [w1770]
          shift-right: [w1768] -> w1757
          shift-left: w1758 -> [w1769]
          i -> [w1767]
          w1773 = 0  # zone
          n946 = Add(x=w1773, y=w1767) -> (x+y=w1772:i32)
          n947 = Increment(x=w1772) -> (x+1=w1771:i32)
          n948 = case shown="True" w1776 {
            tunnel: w1777 -> [_ _]
            tunnel: w1767 -> [_ w1793]
            tunnel: w1775 -> [w1779 w1802]
            tunnel: [w1779 w1802] -> w1774
            tunnel: w1771 -> [_ w1803]
            tunnel: w1770 -> [_ w1790]
            tunnel: w1769 -> [w1778 w1796]
            tunnel: [w1778 w1795] -> w1768
            tunnel: w1767 -> [_ w1794]
            frame False {
            }
            frame True {
              n949 = case shown="8" w1793 {
                tunnel: [w1818 w1821 w1824 w1827 w1830 w1833 w1836 w1839 w1842] -> w1786
                tunnel: [w1817 w1820 w1823 w1826 w1829 w1832 w1835 w1838 w1841] -> w1792
                tunnel: [w1816 w1819 w1822 w1825 w1828 w1831 w1834 w1837 w1840] -> w1781
                frame 0, Default {
                  n950 = control-ref of="Zone Thermocouples"() -> (w1818:refnum<vi>)
                  n951 = control-ref of="Temperature Goal"() -> (w1816:refnum<vi>)
                  n952 = control-ref of="Max Allowable Temp"() -> ()  [unwired: 1 out]
                  n953 = control-ref of="Temperature Calculation"() -> (w1817:refnum<vi>)
                  n954 = control-ref of="Min Allowable Temp"() -> ()  [unwired: 1 out]
                }
                frame 1 {
                  n955 = control-ref of="Zone Thermocouples"() -> (w1821:refnum<vi>)
                  n956 = control-ref of="Temperature Goal"() -> (w1819:refnum<vi>)
                  n957 = control-ref of="Max Allowable Temp"() -> ()  [unwired: 1 out]
                  n958 = control-ref of="Temperature Calculation"() -> (w1820:refnum<vi>)
                  n959 = control-ref of="Min Allowable Temp"() -> ()  [unwired: 1 out]
                }
                frame 2 {
                  n960 = control-ref of="Zone Thermocouples"() -> (w1824:refnum<vi>)
                  n961 = control-ref of="Temperature Goal"() -> (w1822:refnum<vi>)
                  n962 = control-ref of="Max Allowable Temp"() -> ()  [unwired: 1 out]
                  n963 = control-ref of="Temperature Calculation"() -> (w1823:refnum<vi>)
                  n964 = control-ref of="Min Allowable Temp"() -> ()  [unwired: 1 out]
                }
                frame 3 {
                  n965 = control-ref of="Zone Thermocouples"() -> (w1827:refnum<vi>)
                  n966 = control-ref of="Temperature Goal"() -> (w1825:refnum<vi>)
                  n967 = control-ref of="Max Allowable Temp"() -> ()  [unwired: 1 out]
                  n968 = control-ref of="Temperature Calculation"() -> (w1826:refnum<vi>)
                  n969 = control-ref of="Min Allowable Temp"() -> ()  [unwired: 1 out]
                }
                frame 4 {
                  n970 = control-ref of="Zone Thermocouples"() -> (w1830:refnum<vi>)
                  n971 = control-ref of="Temperature Goal"() -> (w1828:refnum<vi>)
                  n972 = control-ref of="Max Allowable Temp"() -> ()  [unwired: 1 out]
                  n973 = control-ref of="Temperature Calculation"() -> (w1829:refnum<vi>)
                  n974 = control-ref of="Min Allowable Temp"() -> ()  [unwired: 1 out]
                }
                frame 5 {
                  n975 = control-ref of="Zone Thermocouples"() -> (w1833:refnum<vi>)
                  n976 = control-ref of="Temperature Goal"() -> (w1831:refnum<vi>)
                  n977 = control-ref of="Max Allowable Temp"() -> ()  [unwired: 1 out]
                  n978 = control-ref of="Temperature Calculation"() -> (w1832:refnum<vi>)
                  n979 = control-ref of="Min Allowable Temp"() -> ()  [unwired: 1 out]
                }
                frame 6 {
                  n980 = control-ref of="Zone Thermocouples"() -> (w1836:refnum<vi>)
                  n981 = control-ref of="Temperature Goal"() -> (w1834:refnum<vi>)
                  n982 = control-ref of="Max Allowable Temp"() -> ()  [unwired: 1 out]
                  n983 = control-ref of="Temperature Calculation"() -> (w1835:refnum<vi>)
                  n984 = control-ref of="Min Allowable Temp"() -> ()  [unwired: 1 out]
                }
                frame 7 {
                  n985 = control-ref of="Zone Thermocouples"() -> (w1839:refnum<vi>)
                  n986 = control-ref of="Temperature Goal"() -> (w1837:refnum<vi>)
                  n987 = control-ref of="Max Allowable Temp"() -> ()  [unwired: 1 out]
                  n988 = control-ref of="Temperature Calculation"() -> (w1838:refnum<vi>)
                  n989 = control-ref of="Min Allowable Temp"() -> ()  [unwired: 1 out]
                }
                frame 8 {
                  n990 = control-ref of="Zone Thermocouples"() -> (w1842:refnum<vi>)
                  n991 = control-ref of="Temperature Goal"() -> (w1840:refnum<vi>)
                  n992 = control-ref of="Max Allowable Temp"() -> ()  [unwired: 1 out]
                  n993 = control-ref of="Temperature Calculation"() -> (w1841:refnum<vi>)
                  n994 = control-ref of="Min Allowable Temp"() -> ()  [unwired: 1 out]
                }
              }
              n995 = To Long Integer(number=w1790) -> (32bit integer=w1789:i32)
              n996 = property class="Arr (strict)"(reference=w1781) -> ("Value"=w1782:dbl[][])  [unwired: 1 in, 2 out]
              n997 = Initialize Array(T14 {"thermalsetpoint"=0, "tempgoal"=0, "ramp"=0, "soakduration"=0} ("thermalprofiles"), w1789) -> (w1798:T24)
              n998 = property class="LstBox (strict)"(reference=w1786) -> ("Item Symbols"=w1787:i32[])  [unwired: 1 in, 2 out]
              n999 = control-ref of="RampSoakTimes"() -> (w1783:refnum<vi>)
              n1000 = Array Size(array=w1787) -> (size(s)=w1788:i32)
              n1001 = for {
                N: w1788 -> [_]
                tunnel: w1787 -> [w1811]
                shift-right: [w1807] -> w1784
                shift-left: i32[] [] -> [w1806]
                i -> [w1805]
                n1002 = Index Array(array=w1811, index=w1805) -> (element=w1809:i32)
                n1003 = Equal?(x=w1809, y=38) -> (x = y?=w1810:bool)
                n1004 = case shown="True" w1810 {
                  tunnel: w1805 -> [_ w1815]
                  tunnel: [w1812 w1813] -> w1807
                  tunnel: w1806 -> [w1812 w1814]
                  frame False {
                  }
                  frame True {
                    n1005 = Build Array (concatenate)(w1814, w1815) -> (w1813:i32[])
                  }
                }
              }
              n1006 = property class="Ring (strict)"(reference=w1792) -> ("Value"=w1791:u16)  [unwired: 1 in, 2 out]
              n1007 = property class="Arr (strict)"(reference=w1783) -> ("Value"=w1780:dbl[][])  [unwired: 1 in, 2 out]
              n1008 = for {
                N: w1789 -> [_]
                tunnel: w1782 -> [w1846]
                tunnel: T14 {"thermalsetpoint"=0, "tempgoal"=0, "ramp"=0, "soakduration"=0} ("thermalprofiles") -> [w1859]
                shift-right: [w1857] -> w1800
                shift-left: w1798 -> [w1858]
                tunnel: w1780 -> [w1850]
                i -> [w1853]
                n1009 = Index Array(array=w1846, index (row)=w1853) -> (element=w1845:dbl[])  [unwired: 1 in]
                n1010 = Index Array(array=w1850, index (row)=w1853) -> (element=w1849:dbl[])  [unwired: 1 in]
                n1011 = Index Array(array=w1845, index #1=0 ("index (row)"), index #2=1 ("index (row)")) -> (element #1=w1844:dbl, element #2=w1843:dbl)
                n1012 = Index Array(array=w1849, index #1=1 ("index (row)"), index #2=2 ("index (row)")) -> (element #1=w1848:dbl, element #2=w1847:dbl)
                n1013 = Bundle By Name(cluster=w1859, "thermalsetpoint"=w1844, "tempgoal"=w1843, "ramp"=w1848, "soakduration"=w1847) -> (w1856:T14)
                n1014 = Replace Array Subset(array=w1858, new element=w1856, index=w1853) -> (w1857:T24)
              }
              n1015 = Bundle By Name(cluster=T13 {"zone"=0, "average"=0, "thermocouples"=[], "thermalprofiles"=[]}, "zone"=w1803, "average"=w1791, "thermocouples"=w1784, "thermalprofiles"=w1800) -> (w1797:T13)
              n1016 = Replace Array Subset(array=w1796, new element=w1797, index=w1794) -> (w1795:T23)
            }
          }
        }
        n1017 = Bundle By Name(cluster=w1762, "ThermalProfileCluster.profiles"=w1757) -> (w1761:T10)
      }
      frame "importProfile" {
        n1018 = property on="Path" class="Path"() -> ("Text.Text"=w1877:string)  [unwired: 2 in, 2 out]
        n1019 = Spreadsheet String To Array(delimiter (Tab)="\\", format string="%s", spreadsheet string=w1877, array type (2D Dbl)=string[][] []) -> (array=w1872:string[][])
        n1020 = call-poly <vilib>:"Read Delimited Spreadsheet.vi"("file path (dialog if empty)"="Path", "delimiter (\\t)"="," ("delimiter (\\t)")) -> ("all rows"=w1861:string[][])  [unwired: 8 in, 5 out]
        n1021 = Array Size(array=w1861) -> (size(s)=w1883:i32[])
        n1022 = Index Array(array=w1883, index=0) -> (element=w1881:i32)
        n1023 = Subtract(x=w1881, y=7) -> (x-y=w1862:i32)
        n1024 = Array Size(array=w1872) -> (size(s)=w1871:i32[])
        n1025 = To Double Precision Float(number=w1862) -> (double precision float=w1878:dbl)
        n1026 = Index Array(array=w1871, index=1) -> (element=w1869:i32)
        n1027 = Decrement(x=w1869) -> (x-1=w1868:i32)
        n1028 = Index Array(array=w1872, index (row)=0, index (col)=w1868) -> (element=w1867:string)
        n1029 = Match Pattern(string=w1867, regular expression=".csv") -> (before substring=w1864:string)  [unwired: 1 in, 3 out]
        n1030 = Bundle By Name(cluster=w1863, "tprofilesheet"=w1861) -> (w1889:T10)
        n1031 = local write "tprofilesheet"(w1861) -> ()
        n1032 = Index Array(array=w1861, index (row)=1) -> (element=w1890:string[])  [unwired: 1 in]
        n1033 = Index Array(array=w1861, index (row)=2) -> (element=w1886:string[])  [unwired: 1 in]
        n1034 = Unbundle By Name(w1889) -> ("ZoneSetup.Zone Selection"=w1888:i32[])
        n1035 = for {
          N: 9 -> [_]
          shift-right: [w1914] -> w1887
          shift-left: w1889 -> [w1929]
          tunnel: w1890 -> [w1928] mode=indexing
          shift-right: [w1926] -> w1884
          shift-left: w1888 -> [w1927]
          tunnel: w1886 -> [w1920]
          tunnel: w1862 -> [w1897]
          tunnel: w1861 -> [w1907]
          i -> [w1899]
          n1036 = case shown="0, Default" w1899 {
            selector: w1899 -> [w2013 w2045 w2077 w2109 w2141 w2173 w2205 w2237 w2269]
            tunnel: w1929 -> [w2017 w2049 w2081 w2113 w2145 w2177 w2209 w2241 w2273]
            tunnel: [w2016 w2048 w2080 w2112 w2144 w2176 w2208 w2240 w2272] -> w1915
            tunnel: w1928 -> [w2015 w2047 w2079 w2111 w2143 w2175 w2207 w2239 w2271]
            tunnel: w1927 -> [w2014 w2046 w2078 w2110 w2142 w2174 w2206 w2238 w2270]
            tunnel: [w2012 w2044 w2076 w2108 w2140 w2172 w2204 w2236 w2268] -> w1926
            tunnel: [w2011 w2043 w2075 w2107 w2139 w2171 w2203 w2235 w2267] -> w1916
            tunnel: [w2010 w2042 w2074 w2106 w2138 w2170 w2202 w2234 w2266] -> w1911
            tunnel: [w2007 w2039 w2071 w2103 w2135 w2167 w2199 w2231 w2263] -> w1912
            frame 0, Default {
              n1037 = control-ref of="Thermocouples Selected"() -> (w2007:refnum<vi>)
              n1038 = case shown="\"\", Default" w2015 {
                tunnel: [2 1 0 0] -> w2008
                tunnel: w2014 -> [w2021 w2026 w2031 w2036]
                tunnel: w2013 -> [w2020 w2025 w2030 w2035]
                tunnel: [w2019 w2024 w2029 w2034] -> w2012
                frame "Max" {
                  n1039 = Replace Array Subset(array=w2021, new element=38, index=w2020) -> (w2019:i32[])
                }
                frame "Min" {
                  n1040 = Replace Array Subset(array=w2026, new element=38, index=w2025) -> (w2024:i32[])
                }
                frame "Average" {
                  n1041 = Replace Array Subset(array=w2031, new element=38, index=w2030) -> (w2029:i32[])
                }
                frame "", Default {
                  n1042 = Replace Array Subset(array=w2036, new element=37, index=w2035) -> (w2034:i32[])
                }
              }
              n1043 = property class="Str"(reference=w2007, "Text.Text"="") -> ()  [unwired: 1 in, 2 out]
              n1044 = control-ref of="Zone Thermocouples"() -> (w2010:refnum<vi>)
              n1045 = property class="LstBox (strict)"(reference=w2010) -> ("Item Symbols"=w2011:i32[])  [unwired: 1 in, 2 out]
              n1046 = Bundle By Name(cluster=w2017, "Zone 1.Temperature Calculation"=w2008) -> (w2016:T10)
              n1047 = control-ref of="Temperature Calculation"() -> (w2009:refnum<vi>)
              n1048 = property class="Ring (strict)"(reference=w2009, "Value"=w2008) -> ()  [unwired: 1 in, 2 out]
            }
            frame 1 {
              n1049 = control-ref of="Thermocouples Selected"() -> (w2039:refnum<vi>)
              n1050 = case shown="\"\", Default" w2047 {
                tunnel: [2 1 0 0] -> w2040
                tunnel: w2046 -> [w2053 w2058 w2063 w2068]
                tunnel: w2045 -> [w2052 w2057 w2062 w2067]
                tunnel: [w2051 w2056 w2061 w2066] -> w2044
                frame "Max" {
                  n1051 = Replace Array Subset(array=w2053, new element=38, index=w2052) -> (w2051:i32[])
                }
                frame "Min" {
                  n1052 = Replace Array Subset(array=w2058, new element=38, index=w2057) -> (w2056:i32[])
                }
                frame "Average" {
                  n1053 = Replace Array Subset(array=w2063, new element=38, index=w2062) -> (w2061:i32[])
                }
                frame "", Default {
                  n1054 = Replace Array Subset(array=w2068, new element=37, index=w2067) -> (w2066:i32[])
                }
              }
              n1055 = property class="Str"(reference=w2039, "Text.Text"="") -> ()  [unwired: 1 in, 2 out]
              n1056 = control-ref of="Zone Thermocouples"() -> (w2042:refnum<vi>)
              n1057 = property class="LstBox (strict)"(reference=w2042) -> ("Item Symbols"=w2043:i32[])  [unwired: 1 in, 2 out]
              n1058 = Bundle By Name(cluster=w2049, "Zone 2.Temperature Calculation"=w2040) -> (w2048:T10)
              n1059 = control-ref of="Temperature Calculation"() -> (w2041:refnum<vi>)
              n1060 = property class="Ring (strict)"(reference=w2041, "Value"=w2040) -> ()  [unwired: 1 in, 2 out]
            }
            frame 2 {
              n1061 = control-ref of="Thermocouples Selected"() -> (w2071:refnum<vi>)
              n1062 = case shown="\"\", Default" w2079 {
                tunnel: [2 1 0 0] -> w2072
                tunnel: w2078 -> [w2085 w2090 w2095 w2100]
                tunnel: w2077 -> [w2084 w2089 w2094 w2099]
                tunnel: [w2083 w2088 w2093 w2098] -> w2076
                frame "Max" {
                  n1063 = Replace Array Subset(array=w2085, new element=38, index=w2084) -> (w2083:i32[])
                }
                frame "Min" {
                  n1064 = Replace Array Subset(array=w2090, new element=38, index=w2089) -> (w2088:i32[])
                }
                frame "Average" {
                  n1065 = Replace Array Subset(array=w2095, new element=38, index=w2094) -> (w2093:i32[])
                }
                frame "", Default {
                  n1066 = Replace Array Subset(array=w2100, new element=37, index=w2099) -> (w2098:i32[])
                }
              }
              n1067 = property class="Str"(reference=w2071, "Text.Text"="") -> ()  [unwired: 1 in, 2 out]
              n1068 = control-ref of="Zone Thermocouples"() -> (w2074:refnum<vi>)
              n1069 = property class="LstBox (strict)"(reference=w2074) -> ("Item Symbols"=w2075:i32[])  [unwired: 1 in, 2 out]
              n1070 = Bundle By Name(cluster=w2081, "Zone 3.Temperature Calculation"=w2072) -> (w2080:T10)
              n1071 = control-ref of="Temperature Calculation"() -> (w2073:refnum<vi>)
              n1072 = property class="Ring (strict)"(reference=w2073, "Value"=w2072) -> ()  [unwired: 1 in, 2 out]
            }
            frame 3 {
              n1073 = control-ref of="Thermocouples Selected"() -> (w2103:refnum<vi>)
              n1074 = case shown="\"\", Default" w2111 {
                tunnel: [2 1 0 0] -> w2104
                tunnel: w2110 -> [w2117 w2122 w2127 w2132]
                tunnel: w2109 -> [w2116 w2121 w2126 w2131]
                tunnel: [w2115 w2120 w2125 w2130] -> w2108
                frame "Max" {
                  n1075 = Replace Array Subset(array=w2117, new element=38, index=w2116) -> (w2115:i32[])
                }
                frame "Min" {
                  n1076 = Replace Array Subset(array=w2122, new element=38, index=w2121) -> (w2120:i32[])
                }
                frame "Average" {
                  n1077 = Replace Array Subset(array=w2127, new element=38, index=w2126) -> (w2125:i32[])
                }
                frame "", Default {
                  n1078 = Replace Array Subset(array=w2132, new element=37, index=w2131) -> (w2130:i32[])
                }
              }
              n1079 = property class="Str"(reference=w2103, "Text.Text"="") -> ()  [unwired: 1 in, 2 out]
              n1080 = control-ref of="Zone Thermocouples"() -> (w2106:refnum<vi>)
              n1081 = property class="LstBox (strict)"(reference=w2106) -> ("Item Symbols"=w2107:i32[])  [unwired: 1 in, 2 out]
              n1082 = Bundle By Name(cluster=w2113, "Zone 4.Temperature Calculation"=w2104) -> (w2112:T10)
              n1083 = control-ref of="Temperature Calculation"() -> (w2105:refnum<vi>)
              n1084 = property class="Ring (strict)"(reference=w2105, "Value"=w2104) -> ()  [unwired: 1 in, 2 out]
            }
            frame 4 {
              n1085 = control-ref of="Thermocouples Selected"() -> (w2135:refnum<vi>)
              n1086 = case shown="\"\", Default" w2143 {
                tunnel: [2 1 0 0] -> w2136
                tunnel: w2142 -> [w2149 w2154 w2159 w2164]
                tunnel: w2141 -> [w2148 w2153 w2158 w2163]
                tunnel: [w2147 w2152 w2157 w2162] -> w2140
                frame "Max" {
                  n1087 = Replace Array Subset(array=w2149, new element=38, index=w2148) -> (w2147:i32[])
                }
                frame "Min" {
                  n1088 = Replace Array Subset(array=w2154, new element=38, index=w2153) -> (w2152:i32[])
                }
                frame "Average" {
                  n1089 = Replace Array Subset(array=w2159, new element=38, index=w2158) -> (w2157:i32[])
                }
                frame "", Default {
                  n1090 = Replace Array Subset(array=w2164, new element=37, index=w2163) -> (w2162:i32[])
                }
              }
              n1091 = property class="Str"(reference=w2135, "Text.Text"="") -> ()  [unwired: 1 in, 2 out]
              n1092 = control-ref of="Zone Thermocouples"() -> (w2138:refnum<vi>)
              n1093 = property class="LstBox (strict)"(reference=w2138) -> ("Item Symbols"=w2139:i32[])  [unwired: 1 in, 2 out]
              n1094 = Bundle By Name(cluster=w2145, "Zone 5.Temperature Calculation"=w2136) -> (w2144:T10)
              n1095 = control-ref of="Temperature Calculation"() -> (w2137:refnum<vi>)
              n1096 = property class="Ring (strict)"(reference=w2137, "Value"=w2136) -> ()  [unwired: 1 in, 2 out]
            }
            frame 5 {
              n1097 = control-ref of="Thermocouples Selected"() -> (w2167:refnum<vi>)
              n1098 = case shown="\"\", Default" w2175 {
                tunnel: [2 1 0 0] -> w2168
                tunnel: w2174 -> [w2181 w2186 w2191 w2196]
                tunnel: w2173 -> [w2180 w2185 w2190 w2195]
                tunnel: [w2179 w2184 w2189 w2194] -> w2172
                frame "Max" {
                  n1099 = Replace Array Subset(array=w2181, new element=38, index=w2180) -> (w2179:i32[])
                }
                frame "Min" {
                  n1100 = Replace Array Subset(array=w2186, new element=38, index=w2185) -> (w2184:i32[])
                }
                frame "Average" {
                  n1101 = Replace Array Subset(array=w2191, new element=38, index=w2190) -> (w2189:i32[])
                }
                frame "", Default {
                  n1102 = Replace Array Subset(array=w2196, new element=37, index=w2195) -> (w2194:i32[])
                }
              }
              n1103 = property class="Str"(reference=w2167, "Text.Text"="") -> ()  [unwired: 1 in, 2 out]
              n1104 = control-ref of="Zone Thermocouples"() -> (w2170:refnum<vi>)
              n1105 = property class="LstBox (strict)"(reference=w2170) -> ("Item Symbols"=w2171:i32[])  [unwired: 1 in, 2 out]
              n1106 = Bundle By Name(cluster=w2177, "Zone 6.Temperature Calculation"=w2168) -> (w2176:T10)
              n1107 = control-ref of="Temperature Calculation"() -> (w2169:refnum<vi>)
              n1108 = property class="Ring (strict)"(reference=w2169, "Value"=w2168) -> ()  [unwired: 1 in, 2 out]
            }
            frame 6 {
              n1109 = control-ref of="Thermocouples Selected"() -> (w2199:refnum<vi>)
              n1110 = case shown="\"\", Default" w2207 {
                tunnel: [2 1 0 0] -> w2200
                tunnel: w2206 -> [w2213 w2218 w2223 w2228]
                tunnel: w2205 -> [w2212 w2217 w2222 w2227]
                tunnel: [w2211 w2216 w2221 w2226] -> w2204
                frame "Max" {
                  n1111 = Replace Array Subset(array=w2213, new element=38, index=w2212) -> (w2211:i32[])
                }
                frame "Min" {
                  n1112 = Replace Array Subset(array=w2218, new element=38, index=w2217) -> (w2216:i32[])
                }
                frame "Average" {
                  n1113 = Replace Array Subset(array=w2223, new element=38, index=w2222) -> (w2221:i32[])
                }
                frame "", Default {
                  n1114 = Replace Array Subset(array=w2228, new element=37, index=w2227) -> (w2226:i32[])
                }
              }
              n1115 = property class="Str"(reference=w2199, "Text.Text"="") -> ()  [unwired: 1 in, 2 out]
              n1116 = control-ref of="Zone Thermocouples"() -> (w2202:refnum<vi>)
              n1117 = property class="LstBox (strict)"(reference=w2202) -> ("Item Symbols"=w2203:i32[])  [unwired: 1 in, 2 out]
              n1118 = Bundle By Name(cluster=w2209, "Zone 7.Temperature Calculation"=w2200) -> (w2208:T10)
              n1119 = control-ref of="Temperature Calculation"() -> (w2201:refnum<vi>)
              n1120 = property class="Ring (strict)"(reference=w2201, "Value"=w2200) -> ()  [unwired: 1 in, 2 out]
            }
            frame 7 {
              n1121 = control-ref of="Thermocouples Selected"() -> (w2231:refnum<vi>)
              n1122 = case shown="\"\", Default" w2239 {
                tunnel: [2 1 0 0] -> w2232
                tunnel: w2238 -> [w2245 w2250 w2255 w2260]
                tunnel: w2237 -> [w2244 w2249 w2254 w2259]
                tunnel: [w2243 w2248 w2253 w2258] -> w2236
                frame "Max" {
                  n1123 = Replace Array Subset(array=w2245, new element=38, index=w2244) -> (w2243:i32[])
                }
                frame "Min" {
                  n1124 = Replace Array Subset(array=w2250, new element=38, index=w2249) -> (w2248:i32[])
                }
                frame "Average" {
                  n1125 = Replace Array Subset(array=w2255, new element=38, index=w2254) -> (w2253:i32[])
                }
                frame "", Default {
                  n1126 = Replace Array Subset(array=w2260, new element=37, index=w2259) -> (w2258:i32[])
                }
              }
              n1127 = property class="Str"(reference=w2231, "Text.Text"="") -> ()  [unwired: 1 in, 2 out]
              n1128 = control-ref of="Zone Thermocouples"() -> (w2234:refnum<vi>)
              n1129 = property class="LstBox (strict)"(reference=w2234) -> ("Item Symbols"=w2235:i32[])  [unwired: 1 in, 2 out]
              n1130 = Bundle By Name(cluster=w2241, "Zone 8.Temperature Calculation"=w2232) -> (w2240:T10)
              n1131 = control-ref of="Temperature Calculation"() -> (w2233:refnum<vi>)
              n1132 = property class="Ring (strict)"(reference=w2233, "Value"=w2232) -> ()  [unwired: 1 in, 2 out]
            }
            frame 8 {
              n1133 = control-ref of="Thermocouples Selected"() -> (w2263:refnum<vi>)
              n1134 = case shown="\"\", Default" w2271 {
                tunnel: [2 1 0 0] -> w2264
                tunnel: w2270 -> [w2277 w2282 w2287 w2292]
                tunnel: w2269 -> [w2276 w2281 w2286 w2291]
                tunnel: [w2275 w2280 w2285 w2290] -> w2268
                frame "Max" {
                  n1135 = Replace Array Subset(array=w2277, new element=38, index=w2276) -> (w2275:i32[])
                }
                frame "Min" {
                  n1136 = Replace Array Subset(array=w2282, new element=38, index=w2281) -> (w2280:i32[])
                }
                frame "Average" {
                  n1137 = Replace Array Subset(array=w2287, new element=38, index=w2286) -> (w2285:i32[])
                }
                frame "", Default {
                  n1138 = Replace Array Subset(array=w2292, new element=37, index=w2291) -> (w2290:i32[])
                }
              }
              n1139 = property class="Str"(reference=w2263, "Text.Text"="") -> ()  [unwired: 1 in, 2 out]
              n1140 = control-ref of="Zone Thermocouples"() -> (w2266:refnum<vi>)
              n1141 = property class="LstBox (strict)"(reference=w2266) -> ("Item Symbols"=w2267:i32[])  [unwired: 1 in, 2 out]
              n1142 = Bundle By Name(cluster=w2273, "Zone 9.Temperature Calculation"=w2264) -> (w2272:T10)
              n1143 = control-ref of="Temperature Calculation"() -> (w2265:refnum<vi>)
              n1144 = property class="Ring (strict)"(reference=w2265, "Value"=w2264) -> ()  [unwired: 1 in, 2 out]
            }
          }
          n1145 = Index Array(array=w1920, index=w1899) -> (element=w1923:string)
          n1146 = call <vilib>:"Space Constant.vi"() -> ("String"=w1924:string)
          n1147 = Initialize Array("", w1897, 3 ("dimension size")) -> (w1902:string[][])
          n1148 = Spreadsheet String To Array(delimiter (Tab)=w1924, format string="%d", spreadsheet string=w1923) -> (array=w1925:dbl[][])  [unwired: 1 in]
          n1149 = Initialize Array("", w1897, 2 ("dimension size")) -> (w1910:string[][])
          n1150 = Index Array(array=w1925, index (row)=0) -> (element=w1919:dbl[])  [unwired: 1 in]
          n1151 = To Long Integer(number=w1919) -> (32bit integer=w1917:i32[])
          n1152 = for {
            N: w1897 -> [_]
            tunnel: w1907 -> [w1951]
            shift-right: [w1948] -> w1906
            shift-left: w1910 -> [w1949]
            tunnel: w1899 -> [w1943]
            shift-right: [w1932] -> w1901
            shift-left: w1902 -> [w1933]
            i -> [w1935]
            n1153 = Add(x=3, y=w1943) -> (x+y=w1942:i32)
            n1154 = Add(x=6, y=w1935) -> (x+y=w1941:i32)
            n1155 = Index Array(array=w1951, index (row) #1=w1941, index (col) #1=0 ("disabled index (col)"), index (row) #2=w1941, index (col) #2=w1942, index (row) #3=w1941, index (col) #3=1 ("disabled index (col)"), index (row) #4=w1941, index (col) #4=2 ("disabled index (col)")) -> (element #1=w1938:string, element #2=w1946:string, element #3=w1937:string, element #4=w1936:string)
            n1156 = Build Array(w1938, w1946) -> (w1945:string[])
            n1157 = Build Array(w1938, w1937, w1936) -> (w1934:string[])
            n1158 = Replace Array Subset(array=w1949, new element=w1945, index (row)=w1935) -> (w1948:string[][])  [unwired: 1 in]
            n1159 = Replace Array Subset(array=w1933, new element=w1934, index (row)=w1935) -> (w1932:string[][])  [unwired: 1 in]
          }
          n1160 = Array Size(array=w1917) -> (size(s)=w1918:i32)
          n1161 = for {
            N: w1918 -> [_]
            tunnel: w1917 -> [w1998] mode=indexing
            shift-right: [w2004] -> w1913
            shift-left: w1916 -> [w2005]
            tunnel: w1912 -> [w1997]
            n1162 = property class="Str"(reference=w1997) -> ("Text.Text"=w2002:string)  [unwired: 1 in, 2 out]
            n1163 = Number To Decimal String(number=w1998) -> (decimal integer string=w1999:string)  [unwired: 1 in]
            n1164 = Replace Array Subset(array=w2005, new element=38, index=w1998) -> (w2004:i32[])
            n1165 = call <vilib>:"Space Constant.vi"() -> ("String"=w2000:string)
            n1166 = Concatenate Strings(w2002, w2000, w1999) -> (w2001:string)
            n1167 = property class="Str"(reference=w1997, "Text.Text"=w2001) -> ()  [unwired: 1 in, 2 out]
          }
          n1168 = property class="LstBox (strict)"(reference=w1911, "Item Symbols"=w1913) -> ()  [unwired: 1 in, 2 out]
          n1169 = Fract/Exp String To Number(string=w1901) -> (number=w1898:dbl[][])  [unwired: 3 in, 1 out]
          n1170 = Fract/Exp String To Number(string=w1906) -> (number=w1905:dbl[][])  [unwired: 3 in, 1 out]
          n1171 = case shown="0, Default" w1899 {
            tunnel: w1915 -> [w1956 w1961 w1966 w1971 w1976 w1981 w1986 w1991 w1996]
            tunnel: [w1955 w1960 w1965 w1970 w1975 w1980 w1985 w1990 w1995] -> w1914
            tunnel: w1913 -> [w1954 w1959 w1964 w1969 w1974 w1979 w1984 w1989 w1994]
            tunnel: w1905 -> [w1952 w1957 w1962 w1967 w1972 w1977 w1982 w1987 w1992]
            frame 0, Default {
              n1172 = Bundle By Name(cluster=w1956, "Zone 1.Zone Thermocouples"=w1954) -> (w1955:T10)
              n1173 = control-ref of="Temperature Goal"() -> (w1953:refnum<vi>)
              n1174 = property class="Arr (strict)"(reference=w1953, "Value"=w1952) -> ()  [unwired: 1 in, 2 out]
            }
            frame 1 {
              n1175 = Bundle By Name(cluster=w1961, "Zone 2.Zone Thermocouples"=w1959) -> (w1960:T10)
              n1176 = control-ref of="Temperature Goal"() -> (w1958:refnum<vi>)
              n1177 = property class="Arr (strict)"(reference=w1958, "Value"=w1957) -> ()  [unwired: 1 in, 2 out]
            }
            frame 2 {
              n1178 = Bundle By Name(cluster=w1966, "Zone 3.Zone Thermocouples"=w1964) -> (w1965:T10)
              n1179 = control-ref of="Temperature Goal"() -> (w1963:refnum<vi>)
              n1180 = property class="Arr (strict)"(reference=w1963, "Value"=w1962) -> ()  [unwired: 1 in, 2 out]
            }
            frame 3 {
              n1181 = Bundle By Name(cluster=w1971, "Zone 4.Zone Thermocouples"=w1969) -> (w1970:T10)
              n1182 = control-ref of="Temperature Goal"() -> (w1968:refnum<vi>)
              n1183 = property class="Arr (strict)"(reference=w1968, "Value"=w1967) -> ()  [unwired: 1 in, 2 out]
            }
            frame 4 {
              n1184 = Bundle By Name(cluster=w1976, "Zone 5.Zone Thermocouples"=w1974) -> (w1975:T10)
              n1185 = control-ref of="Temperature Goal"() -> (w1973:refnum<vi>)
              n1186 = property class="Arr (strict)"(reference=w1973, "Value"=w1972) -> ()  [unwired: 1 in, 2 out]
            }
            frame 5 {
              n1187 = Bundle By Name(cluster=w1981, "Zone 6.Zone Thermocouples"=w1979) -> (w1980:T10)
              n1188 = control-ref of="Temperature Goal"() -> (w1978:refnum<vi>)
              n1189 = property class="Arr (strict)"(reference=w1978, "Value"=w1977) -> ()  [unwired: 1 in, 2 out]
            }
            frame 6 {
              n1190 = Bundle By Name(cluster=w1986, "Zone 7.Zone Thermocouples"=w1984) -> (w1985:T10)
              n1191 = control-ref of="Temperature Goal"() -> (w1983:refnum<vi>)
              n1192 = property class="Arr (strict)"(reference=w1983, "Value"=w1982) -> ()  [unwired: 1 in, 2 out]
            }
            frame 7 {
              n1193 = Bundle By Name(cluster=w1991, "Zone 8.Zone Thermocouples"=w1989) -> (w1990:T10)
              n1194 = control-ref of="Temperature Goal"() -> (w1988:refnum<vi>)
              n1195 = property class="Arr (strict)"(reference=w1988, "Value"=w1987) -> ()  [unwired: 1 in, 2 out]
            }
            frame 8 {
              n1196 = Bundle By Name(cluster=w1996, "Zone 9.Zone Thermocouples"=w1994) -> (w1995:T10)
              n1197 = control-ref of="Temperature Goal"() -> (w1993:refnum<vi>)
              n1198 = property class="Arr (strict)"(reference=w1993, "Value"=w1992) -> ()  [unwired: 1 in, 2 out]
            }
          }
          n1199 = Equal To 0?(x=w1899) -> (x = 0?=w1900:bool)
          n1200 = case shown="True" w1900 {
            tunnel: w1898 -> [_ w1930]
            frame False {
            }
            frame True {
              n1201 = control-ref of="RampSoakTimes"() -> (w1931:refnum<vi>)
              n1202 = property class="Arr (strict)"(reference=w1931, "Value"=w1930) -> ()  [unwired: 1 in, 2 out]
            }
          }
        }
        n1203 = control-ref of="Number of Set points"() -> (w1879:refnum<vi>)
        n1204 = control-ref of="Thermal Profile Name"() -> (w1865:refnum<vi>)
        n1205 = control-ref of="Zone Selection"() -> (w1885:refnum<vi>)
        n1206 = Bundle By Name(cluster=w1887, "ZoneSetup.Zone Selection"=w1884, "ZoneSetup.Number of Set points"=w1878, "ZoneSetup.Thermal Profile Name"=w1864) -> (w1860:T10)
        n1207 = property class="Str"(reference=w1865, "Text.Text"=w1864) -> ()  [unwired: 1 in, 2 out]
        n1208 = property class="DigNum (strict)"(reference=w1879, "Value"=w1878) -> ()  [unwired: 1 in, 2 out]
        n1209 = property class="LstBox (strict)"(reference=w1885, "Item Symbols"=w1884) -> ()  [unwired: 1 in, 2 out]
      }
      frame "graphTC" {
        n1210 = property on="Waveform Chart" class="WFChart (strict)"("LegScrollVis"=TRUE ("Legend:Scrollbar Visible")) -> ()  [unwired: 2 in, 2 out]
        n1211 = Unbundle By Name(w2304) -> ("working array"=w2301:bool[], "Thermocouples"=w2302:T3, "TCs"=w2295:T7)
        n1212 = for {
          N: 120 -> [_]
          tunnel: w2295 -> [w2338] mode=indexing
          tunnel: [w2337] -> w2296 mode=indexing
          shift-right: [w2316] -> w2298
          shift-left: w2302 -> [w2323]
          shift-right: [w2315] -> w2303
          shift-left: w2301 -> [w2314]
          i -> [w2313]
          n1213 = Unbundle By Name(w2338) -> ("thermocouple"=w2347:i32, "temp"=w2311:dbl, "alarm"=w2342:i32, "working"=w2341:bool)
          n1214 = Quotient & Remainder(x=w2313, y=4) -> (x-y*floor(x/y)=w2321:i32, floor(x/y)=w2322:i32)
          n1215 = Index Array(array=w2323, index (row)=w2322, index (col)=w2321) -> (element=w2336:T11)
          n1216 = Multiply(x=w2322, y=4) -> (x*y=w2331:i32)
          n1217 = Multiply(x=w2322, y=4) -> (x*y=w2343:i32)
          n1218 = Unbundle By Name(w2336) -> ("Graph On/Off"=w2320:u32)
          n1219 = Add(x=w2331, y=w2321) -> (x+y=w2329:i32)
          n1220 = Add(x=w2343, y=w2321) -> (x+y=w2312:i32)
          n1221 = Replace Array Subset(array=w2314, new element=w2341, index=w2313) -> (w2315:bool[])
          n1222 = To Double Precision Float(number=w2311) -> (double precision float=w2310:dbl)
          n1223 = Get Date/Time In Seconds() -> (seconds since 1Jan1904=w2340:timestamp)
          n1224 = property on="Waveform Chart" class="WFChart (strict)"("Active Plot"=w2312) -> ()  [unwired: 2 in, 2 out]
          n1225 = Index Array(array=w2315, index=w2329) -> (element=w2328:bool)
          n1226 = Bundle By Name("t0"=w2340) -> (w2339:waveform(dbl))  [unwired: 1 in]
          n1227 = Build Array(w2310) -> (w2309:dbl[])
          n1228 = Number To Fractional String(number=w2310, precision (6)=i16 2 ("width (-)")) -> (F-format string=w2326:string)  [unwired: 2 in]
          n1229 = Bundle By Name(cluster=w2339, "Y"=w2309) -> (w2337:waveform(dbl))
          n1230 = case shown="True" w2328 {
            tunnel: w2320 -> [_ w2352]
            tunnel: [u32 12369084 ("y") w2352] -> w2324
            tunnel: w2326 -> [_ w2351]
            tunnel: ["NaN" w2351] -> w2325
            frame False {
            }
            frame True {
            }
          }
          n1231 = case shown="1" w2342 {
            tunnel: ["" "L" "H"] -> w2317
            tunnel: w2342 -> [_ _ _]
            tunnel: [u32 12369084 u32 2812927 u32 16711680] -> w2318
            frame 0, Default {
            }
            frame 1 {
            }
            frame 2 {
            }
          }
          n1232 = Number To Decimal String(number=w2347) -> (decimal integer string=w2348:string)  [unwired: 1 in]
          n1233 = Index Array(array=w2323, index (row)=w2322, index (col)=w2321) -> (element=w2334:T11)
          n1234 = Equal?(x=w2324, y=u32 6618880) -> (x = y?=w2332:bool)
          n1235 = Concatenate Strings("TC " ("string"), w2348) -> (w2319:string)
          n1236 = property on="Waveform Chart" class="WFChart (strict)"("Plot.Plot Name"=w2319) -> ()  [unwired: 2 in, 2 out]
          n1237 = case shown="True" w2332 {
            tunnel: [w2360 w2368] -> w2335
            tunnel: w2334 -> [w2359 w2367]
            tunnel: w2324 -> [w2357 w2366]
            tunnel: w2325 -> [w2358 w2365]
            tunnel: w2319 -> [w2356 w2364]
            tunnel: w2318 -> [w2355 w2363]
            tunnel: w2317 -> [w2354 w2362]
            frame False {
              n1238 = Bundle By Name(cluster=w2359, "Graph On/Off"=w2357, "TC Label"=w2356, "PlotColor"=u32 12369084 ("y"), "Temperature"=w2358, "Alarm Color"=w2355, "Alarm Status"=w2354) -> (w2360:T11)
            }
            frame True {
              n1239 = property on="Waveform Chart" class="WFChart (strict)"() -> ("Plot.Plot Color"=w2361:u32)  [unwired: 2 in, 2 out]
              n1240 = Bundle By Name(cluster=w2367, "Graph On/Off"=w2366, "TC Label"=w2364, "PlotColor"=w2361, "Temperature"=w2365, "Alarm Color"=w2363, "Alarm Status"=w2362) -> (w2368:T11)
            }
          }
          n1241 = Replace Array Subset(array=w2323, new element=w2335, index (row)=w2322, index (col)=w2321) -> (w2316:T3)
        }
        n1242 = local write "Thermocouples"(w2298) -> ()
        n1243 = Bundle By Name(cluster=w2304, "Thermocouples"=w2298, "working array"=w2303) -> (w2299:T10)
        n1244 = Build Array (concatenate)(waveform(dbl) {"t0"=timestamp(0 s since 1904-01-01), "dt"=1.0, "Y"=[]} ("element"), w2296) -> (w2307:waveform(dbl)[])
        n1245 = Delete From Array(array=w2307, index=0) -> (array with subset deleted=→"Waveform Chart":waveform(dbl)[])  [unwired: 1 in, 1 out]
      }
      frame "receiveCompressorTemp" {
        n1246 = Unflatten From JSON(JSON string=w2378, type and defaults=cluster{"CompressorTemp":dbl} {"CompressorTemp"=0.0}) -> (value=w2376:cluster{"CompressorTemp":dbl})  [unwired: 5 in, 1 out]
        n1247 = Unbundle(w2376) -> ("CompressorTemp"=w2375:dbl)
        n1248 = Bundle By Name(cluster=w2380, "Compressor.CompressorTemp"=w2375) -> (w2381:T10)
      }
      frame "receiveMCCData" {
        n1249 = Unflatten From JSON(JSON string=w2383, type and defaults=T15 {"DutyCycle"=0, "Stage1Temp"=0, "CryoPumpReadyState"={"MotorOn"=FALSE, "Ready"=FALSE}, "PurgeValveState"=FALSE, "RegenError"="", "RegenStep"="", "RoughingValveState"=FALSE, "RoughingInterlock"={"RoughingPermission"=FALSE, "RoughingNeeded"=FALSE, "Cryopumprunning"=FALSE}, "Stage2Temp"=0, "Status"={"PumpOn"=FALSE, "RoughOpen"=FALSE, "PurgeOpen"=FALSE, "ThermocoupleGaugeOn"=FALSE, "PowerFailureOccurred"=FALSE}, "TcPressure"=0}) -> (value=w2392:T15)  [unwired: 5 in, 1 out]
        n1250 = Unbundle By Name(w2392) -> ("Stage1Temp"=w2390:i32, "Stage2Temp"=w2389:i32)
        n1251 = To Double Precision Float(number=w2390) -> (double precision float=w2388:dbl)
        n1252 = To Double Precision Float(number=w2389) -> (double precision float=w2387:dbl)
        n1253 = Build Array(w2387) -> (w2386:dbl[])
        n1254 = Build Array(w2388) -> (w2385:dbl[])
        n1255 = Bundle(w2385, w2386) -> (w2382:cluster{dbl[], dbl[]})  [unwired: 1 in]
        n1256 = Bundle By Name(cluster=w2393, "PumpTemps"=w2382) -> (w2394:T10)
      }
      frame "receiveLastError" {
        n1257 = Unflatten From JSON(JSON string=w2414, type and defaults=T16 {"time"=[], "event"=[], "Thermocouple"=[], "details"=[], "actions"=[]}) -> (value=w2401:T16)  [unwired: 5 in, 1 out]
        n1258 = Unbundle By Name(w2401) -> ("time"=w2396:string[], "details"=w2397:string[])  [unwired: 2 out]
        n1259 = Array Size(array=w2396) -> (size(s)=w2395:i32)
        n1260 = Initialize Array("", w2395, 3 ("dimension size")) -> (w2411:string[][])
        n1261 = Initialize Array("", 3 ("dimension size")) -> (w2408:string[])
        n1262 = for {
          N: w2395 -> [_]
          tunnel: w2408 -> [w2424]
          tunnel: [w2422] -> w2406
          shift-right: [w2421] -> w2402
          shift-left: w2411 -> [w2425]
          tunnel: w2397 -> [w2416] mode=indexing
          tunnel: w2396 -> [w2415] mode=indexing
          i -> [w2417]
          n1263 = control-ref of="Current Errors (click to clear)"() -> (w2428:refnum<vi>)
          n1264 = Bundle(w2417, 2) -> (w2426:cluster{i32, i32})  [unwired: 1 in]
          n1265 = property on="Property Node" class="MCListbox (strict)"(reference=w2428, "ActiveCell"=w2426) -> (reference out=w2422:refnum<vi>)  [unwired: 1 in, 1 out]
          n1266 = Replace Array Subset(array=w2424, new element=w2416, index=2) -> (w2420:string[])
          n1267 = Replace Array Subset(array=w2420, new element=w2415, index=1) -> (w2418:string[])
          n1268 = Replace Array Subset(array=w2425, new element=w2418, index (row)=w2417) -> (w2421:string[][])  [unwired: 1 in]
        }
        n1269 = property class="MCListbox (strict)"(reference=w2406, "ItemNames"=w2402) -> ()  [unwired: 1 in, 2 out]
        n1270 = Initialize Array(37, w2395) -> (w2404:i32[])
        n1271 = property class="MCListbox (strict)"(reference=w2406, "ItemSyms"=w2404) -> ()  [unwired: 1 in, 2 out]
        n1272 = local write "errortrue"(FALSE ("Generate Error")) -> ()
        n1273 = Bundle By Name(cluster=w2398, "ErrorArray"=w2402) -> (w2403:T10)
      }
      frame "receivePressure" {
        n1274 = Unflatten From JSON(JSON string=w2429, type and defaults=T17 {"CryoPressure"=0.0, "ChamberPressure"=0.0, "RoughingPressure"=0.0}) -> (value=w2435:T17)  [unwired: 5 in, 1 out]
        n1275 = Unbundle By Name(w2435) -> ("CryoPressure"=w2434:dbl, "ChamberPressure"=w2433:dbl, "RoughingPressure"=w2432:dbl)
        n1276 = Build Array(w2434, w2433, w2432) -> (w2436:dbl[])
        n1277 = Bundle By Name(cluster=w2438, "Pressure"=w2436) -> (w2437:T10)
      }
      frame "receiveTC" {
        n1278 = Unflatten From JSON(JSON string=w2442, type and defaults=T18 {"time"="", "TCs"=[]} ("Cluster")) -> (value=w2445:T18)  [unwired: 5 in, 1 out]
        n1279 = Unbundle By Name(w2445) -> ("TCs"=w2444:T7)
        n1280 = Bundle By Name(cluster=w2443, "TCs"=w2444) -> (w2439:T10)
      }
      frame "receiveZoneTemps" {
        n1281 = Unflatten From JSON(JSON string=w2448, type and defaults=cluster{"ZoneTemps":dbl[]} {"ZoneTemps"=[]}) -> (value=w2446:cluster{"ZoneTemps":dbl[]})  [unwired: 5 in, 1 out]
        n1282 = Bundle By Name(cluster=w2450, "ZoneTemps"=w2446) -> (w2451:T10)
      }
      frame "masterDatabase" {
        n1283 = Unbundle By Name(w2465) -> ("Thermocouples"=w2466:T3, "Pressure"=w2458:dbl[], "PumpTemps"=w2461:T8, "NumberTCs"=w2467:i32, "ZoneTemps"=w2455:cluster{"ZoneTemps":dbl[]}, "Compressor.CompressorTemp"=w2453:dbl)  [unwired: 1 out]
        n1284 = Initialize Array(0.0 ("element"), w2467) -> (w2469:dbl[])
        n1285 = Unbundle(w2461) -> ("Cp Stage 1 Temp"=w2460:dbl[], "Cp Stage 2 Temp"=w2459:dbl[])
        n1286 = Unbundle(w2455) -> ("ZoneTemps"=w2454:dbl[])
        n1287 = Build Array (concatenate)(w2460, w2459) -> (w2457:dbl[])
        n1288 = Build Array(w2453) -> (w2452:dbl[])
        n1289 = for {
          N: w2467 -> [_]
          shift-right: [w2479] -> w2456
          shift-left: w2469 -> [w2480]
          tunnel: w2466 -> [w2475]
          i -> [w2477]
          n1290 = Quotient & Remainder(x=w2477, y=4) -> (x-y*floor(x/y)=w2474:i32, floor(x/y)=w2476:i32)
          n1291 = Index Array(array=w2475, index (row)=w2476, index (col)=w2474) -> (element=w2473:T11)
          n1292 = Unbundle By Name(w2473) -> ("Temperature"=w2472:string)
          n1293 = Fract/Exp String To Number(string=w2472) -> (number=w2471:dbl)  [unwired: 3 in, 1 out]
          n1294 = To Double Precision Float(number=w2471) -> (double precision float=w2481:dbl)
          n1295 = Replace Array Subset(array=w2480, new element=w2481, index=w2477) -> (w2479:dbl[])
        }
        n1296 = Build Array (concatenate)(dbl[] [0.0], w2458, w2454, w2456, w2457, w2452) -> (w2463:dbl[])
        n1297 = Bundle By Name(cluster=w2465, "Database"=w2463) -> (w2464:T10)
      }
      frame "multipleGraphs" {
        n1298 = local read "Custom Graph Selector"() -> (w2482:i32)
        n1299 = for {
          N: 6 ("Numeric") -> [_]
          tunnel: w2485 -> [w2499]
          tunnel: w2484 -> [w2498]
          tunnel: w2482 -> [w2489]
          i -> [w2486]
          n1300 = case shown="1" w2486 {
            tunnel: [w2545 w2546 w2548 w2550 w2552 w2554] -> w2491
            tunnel: [w2544 w2547 w2549 w2551 w2553 w2555] -> w2490
            frame 0, Default {
              n1301 = control-ref of="Custom Chart 1 Selection"() -> (w2544:refnum<vi>)
              n1302 = control-ref of="Custom Chart 1"() -> (w2545:refnum<vi>)
            }
            frame 1 {
              n1303 = control-ref of="Custom Chart 2 Selection"() -> (w2547:refnum<vi>)
              n1304 = control-ref of="Custom Chart 2"() -> (w2546:refnum<vi>)
            }
            frame 2 {
              n1305 = control-ref of="Custom Chart 3 Selection"() -> (w2549:refnum<vi>)
              n1306 = control-ref of="Custom Chart 3"() -> (w2548:refnum<vi>)
            }
            frame 3 {
              n1307 = control-ref of="Custom Chart 4 Selection"() -> (w2551:refnum<vi>)
              n1308 = control-ref of="Custom Chart 4"() -> (w2550:refnum<vi>)
            }
            frame 4 {
              n1309 = control-ref of="Custom Chart 5 Selection"() -> (w2553:refnum<vi>)
              n1310 = control-ref of="Custom Chart 5"() -> (w2552:refnum<vi>)
            }
            frame 5 {
              n1311 = control-ref of="Custom Chart 6 Selection"() -> (w2555:refnum<vi>)
              n1312 = control-ref of="Custom Chart 6"() -> (w2554:refnum<vi>)
            }
          }
          n1313 = Equal?(x=w2489, y=w2486) -> (x = y?=w2487:bool)
          n1314 = Unbundle By Name(w2498) -> ("Database"=w2496:dbl[], "numSensors"=w2497:i32)
          n1315 = case shown="True" w2487 {
            tunnel: w2499 -> [_ w2513]
            tunnel: [w2502 w2507] -> w2495
            tunnel: [1000 w2506] -> w2494
            tunnel: w2490 -> [w2503 w2505]
            tunnel: [FALSE w2504] -> w2488
            frame False {
              n1316 = property on="Property Node" class="LstBox (strict)"(reference=w2503) -> ("Item Symbols"=w2502:i32[])  [unwired: 1 in, 2 out]
            }
            frame True {
              n1317 = property on="Property Node" class="LstBox (strict)"(reference=w2505) -> ("Item Symbols"=w2507:i32[])  [unwired: 1 in, 2 out]
              n1318 = Decimal String To Number(string=w2513) -> (number=w2506:i32)  [unwired: 2 in, 1 out]
              n1319 = Index Array(array=w2507, index=0) -> (element=w2508:i32)
              n1320 = Equal?(x=37, y=w2508) -> (x = y?=w2510:bool)
              n1321 = Equal To 0?(x=w2506) -> (x = 0?=w2512:bool)
              n1322 = And(x=w2510, y=w2512) -> (x .and. y?=w2504:bool)
            }
          }
          n1323 = case shown="False" w2488 {
            tunnel: [0 ("index") w2608] -> w2493
            tunnel: w2497 -> [w2562 w2604]
            tunnel: w2496 -> [w2561 _]
            tunnel: [w2560 _] -> w2492
            tunnel: w2494 -> [w2558 w2608]
            tunnel: w2495 -> [w2559 w2607]
            tunnel: w2490 -> [w2557 w2603]
            tunnel: w2491 -> [w2556 w2602]
            frame False {
              n1324 = for {
                N: w2562 -> [_]
                tunnel: [w2581] -> w2560 mode=indexing
                tunnel: w2558 -> [w2575]
                tunnel: w2559 -> [w2570]
                tunnel: w2561 -> [w2567] mode=indexing
                tunnel: w2557 -> [w2565]
                tunnel: w2556 -> [w2564]
                i -> [w2568]
                n1325 = Wait (ms)(milliseconds to wait=u32 0) -> ()  [unwired: 1 out]
                n1326 = Get Date/Time In Seconds() -> (seconds since 1Jan1904=w2583:timestamp)
                n1327 = Bundle By Name("t0"=w2583) -> (w2582:waveform(dbl))  [unwired: 1 in]
                n1328 = Build Array(w2567) -> (w2566:dbl[])
                n1329 = Bundle By Name(cluster=w2582, "Y"=w2566) -> (w2581:waveform(dbl))
                n1330 = Index Array(array=w2570, index=w2575) -> (element=w2573:i32)
                n1331 = Index Array(array=w2570, index=w2575) -> (element=w2576:i32)
                n1332 = Equal?(x=w2573, y=38) -> (x = y?=w2572:bool)
                n1333 = Equal?(x=w2576, y=37) -> (x = y?=w2578:bool)
                n1334 = Equal?(x=w2568, y=w2575) -> (x = y?=w2571:bool)
                n1335 = And(x=w2571, y=w2572) -> (x .and. y?=w2569:bool)
                n1336 = And(x=w2571, y=w2578) -> (x .and. y?=w2577:bool)
                n1337 = case shown="True" w2577 {
                  tunnel: w2570 -> [_ w2601]
                  tunnel: w2575 -> [_ _]
                  tunnel: w2568 -> [_ w2596]
                  tunnel: w2564 -> [_ w2595]
                  tunnel: w2565 -> [_ w2594]
                  frame False {
                  }
                  frame True {
                    n1338 = property on="Property Node" class="WFChart (strict)"(reference=w2595, "Active Plot"=w2596) -> (reference out=w2599:refnum<vi>)  [unwired: 1 in, 1 out]
                    n1339 = Replace Array Subset(array=w2601, new element=38, index=w2596) -> (w2597:i32[])
                    n1340 = property on="Property Node" class="WFChart (strict)"(reference=w2595) -> ("Plot.Plot Color"=w2593:u32)  [unwired: 1 in, 2 out]
                    n1341 = property on="Property Node" class="WFChart (strict)"(reference=w2599, "Plot.Visible?"=TRUE ("Plot.Visible")) -> ()  [unwired: 1 in, 2 out]
                    n1342 = property on="Property Node" class="LstBox (strict)"(reference=w2594, "Active Row"=w2596) -> ()  [unwired: 1 in, 2 out]
                    n1343 = property on="Property Node" class="LstBox (strict)"(reference=w2594, "CellBG"=w2593) -> ()  [unwired: 1 in, 2 out]
                    n1344 = property on="Property Node" class="LstBox (strict)"(reference=w2594, "Item Symbols"=w2597) -> ()  [unwired: 1 in, 2 out]
                  }
                }
                n1345 = case shown="True" w2569 {
                  tunnel: w2570 -> [_ w2592]
                  tunnel: w2568 -> [_ w2585]
                  tunnel: w2564 -> [_ w2586]
                  tunnel: w2565 -> [_ w2587]
                  frame False {
                  }
                  frame True {
                    n1346 = property on="Property Node" class="WFChart (strict)"(reference=w2586, "Active Plot"=w2585) -> (reference out=w2590:refnum<vi>)  [unwired: 1 in, 1 out]
                    n1347 = Replace Array Subset(array=w2592, new element=37, index=w2585) -> (w2588:i32[])
                    n1348 = property on="Property Node" class="WFChart (strict)"(reference=w2590, "Plot.Visible?"=FALSE ("Plot.Visible")) -> ()  [unwired: 1 in, 2 out]
                    n1349 = property on="Property Node" class="LstBox (strict)"(reference=w2587, "Active Row"=w2585) -> ()  [unwired: 1 in, 2 out]
                    n1350 = property on="Property Node" class="LstBox (strict)"(reference=w2587, "CellBG"=u32 13816530 ("Active Row:Cell Background Color")) -> ()  [unwired: 1 in, 2 out]
                    n1351 = property on="Property Node" class="LstBox (strict)"(reference=w2587, "Item Symbols"=w2588) -> ()  [unwired: 1 in, 2 out]
                  }
                }
              }
            }
            frame True {
              n1352 = for {
                N: w2604 -> [_]
                tunnel: w2607 -> [_]
                tunnel: w2603 -> [w2610]
                tunnel: w2602 -> [w2609]
                i -> [w2611]
                n1353 = property on="Property Node" class="WFChart (strict)"(reference=w2609, "Active Plot"=w2611) -> (reference out=w2614:refnum<vi>)  [unwired: 1 in, 1 out]
                n1354 = property on="Property Node" class="WFChart (strict)"(reference=w2614, "Plot.Visible?"=FALSE ("Plot.Visible")) -> ()  [unwired: 1 in, 2 out]
                n1355 = property on="Property Node" class="LstBox (strict)"(reference=w2610, "Active Row"=w2611) -> ()  [unwired: 1 in, 2 out]
                n1356 = property on="Property Node" class="LstBox (strict)"(reference=w2610, "CellBG"=u32 13816530 ("Active Row:Cell Background Color")) -> ()  [unwired: 1 in, 2 out]
              }
              n1357 = Initialize Array(37, w2604) -> (w2605:i32[])
              n1358 = property on="Property Node" class="LstBox (strict)"(reference=w2603, "Item Symbols"=w2605) -> ()  [unwired: 1 in, 2 out]
            }
          }
          n1359 = case shown="4" w2486 {
            tunnel: w2493 -> [w2515 w2520 w2525 w2530 w2535 w2540]
            tunnel: w2492 -> [w2514 w2519 w2524 w2529 w2534 w2539]
            frame 0, Default {
              n1360 = Build Array (concatenate)(waveform(dbl) {"t0"=timestamp(0 s since 1904-01-01), "dt"=1.0, "Y"=[]} ("element"), w2514) -> (w2518:waveform(dbl)[])
              n1361 = Delete From Array(array=w2518, index=w2515) -> (array with subset deleted=→"Custom Chart 1":waveform(dbl)[])  [unwired: 1 in, 1 out]
            }
            frame 1 {
              n1362 = Build Array (concatenate)(waveform(dbl) {"t0"=timestamp(0 s since 1904-01-01), "dt"=1.0, "Y"=[]} ("element"), w2519) -> (w2523:waveform(dbl)[])
              n1363 = Delete From Array(array=w2523, index=w2520) -> (array with subset deleted=→"Custom Chart 2":waveform(dbl)[])  [unwired: 1 in, 1 out]
            }
            frame 2 {
              n1364 = Build Array (concatenate)(waveform(dbl) {"t0"=timestamp(0 s since 1904-01-01), "dt"=1.0, "Y"=[]} ("element"), w2524) -> (w2528:waveform(dbl)[])
              n1365 = Delete From Array(array=w2528, index=w2525) -> (array with subset deleted=→"Custom Chart 3":waveform(dbl)[])  [unwired: 1 in, 1 out]
            }
            frame 3 {
              n1366 = Build Array (concatenate)(waveform(dbl) {"t0"=timestamp(0 s since 1904-01-01), "dt"=1.0, "Y"=[]} ("element"), w2529) -> (w2533:waveform(dbl)[])
              n1367 = Delete From Array(array=w2533, index=w2530) -> (array with subset deleted=→"Custom Chart 4":waveform(dbl)[])  [unwired: 1 in, 1 out]
            }
            frame 4 {
              n1368 = Build Array (concatenate)(waveform(dbl) {"t0"=timestamp(0 s since 1904-01-01), "dt"=1.0, "Y"=[]} ("element"), w2534) -> (w2538:waveform(dbl)[])
              n1369 = Delete From Array(array=w2538, index=w2535) -> (array with subset deleted=→"Custom Chart 5":waveform(dbl)[])  [unwired: 1 in, 1 out]
            }
            frame 5 {
              n1370 = Build Array (concatenate)(waveform(dbl) {"t0"=timestamp(0 s since 1904-01-01), "dt"=1.0, "Y"=[]} ("element"), w2539) -> (w2543:waveform(dbl)[])
              n1371 = Delete From Array(array=w2543, index=w2540) -> (array with subset deleted=→"Custom Chart 6":waveform(dbl)[])  [unwired: 1 in, 1 out]
            }
          }
        }
      }
      frame "exit" {
        n1372 = Unbundle By Name(w2616) -> ("Http session"=w2617:T9)
        n1373 = call <vilib>:"CloseHandle.vi"("client handle"=w2617, "error in (no error)"=w2619) -> ("error out"=w2618:errorcluster)  [unwired: 13 in]
        n1374 = Bundle By Name(cluster=w2616, "go"=FALSE ("Bundle Element")) -> (w2620:T10)
      }
      frame Default {
        n1375 = call "Unknown Message Dialog.vi"("error in (no error)"=w2623, "event name"=w2622) -> ("error out"=w2621:errorcluster)  [unwired: 9 in]
      }
    }
    n1376 = Unbundle By Name(w49) -> ("go"=w48:bool)
    n1377 = call "log system event.vi"("error in (no error)"=w51) -> ("error out"=w50:errorcluster)  [unwired: 9 in, 1 out]
  }
  n1378 = local read "Local Debug"() -> (w16:bool)
  n1379 = call "getData.vi"("Local Debug"=w16) -> ()  [unwired: 11 in]
  n1380 = call "Unload Module.vi"("error in (no error)"=w28) -> ()  [unwired: 10 in, 1 out]
  n1381 = property on="Waveform Chart" class="WFChart (strict)" props=["Plot", "Visible?"]() -> ()  [unwired: 2 in, 3 out]
